vi "OP_Print_TPS_cluster_20180209_v2013last.vi"() -> ()   [LabVIEW 2017]
uses:
  <vilib>/addons/database/Connection.llb/DB Tools Open Connec (Path).vi
  <vilib>/addons/database/Connection.llb/Conn Execute.vi
  <vilib>/addons/database/Recordset.llb/Rec Fetch Recordset Data (R).vi
  <vilib>/addons/database/Recordset.llb/Rec Destroy - Connection.vi
  <userlib>/caLab/Private/Get_PV-1D.vi
  <userlib>/caLab/Private/Get_PV.vi
  <vilib>/Utility/file.llb/Write To Spreadsheet File (string).vi
  <vilib>/addons/database/NI_Database_API.lvlib
panel:
  out "error out 2":errorcluster
  in  "WindowsMediaPlayer":refnum<k7>(container)
  in  "Vol.":i32(slide)=12 min=0 max=100 step=1 scale=0.0..100.0
  out "index":i32
  in  "Play Button":bool
  in  "Skip Forward Button":bool
  in  "Skip Back Button":bool
  in  "Pause Button":bool
  out "appended path":path=path "C:/Users/TPSOP/Desktop/新增資料夾 (2)/musics/1.mp3"
  out "status":string="就緒"
  out "error out":errorcluster
  out "new picture":picture
  in  "T:Slow\nF:Fast":bool
  in  "Switch Tab":bool=TRUE
  out "Tab Control":enum32{"_____", "           "}(tab)
  out "Cluster":T1={"SR Fill Pattern"=[], "Beam Current(mA"=320.769453, "Beam Lifetime(min)"=354.3939151043138, "Beamsize X(um)"=63.15189373514937, "Beamsize Y(um)"=38.03691397287648, "Tune X(from BPM)"=0.1487279843444227, "Tune Y(from BPM)"=0.2309197651663405, "Mode"="Top-Up", "NuX(from BBF) "=0.15142063757609414, "NuY(from BBF)"=0.22496346361412184, "IU22-23gap(R)"=7.0, "IU22-05gap(R)"=7.372, "IU22-05M"=TRUE, "IU22A-09gap(R)"=8.05, "IU22A-09M"=TRUE, "IU22B-09gap(R)"=40.001, "IU22B-09M"=FALSE, "IUT22-21gap(R)"=7.0, "IUT22-21M"=TRUE, "IU22-23M"=TRUE, "IU22A-25gap(R)"=7.0, "IU22A-25M"=TRUE, "IU22B-25gap(R)"=40.0, "IU22B-25M"=FALSE, "EPU48A-41gap(R)"=65.00055, "EPU48A-41gM"=FALSE, "EPU48B-41gap(R)"=27.450000000000003, "EPU48B-41gM"=TRUE, "EPU46-45gap(R)"=44.99850000000001, "EPU46-45gM"=FALSE, "EPU48A-41phase(R)"=0.00055, "EPU48B-41phase(R)"=0.0, "EPU46-45phase(R)"=5e-05, "Grid volt.(V)[S]"=33.0, "Gun mode"="MBM", "Mod.3 HV(kV)[S]"=35.37999999999996, "SR"="SR_DMB_2017_1024_0300LOCO.data", "BR"="Booster_2017_1023_0900.data", "LI"="Linac_2017_0413_1015.data", "LTB"="LTB_JT_2017_0828_1050.data", "BTS"="BTS_2017_1023_0900.data", "RF2 remote"=TRUE, "RF2 OP mode"=TRUE, "RF2 phase.[S]"=-42.0, "RF Freq.(s)"=499655365.67399085, "RF2 gap volt[S]"=1600.0, "RF3 remote"=TRUE, "RF3 OP mode"=TRUE, "RF3 phase.[S]"=1.1999999999999995, "RF3 gap volt.[S]"=1600.0, "BBF V"=TRUE, "BBF H"=TRUE, "BR ext. kicker1(kV)"=17.666, "BR ext. kicker2(kV)"=17.666, "BR ext. sep.1(V)"=322.14, "BR ext. sep.2(V)"=441.1, "BR inj. sep.(V)"=104.95, "BR inj. kicker(kV)"=13.449999999999969, "SR kicker4(kV)"=7.945, "SR kicker3(kV)"=8.02, "SR kicker2(kV)"=8.142, "SR kicker1(kV)"=8.1, "SR inj. sep.2(V)"=397.2, "SR inj. sep.1(V)"=398.04, "Bucket Start"=100.0, "Bucket Last"=450.0, "Bucket Step"=10.0, "Orbit ILK(P)"=TRUE, "IU22-05 Hutch Enable"=TRUE, "IU22A-09M Hutch Enable"=TRUE, "IUT22-21M Hutch Enable"=TRUE, "IU22-23M Hutch Enable"=TRUE, "IU22A-25M Hutch Enable"=TRUE, "EPU48A-41M Hutch Enable"=TRUE, "EPU46-45M Hutch Enable"=FALSE, "EPU46-45 FE Enable"=TRUE, "EPU48A-41 FE Enable"=TRUE, "IU22A-25 FE Enable"=TRUE, "IU22-23 FE Enable"=TRUE, "IUT22-21 FE Enable"=TRUE, "IU22A-09 FE Enable"=TRUE, "IU22-05 FE Enable"=TRUE, "EPU48A-41pM"=FALSE, "EPU48B-41pM"=TRUE, "EPU46-45pM"=FALSE, "Gun volt.(V)[S]"=23.5, "Width count"=75.0, "2ns step"=2.0, "10ps delay"=150.0, "phase shifter"=130.0015, "Taper"=1.0899999999999999, "05XBPMX 1"=14.279, "09XBPMX 1"=-34.837, "21XBPMX 1"=-36.466, "23XBPMX 1"=-38.547000000000004, "25XBPMX 1"=-40.08, "41XBPMX 1"=-513.551, "45XBPMX 1"=-12.86, "05XBPMY 1"=51.999, "09XBPMY 1"=30.004, "21XBPMY 1"=-4.771, "23XBPMY 1"=19.080000000000002, "25XBPMY 1"=-4.366, "41XBPMY 1"=309.241, "45XBPMY 1"=1.842, "FOFB H"="On", "FOFB V"="On", "time string"="15:45:09", "date"="2017/10/28", "date (last kicker ON)"="", "time string (last kicker ON)"="", "Radio Buttons 2"=enum."absolute", "09XBPMX 2"="23.77", "09XBPMY 2"="-18.01", "05XBPMY 2"="-459.85", "05XBPMX 2"="-403.56", "21XBPMY 2"="-134.87", "21XBPMX 2"="-31.92", "23XBPMY 2"="233.82", "23XBPMX 2"="11.09", "25XBPMY 2"="5171.53", "25XBPMX 2"="2152.43", "41XBPMY 2"=" closed", "41XBPMX 2"=" PAB ", "45XBPMX 2"=" Hutch ", "45XBPMY 2"=" closed", "05 mode"="Follow", "09A mode"="Follow", "09B mode"="Follow", "21 mode"="Follow", "23 mode"="Follow", "25A mode"="Follow", "25B mode"="Follow", "41A mode"="Follow", "41B mode"="Follow", "46 mode"="Follow", "BeamCurrent History"={"BPM NO.  1_172"=array[4319 elements], array[4319 elements]}, "SR Beam Current in            hours"=12.0, "RF FB"="On", "gap value："=0, "BR Fill Pattern"=[], "time string (last INJ) "="", "BPMX Graph 2"={"Array of X axis  平均分配至各段"=[1.0, 1.1666666666666667, 1.3333333333333333, 1.5, 1.6666666666666665, 1.8333333333333333, 2.0, 2.142857142857143, 2.2857142857142856, 2.4285714285714284, 2.571428571428571, 2.7142857142857144, 2.857142857142857, 3.0, 3.142857142857143, 3.2857142857142856, 3.4285714285714284, 3.571428571428571, 3.7142857142857144, 3.857142857142857, 4.0, 4.125, 4.25, 4.375, 4.5, 4.625, 4.75, 4.875, 5.0, 5.125, 5.25, 5.375, 5.5, 5.625, 5.75, 5.875, 6.0, 6.142857142857143, 6.285714285714286, 6.428571428571429, 6.571428571428571, 6.714285714285714, 6.857142857142857, 7.0, 7.142857142857143, 7.285714285714286, 7.428571428571429, 7.571428571428571, 7.714285714285714, 7.857142857142857, 8.0, 8.142857142857142, 8.285714285714286, 8.428571428571429, 8.571428571428571, 8.714285714285714, 8.857142857142858, 9.0, 9.142857142857142, 9.285714285714286, 9.428571428571429, 9.571428571428571, 9.714285714285714, 9.857142857142858, 10.0, 10.142857142857142, 10.285714285714286, 10.428571428571429, 10.571428571428571, 10.714285714285714, 10.857142857142858, 11.0, 11.142857142857142, 11.285714285714286, 11.428571428571429, 11.571428571428571, 11.714285714285714, 11.857142857142858, 12.0, 12.125, 12.25, 12.375, 12.5, 12.625, 12.75, 12.875, 13.0, 13.125, 13.25, 13.375, 13.5, 13.625, 13.75, 13.875, 14.0, 14.142857142857142, 14.285714285714286, 14.428571428571429, 14.571428571428571, 14.714285714285714, 14.857142857142858, 15.0, 15.142857142857142, 15.285714285714286, 15.428571428571429, 15.571428571428571, 15.714285714285714, 15.857142857142858, 16.0, 16.142857142857142, 16.285714285714285, 16.428571428571427, 16.571428571428573, 16.714285714285715, 16.857142857142858, 17.0, 17.142857142857142, 17.285714285714285, 17.428571428571427, 17.571428571428573, 17.714285714285715, 17.857142857142858, 18.0, 18.142857142857142, 18.285714285714285, 18.428571428571427, 18.571428571428573, 18.714285714285715, 18.857142857142858, 19.0, 19.142857142857142, 19.285714285714285, 19.428571428571427, 19.571428571428573, 19.714285714285715, 19.857142857142858, 20.0, 20.125, 20.25, 20.375, 20.5, 20.625, 20.75, 20.875, 21.0, 21.125, 21.25, 21.375, 21.5, 21.625, 21.75, 21.875, 22.0, 22.142857142857142, 22.285714285714285, 22.428571428571427, 22.571428571428573, 22.714285714285715, 22.857142857142858, 23.0, 23.142857142857142, 23.285714285714285, 23.428571428571427, 23.571428571428573, 23.714285714285715, 23.857142857142858, 24.0, 24.166666666666668, 24.333333333333332, 24.5, 24.666666666666668, 24.833333333333332], [-104.35000000000001, -27.61, -81.269, 31.074, 6.062, -136.0, 99.494, -88.141, -46.889, -165.06900000000002, 6.021, -84.98, 1.75, -8.811, 8.532, -133.949, -96.848, 24.799, 5.059, -100.301, 144.643, -9.353, 21.271, -55.053000000000004, 53.308, 191.175, 158.868, 222.566, -123.501, -26.869, 534.8770000000001, 573.141, -225.076, -6.779, 120.711, -75.419, 85.256, 50.948, -59.4, -203.09900000000002, -20.847, 130.465, -112.508, 76.115, 15.039, -35.207, -105.659, -16.897000000000002, 68.91, -141.159, 107.378, 144.351, -55.053000000000004, -193.076, 129.21, 58.157000000000004, -162.566, 153.643, 28.149, 9.358, -84.211, 85.112, 22.422, -31.252, 89.379, -47.49, 54.793, -68.275, 110.611, -118.584, -371.90500000000003, -20.115000000000002, -329.103, -249.097, -146.817, 118.556, -25.749, -98.32600000000001, 55.269, -122.093, 50.967, -55.89, 88.019, -0.462, -608.1560000000001, -139.752, -304.999, -215.022, 93.23400000000001, 44.699, -65.235, 37.049, -3.491, -169.852, 216.458, 50.398, -92.285, -132.13400000000001, -12.869, 66.74, -188.53300000000002, 148.653, -5.112, -71.334, -177.681, 41.168, -12.532, -184.913, 194.919, 52.414, -75.628, -80.415, -36.814, 105.73100000000001, -104.36800000000001, 110.101, 49.669000000000004, -67.327, -157.372, 29.624000000000002, 22.156, -105.663, 47.799, 11.591000000000001, -75.285, -79.821, 34.331, -24.937, -158.703, 177.15, 200.872, -165.849, -60.67, 20.183, -15.311, -111.206, 107.58800000000001, 26.489, 69.547, -41.230000000000004, 81.986, 54.43, 253.076, 378.43600000000004, -117.003, -304.999, 131.013, 2.21, -158.435, 94.489, 63.017, -82.94500000000001, 99.147, 65.752, -37.261, -102.577, 41.791000000000004, 66.599, -163.73, 160.137, -7.15, -51.275, -140.353, 33.772, 54.203, -147.597, 128.696, 58.22, -47.144, -184.493, 56.980000000000004, 67.437, -54.227000000000004, -0.031]}, "BPMY Graph 2"={"Array of X axis  平均分配至各段"=[1.0, 1.1666666666666667, 1.3333333333333333, 1.5, 1.6666666666666665, 1.8333333333333333, 2.0, 2.142857142857143, 2.2857142857142856, 2.4285714285714284, 2.571428571428571, 2.7142857142857144, 2.857142857142857, 3.0, 3.142857142857143, 3.2857142857142856, 3.4285714285714284, 3.571428571428571, 3.7142857142857144, 3.857142857142857, 4.0, 4.125, 4.25, 4.375, 4.5, 4.625, 4.75, 4.875, 5.0, 5.125, 5.25, 5.375, 5.5, 5.625, 5.75, 5.875, 6.0, 6.142857142857143, 6.285714285714286, 6.428571428571429, 6.571428571428571, 6.714285714285714, 6.857142857142857, 7.0, 7.142857142857143, 7.285714285714286, 7.428571428571429, 7.571428571428571, 7.714285714285714, 7.857142857142857, 8.0, 8.142857142857142, 8.285714285714286, 8.428571428571429, 8.571428571428571, 8.714285714285714, 8.857142857142858, 9.0, 9.142857142857142, 9.285714285714286, 9.428571428571429, 9.571428571428571, 9.714285714285714, 9.857142857142858, 10.0, 10.142857142857142, 10.285714285714286, 10.428571428571429, 10.571428571428571, 10.714285714285714, 10.857142857142858, 11.0, 11.142857142857142, 11.285714285714286, 11.428571428571429, 11.571428571428571, 11.714285714285714, 11.857142857142858, 12.0, 12.125, 12.25, 12.375, 12.5, 12.625, 12.75, 12.875, 13.0, 13.125, 13.25, 13.375, 13.5, 13.625, 13.75, 13.875, 14.0, 14.142857142857142, 14.285714285714286, 14.428571428571429, 14.571428571428571, 14.714285714285714, 14.857142857142858, 15.0, 15.142857142857142, 15.285714285714286, 15.428571428571429, 15.571428571428571, 15.714285714285714, 15.857142857142858, 16.0, 16.142857142857142, 16.285714285714285, 16.428571428571427, 16.571428571428573, 16.714285714285715, 16.857142857142858, 17.0, 17.142857142857142, 17.285714285714285, 17.428571428571427, 17.571428571428573, 17.714285714285715, 17.857142857142858, 18.0, 18.142857142857142, 18.285714285714285, 18.428571428571427, 18.571428571428573, 18.714285714285715, 18.857142857142858, 19.0, 19.142857142857142, 19.285714285714285, 19.428571428571427, 19.571428571428573, 19.714285714285715, 19.857142857142858, 20.0, 20.125, 20.25, 20.375, 20.5, 20.625, 20.75, 20.875, 21.0, 21.125, 21.25, 21.375, 21.5, 21.625, 21.75, 21.875, 22.0, 22.142857142857142, 22.285714285714285, 22.428571428571427, 22.571428571428573, 22.714285714285715, 22.857142857142858, 23.0, 23.142857142857142, 23.285714285714285, 23.428571428571427, 23.571428571428573, 23.714285714285715, 23.857142857142858, 24.0, 24.166666666666668, 24.333333333333332, 24.5, 24.666666666666668, 24.833333333333332], [-143.858, -13.775, -13.785, 122.665, -66.475, 31.541, 2.118, -24.67, 28.275000000000002, 0.139, -36.578, -28.396, 48.925000000000004, 9.287, -3.412, 70.053, -21.479, 14.89, -7.234, 5.521, -3.164, 19.558, -37.538000000000004, 37.11, -77.159, -13.755, 77.63, 28.249000000000002, -209.114, -44.569, 92.851, 173.641, -70.156, -22.722, 17.795, -6.59, 25.654, -41.882, 53.713, 9.237, -26.164, 18.357, 63.695, -8.542, 5.183, -5.99, 9.508000000000001, -5.462, -29.446, 36.574, -52.552, 51.439, -48.502, 0.73, -23.836000000000002, -3.648, -9.628, -5.485, -68.679, 95.486, -62.041000000000004, 54.633, -58.791000000000004, 68.305, -49.682, 29.838, -8.459, 3.213, -5.561, -80.617, 58.144, 15.346, -158.743, -40.726, 5.259, 3.258, 41.128, -54.377, 5.01, 18.84, 11.403, -20.73, 21.792, -17.296, 27.29, 0.783, -6.804, -137.476, 116.70700000000001, -6.929, 17.846, -3.586, 11.754, 6.341, 0.292, -0.911, -8.236, -5.312, 14.939, -29.945, 30.573, -9.991, -49.344, 82.117, -27.45, 22.291, -6.636, -9.389, 10.034, -14.218, 14.215, -7.3, 12.409, -44.302, 50.197, -36.089, -9.120000000000001, 45.881, 14.836, -27.324, 10.765, -10.139, -33.252, 2.737, -9.99, -6.019, -53.329, -28.159, 2.676, -36.9, -2.372, 8.92, 13.599, -25.723, -16.436, 7.722, -0.088, -29.122, 32.814, -20.521, 30.155, -45.734, 36.611000000000004, 74.528, 68.482, -22.548000000000002, -31.398, 134.603, -45.587, -0.981, -40.156, 24.441, 20.477, -31.424, 19.5, -11.789, 16.394000000000002, -38.567, 9.523, 0.09, -0.058, -4.8500000000000005, 11.71, 25.637, -10.51, -18.101, -12.389000000000001, 95.417, -138.726, 30.355, 96.245, -48.666000000000004, 40.851, -0.71]}} {"SR Beam Current in            hours" min=1.0 max=24.0 step=1.0 format="%#_2f"; "45XBPMY 1" format="%#.2f"; "41XBPMY 1" format="%#.2f"; "25XBPMY 1" format="%#.2f"; "23XBPMY 1" format="%#.2f"; "21XBPMY 1" format="%#.2f"; "09XBPMY 1" format="%#.2f"; "05XBPMY 1" format="%#.2f"; "45XBPMX 1" format="%#.2f"; "41XBPMX 1" format="%#.2f"; "25XBPMX 1" format="%#.2f"; "23XBPMX 1" format="%#.2f"; "21XBPMX 1" format="%#.2f"; "09XBPMX 1" format="%#.2f"; "05XBPMX 1" format="%#.2f"; "Taper" format="%#.4f"; "phase shifter" format="%#.3f"; "10ps delay" format="%#.1f"; "2ns step" format="%#.1f"; "Width count" format="%#.1f"; "Gun volt.(V)[S]" format="%#.1f"; "Bucket Step" format="%#.2f"; "Bucket Last" format="%#.2f"; "Bucket Start" format="%#.2f"; "BR ext. kicker1(kV)" format="%#.2f"; "BR ext. kicker2(kV)" format="%#.2f"; "BR ext. sep.1(V)" format="%#.2f"; "BR ext. sep.2(V)" format="%#.2f"; "BR inj. sep.(V)" format="%#.3f"; "BR inj. kicker(kV)" format="%#.3f"; "SR kicker4(kV)" format="%#.2f"; "SR kicker3(kV)" format="%#.2f"; "SR kicker2(kV)" format="%#.2f"; "SR kicker1(kV)" format="%#.2f"; "SR inj. sep.2(V)" format="%#.2f"; "SR inj. sep.1(V)" format="%#.2f"; "RF3 gap volt.[S]" format="%#.0f"; "RF3 phase.[S]" format="%#.1f"; "RF2 gap volt[S]" format="%#.0f"; "RF Freq.(s)" format="%#.1f"; "RF2 phase.[S]" format="%#.1f"; "Mod.3 HV(kV)[S]" format="%#.3f"; "Grid volt.(V)[S]" format="%#.1f"; "EPU46-45phase(R)" format="%#.4f"; "EPU48B-41phase(R)" format="%#.4f"; "EPU48A-41phase(R)" format="%#.4f"; "EPU46-45gap(R)" format="%#.4f"; "EPU48B-41gap(R)" format="%#.4f"; "EPU48A-41gap(R)" format="%#.4f"; "IU22B-25gap(R)" format="%#.4f"; "IU22A-25gap(R)" format="%#.4f"; "IUT22-21gap(R)" format="%#.4f"; "IU22B-09gap(R)" format="%#.4f"; "IU22A-09gap(R)" format="%#.4f"; "IU22-05gap(R)" format="%#.4f"; "IU22-23gap(R)" format="%#.4f"; "NuY(from BBF)" format="%#.4f"; "NuX(from BBF)" format="%#.4f"; "Tune Y(from BPM)" format="%#.4f"; "Tune X(from BPM)" format="%#.4f"; "Beamsize Y(um)" format="%#.2f"; "Beamsize X(um)" format="%#.2f"; "Beam Lifetime(min)" format="%#.3f"; "Beam Current(mA" format="%#.3f"}
  out "Diff list":string[][](array[string])
  out "EVENTs":i32
  out "check loop":i32
  in  "Check period":i32=10 min=0 max=10
  out "Program Start Time":dbl=3592021508.642459
  out "dT":u32=325
  out "PV list":string[](array[string])=["LI-ES-CPS-01:SETMODE", "LI-ES-CPS-01:PULSEMODE", "LI-ES-BPS-01:SETU:GRID", "LI-ES-BPS-01:SETU:SBM", "LI-ES-BPS-01:SETU:MBM", "LI-RF-CAB-07:SET:MODE", "LI-RF-HVP-11:SET:U", "LI-RF-CAB-09:SET:MODE", "LI-RF-HVP-21:SET:U", "LI-RF-CAB-11:SET:MODE", "LI-RF-HVP-31:SET:U", "LI-RF-WGA-01:SET:POS", "LI-RF-WGA-02:SET:POS", "LI-RF-WGA-03:SET:POS", "LI-RF-SFT-01:SET:POS", "LI-RF-SFT-02:SET:POS", "LI-RF-SFT-03:SET:POS", "LI-RF-CTR-01:ES:SET:DEG", "LI-RF-CTR-01:SP:SET:DEG", "LI-RF-CTR-01:K123:SET:DEG", "LI-RF-CTR-01:K1:SET:DEG", "LI-RF-CTR-01:K3:SET:DEG", "LI-RF-AMP-01:SET:PWR", "LI-RF-AMP-02:SET:PWR", "LI-MA-SPS-01:SET:I", "LI-MA-SPS-02:SET:I", "LI-MA-SPS-03:SET:I", "LI-MA-SPS-04:SET:I", "LI-MA-SPS-05:SET:I", "LI-MA-SPS-06:SET:I", "LI-MA-SPS-07:SET:I", "LI-MA-SPS-08:SET:I", "LI-MA-SPS-09:SET:I", "LI-MA-SPS-10:SET:I", "LI-MA-SPS-11:SET:I", "LI-MA-SPS-12:SET:I", "LI-MA-SPS-13:SET:I", "LI-MA-SPS-14:SET:I", "LI-MA-SPS-15:SET:I", "LI-MA-SPS-16:SET:I", "LI-MA-STP-01:SET:I", "LI-MA-STP-02:SET:I", "LI-MA-STP-03:SET:I", "LI-MA-STP-04:SET:I", "LI-MA-STP-05:SET:I", "LI-MA-STP-06:SET:I", "LI-MA-STP-07:SET:I", "LI-MA-STP-08:SET:I", "LI-MA-STP-09:SET:I", "LI-MA-STP-10:SET:I", "LI-MA-STP-11:SET:I", "LI-MA-STP-12:SET:I", "LI-MA-STP-13:SET:I", "LI-MA-STP-14:SET:I", "LI-MA-STP-15:SET:I", "LI-MA-STP-16:SET:I", "LI-MA-QPS-01:SET:I", "LI-MA-QPS-02:SET:I", "LI-MA-QPS-03:SET:I", "LI-MA-QPS-04:SET:I", "LI-MA-QPS-05:SET:I", "LI-MA-QPS-06:SET:I", "CPCITM-TI-EVRTG:Pulse7DelaySet", "CPCITM-TI-EVRTG:Pulse7WidthSet", "CPCITM-TI-EVRTG:GTX7CtrlGTXPHSet", "CPCITM-TI-EVRTG:GTX7DlySet", "CPCITM-TI-EVRTG:Pulse6DelaySet", "CPCITM-TI-EVRTG:Pulse6WidthSet", "CPCITM-TI-EVRTG:GTX6CtrlGTXPHSet", "CPCITM-TI-EVRTG:GTX6DlySet", "CPCILI-TI-EVR:Pulse2DelaySet", "CPCILI-TI-EVR:Pulse2WidthSet", "CPCILI-TI-EVR:Pulse3DelaySet", "CPCILI-TI-EVR:Pulse3WidthSet", "CPCILI-TI-EVR:Pulse4DelaySet", "CPCILI-TI-EVR:Pulse4WidthSet", "CPCILI-TI-EVR:Pulse5DelaySet", "CPCILI-TI-EVR:Pulse5WidthSet", "CPCILI-TI-EVR:Pulse6DelaySet", "CPCILI-TI-EVR:Pulse6WidthSet", "CPCILI-TI-EVR:Pulse7DelaySet", "CPCILI-TI-EVR:Pulse7WidthSet", "CPCILI-TI-EVR:Pulse8DelaySet", "CPCILI-TI-EVR:Pulse8WidthSet", "CPCILI-TI-EVR:Pulse9DelaySet", "CPCILI-TI-EVR:Pulse9WidthSet", "CPCITM-TI-EVRTG:GTX6DlySet", "CPCITM-TI-EVRTG:GTX7DlySet", "LTB-PS-HC-1:setI", "LTB-PS-HC-2:setI", "LTB-PS-HC-3:setI", "LTB-PS-HC-4:setI", "LTB-PS-HC-5:setI", "LTB-PS-VC-1:setI", "LTB-PS-VC-2:setI", "LTB-PS-VC-3:setI", "LTB-PS-VC-4:setI", "LTB-PS-VC-5:setI", "LTB-PS-VC-6:setI", "LTB-PS-VC-7:setI", "LTB-PS-Q1A:setI", "LTB-PS-Q1B:setI", "LTB-PS-Q1C:setI", "LTB-PS-Q2A:setI", "LTB-PS-Q2B:setI", "LTB-PS-Q2C:setI", "LTB-PS-Q3A:setI", "LTB-PS-Q3B:setI", "LTB-PS-Q4A:setI", "LTB-PS-Q4B:setI", "LTB-PS-QQ:setI", "LTB-PS-BEND-1:setI", "LTB-PS-VC-2a:setI", "LTB-PS-HC-3a:setI", "LTB-PS-HC-3b:setI", "LTB-PS-HC-4a:setI", "LTB-PS-HC-5a:setI", "LI-DI-SLIT-motor:axis2Position1", "LI-DI-SLIT-motor:axis1Position1", "BR-PS-HC-101:setI", "BR-PS-HC-102:setI", "BR-PS-HC-103:setI", "BR-PS-HC-104:setI", "BR-PS-HC-105:setI", "BR-PS-HC-106:setI", "BR-PS-HC-107:setI", "BR-PS-HC-108:setI", "BR-PS-HC-109:setI", "BR-PS-HC-110:setI", "BR-PS-HC-201:setI", "BR-PS-HC-202:setI", "BR-PS-HC-203:setI", "BR-PS-HC-204:setI", "BR-PS-HC-205:setI", "BR-PS-HC-206:setI", "BR-PS-HC-207:setI", "BR-PS-HC-208:setI", "BR-PS-HC-209:setI", "BR-PS-HC-210:setI", "BR-PS-HC-301:setI", "BR-PS-HC-302:setI", "BR-PS-HC-303:setI", "BR-PS-HC-304:setI", "BR-PS-HC-305:setI", "BR-PS-HC-306:setI", "BR-PS-HC-307:setI", "BR-PS-HC-308:setI", "BR-PS-HC-309:setI", "BR-PS-HC-310:setI", "BR-PS-HC-401:setI", "BR-PS-HC-402:setI", "BR-PS-HC-403:setI", "BR-PS-HC-404:setI", "BR-PS-HC-405:setI", "BR-PS-HC-406:setI", "BR-PS-HC-407:setI", "BR-PS-HC-408:setI", "BR-PS-HC-409:setI", "BR-PS-HC-410:setI", "BR-PS-HC-501:setI", "BR-PS-HC-502:setI", "BR-PS-HC-503:setI", "BR-PS-HC-504:setI", "BR-PS-HC-505:setI", "BR-PS-HC-506:setI", "BR-PS-HC-507:setI", "BR-PS-HC-508:setI", "BR-PS-HC-509:setI", "BR-PS-HC-510:setI", "BR-PS-HC-601:setI", "BR-PS-HC-602:setI", "BR-PS-HC-603:setI", "BR-PS-HC-603a:setI", "BR-PS-HC-604:setI", "BR-PS-HC-605:setI", "BR-PS-HC-606:setI", "BR-PS-HC-606a:setI", "BR-PS-HC-607:setI", "BR-PS-HC-608:setI", "BR-PS-HC-609:setI", "BR-PS-HC-610:setI", "BR-PS-VC-101:setI", "BR-PS-VC-102:setI", "BR-PS-VC-103:setI", "BR-PS-VC-104:setI", "BR-PS-VC-105:setI", "BR-PS-VC-106:setI", "BR-PS-VC-201:setI", "BR-PS-VC-202:setI", "BR-PS-VC-203:setI", "BR-PS-VC-204:setI", "BR-PS-VC-205:setI", "BR-PS-VC-206:setI", "BR-PS-VC-301:setI", "BR-PS-VC-302:setI", "BR-PS-VC-303:setI", "BR-PS-VC-304:setI", "BR-PS-VC-305:setI", "BR-PS-VC-306:setI", "BR-PS-VC-401:setI", "BR-PS-VC-402:setI", "BR-PS-VC-403:setI", "BR-PS-VC-404:setI", "BR-PS-VC-405:setI", "BR-PS-VC-406:setI", "BR-PS-VC-501:setI", "BR-PS-VC-502:setI", "BR-PS-VC-503:setI", "BR-PS-VC-504:setI", "BR-PS-VC-505:setI", "BR-PS-VC-506:setI", "BR-PS-VC-601:setI", "BR-PS-VC-602:setI", "BR-PS-VC-602a:setI", "BR-PS-VC-603:setI", "BR-PS-VC-604:setI", "BR-PS-VC-604a:setI", "BR-PS-VC-605:setI", "BR-PS-VC-606:setI", "BR-PS-VC-100a:setI", "BR-PS-SD:setI", "BR-PS-SF:setI", "cpsc_027:AO:SLOW_SET:CH:1", "cpsc_037:AO:SLOW_SET:CH:3", "BR-RF-LLRF:setStationPhase", "TI-INJ-PROC:setTinj", "BR-PS-INJ-SE:setHV", "CPCIPM-TI-EVR:Pulse1DelaySet", "BR-PS-INJ-KI:setHV", "CPCIPM-TI-EVR:Pulse2DelaySet", "BR-PS-QF:setWfDC", "BR-PS-QM:setWfDC", "BR-PS-Q1:setWfDC", "BR-PS-Q2:setWfDC", "BR-PS-BEND:setWfDC", "BTS-PS-HC-1:setI", "BTS-PS-HC-2:setI", "BTS-PS-HC-3:setI", "BTS-PS-HC-4:setI", "BTS-PS-HC-5:setI", "BTS-PS-VC-2:setI", "BTS-PS-VC-3:setI", "BTS-PS-VC-4:setI", "BTS-PS-VC-5:setI", "BTS-PS-VC-6:setI", "BTS-PS-Q1A:setI", "BTS-PS-Q1B:setI", "BTS-PS-Q1C:setI", "BTS-PS-Q2A:setI", "BTS-PS-Q2B:setI", "BTS-PS-Q2C:setI", "BTS-PS-Q3A:setI", "BTS-PS-BEND-1:setI", "BTS-PS-BEND-2:setI", "BR-PS-EXT-K1:setHV", "BR-PS-EXT-K2:setHV", "SR-PS-INJ-SE1:setHV", "SR-PS-INJ-SE2:setHV", "SR-PS-INJ-K1:setHV", "SR-PS-INJ-K2:setHV", "SR-PS-INJ-K3:setHV", "SR-PS-INJ-K4:setHV", "CPCIPM-TI-EVR:Pulse4DelaySet", "CPCIPM-TI-EVR:Pulse5DelaySet", "CPCIPM-TI-EVR:Pulse3DelaySet", "CPCIPM-TI-EVR:Pulse6DelaySet", "CPCIPM-TI-EVR:Pulse7DelaySet", "T560:setADelay", "T560:setBDelay", "T560:setCDelay", "T560:setDDelay", "CPCIPM-TI-EVR:Pulse4DelaySet", "CPCIPM-TI-EVR:Pulse5DelaySet", "BR-PS-EXT-SE1:setHV", "BR-PS-EXT-SE2:setHV", "CPCIPM-TI-EVR:Pulse3DelaySet", "CPCIPM-TI-EVR:Pulse11DelaySet", "SR-PS-BEND:setI", "SR-PS-HC-011:setI", "SR-PS-HC-012:setI", "SR-PS-HC-013:setI", "SR-PS-HC-014:setI", "SR-PS-HC-015:setI", "SR-PS-HC-016:setI", "SR-PS-HC-017:setI", "SR-PS-HC-021:setI", "SR-PS-HC-022:setI", "SR-PS-HC-023:setI", "SR-PS-HC-024:setI", "SR-PS-HC-025:setI", "SR-PS-HC-026:setI", "SR-PS-HC-027:setI", "SR-PS-HC-031:setI", "SR-PS-HC-032:setI", "SR-PS-HC-033:setI", "SR-PS-HC-034:setI", "SR-PS-HC-035:setI", "SR-PS-HC-036:setI", "SR-PS-HC-037:setI", "SR-PS-HC-041:setI", "SR-PS-HC-042:setI", "SR-PS-HC-043:setI", "SR-PS-HC-044:setI", "SR-PS-HC-045:setI", "SR-PS-HC-046:setI", "SR-PS-HC-047:setI", "SR-PS-HC-051:setI", "SR-PS-HC-052:setI", "SR-PS-HC-053:setI", "SR-PS-HC-054:setI", "SR-PS-HC-055:setI", "SR-PS-HC-056:setI", "SR-PS-HC-057:setI", "SR-PS-HC-061:setI", "SR-PS-HC-062:setI", "SR-PS-HC-063:setI", "SR-PS-HC-064:setI", "SR-PS-HC-065:setI", "SR-PS-HC-066:setI", "SR-PS-HC-067:setI", "SR-PS-HC-071:setI", "SR-PS-HC-072:setI", "SR-PS-HC-073:setI", "SR-PS-HC-074:setI", "SR-PS-HC-075:setI", "SR-PS-HC-076:setI", "SR-PS-HC-077:setI", "SR-PS-HC-081:setI", "SR-PS-HC-082:setI", "SR-PS-HC-083:setI", "SR-PS-HC-084:setI", "SR-PS-HC-085:setI", "SR-PS-HC-086:setI", "SR-PS-HC-087:setI", "SR-PS-HC-091:setI", "SR-PS-HC-092:setI", "SR-PS-HC-093:setI", "SR-PS-HC-094:setI", "SR-PS-HC-095:setI", "SR-PS-HC-096:setI", "SR-PS-HC-097:setI", "SR-PS-HC-101:setI", "SR-PS-HC-102:setI", "SR-PS-HC-103:setI", "SR-PS-HC-104:setI", "SR-PS-HC-105:setI", "SR-PS-HC-106:setI", "SR-PS-HC-107:setI", "SR-PS-HC-111:setI", "SR-PS-HC-112:setI", "SR-PS-HC-113:setI", "SR-PS-HC-114:setI", "SR-PS-HC-115:setI", "SR-PS-HC-116:setI", "SR-PS-HC-117:setI", "SR-PS-HC-121:setI", "SR-PS-HC-122:setI", "SR-PS-HC-123:setI", "SR-PS-HC-124:setI", "SR-PS-HC-125:setI", "SR-PS-HC-126:setI", "SR-PS-HC-127:setI", "SR-PS-HC-131:setI", "SR-PS-HC-132:setI", "SR-PS-HC-133:setI", "SR-PS-HC-134:setI", "SR-PS-HC-135:setI", "SR-PS-HC-136:setI", "SR-PS-HC-137:setI", "SR-PS-HC-141:setI", "SR-PS-HC-142:setI", "SR-PS-HC-143:setI", "SR-PS-HC-144:setI", "SR-PS-HC-145:setI", "SR-PS-HC-146:setI", "SR-PS-HC-147:setI", "SR-PS-HC-151:setI", "SR-PS-HC-152:setI", "SR-PS-HC-153:setI", "SR-PS-HC-154:setI", "SR-PS-HC-155:setI", "SR-PS-HC-156:setI", "SR-PS-HC-157:setI", "SR-PS-HC-161:setI", "SR-PS-HC-162:setI", "SR-PS-HC-163:setI", "SR-PS-HC-164:setI", "SR-PS-HC-165:setI", "SR-PS-HC-166:setI", "SR-PS-HC-167:setI", "SR-PS-HC-171:setI", "SR-PS-HC-172:setI", "SR-PS-HC-173:setI", "SR-PS-HC-174:setI", "SR-PS-HC-175:setI", "SR-PS-HC-176:setI", "SR-PS-HC-177:setI", "SR-PS-HC-181:setI", "SR-PS-HC-182:setI", "SR-PS-HC-183:setI", "SR-PS-HC-184:setI", "SR-PS-HC-185:setI", "SR-PS-HC-186:setI", "SR-PS-HC-187:setI", "SR-PS-HC-191:setI", "SR-PS-HC-192:setI", "SR-PS-HC-193:setI", "SR-PS-HC-194:setI", "SR-PS-HC-195:setI", "SR-PS-HC-196:setI", "SR-PS-HC-197:setI", "SR-PS-HC-201:setI", "SR-PS-HC-202:setI", "SR-PS-HC-203:setI", "SR-PS-HC-204:setI", "SR-PS-HC-205:setI", "SR-PS-HC-206:setI", "SR-PS-HC-207:setI", "SR-PS-HC-211:setI", "SR-PS-HC-212:setI", "SR-PS-HC-213:setI", "SR-PS-HC-214:setI", "SR-PS-HC-215:setI", "SR-PS-HC-216:setI", "SR-PS-HC-217:setI", "SR-PS-HC-221:setI", "SR-PS-HC-222:setI", "SR-PS-HC-223:setI", "SR-PS-HC-224:setI", "SR-PS-HC-225:setI", "SR-PS-HC-226:setI", "SR-PS-HC-227:setI", "SR-PS-HC-231:setI", "SR-PS-HC-232:setI", "SR-PS-HC-233:setI", "SR-PS-HC-234:setI", "SR-PS-HC-235:setI", "SR-PS-HC-236:setI", "SR-PS-HC-237:setI", "SR-PS-HC-241:setI", "SR-PS-HC-242:setI", "SR-PS-HC-243:setI", "SR-PS-HC-244:setI", "SR-PS-HC-245:setI", "SR-PS-HC-246:setI", "SR-PS-HC-247:setI", "SR-PS-VC-011:setI", "SR-PS-VC-012:setI", "SR-PS-VC-013:setI", "SR-PS-VC-014:setI", "SR-PS-VC-015:setI", "SR-PS-VC-016:setI", "SR-PS-VC-017:setI", "SR-PS-VC-021:setI", "SR-PS-VC-022:setI", "SR-PS-VC-023:setI", "SR-PS-VC-024:setI", "SR-PS-VC-025:setI", "SR-PS-VC-026:setI", "SR-PS-VC-027:setI", "SR-PS-VC-031:setI", "SR-PS-VC-032:setI", "SR-PS-VC-033:setI", "SR-PS-VC-034:setI", "SR-PS-VC-035:setI", "SR-PS-VC-036:setI", "SR-PS-VC-037:setI", "SR-PS-VC-041:setI", "SR-PS-VC-042:setI", "SR-PS-VC-043:setI", "SR-PS-VC-044:setI", "SR-PS-VC-045:setI", "SR-PS-VC-046:setI", "SR-PS-VC-047:setI", "SR-PS-VC-051:setI", "SR-PS-VC-052:setI", "SR-PS-VC-053:setI", "SR-PS-VC-054:setI", "SR-PS-VC-055:setI", "SR-PS-VC-056:setI", "SR-PS-VC-057:setI", "SR-PS-VC-061:setI", "SR-PS-VC-062:setI", "SR-PS-VC-063:setI", "SR-PS-VC-064:setI", "SR-PS-VC-065:setI", "SR-PS-VC-066:setI", "SR-PS-VC-067:setI", "SR-PS-VC-071:setI", "SR-PS-VC-072:setI", "SR-PS-VC-073:setI", "SR-PS-VC-074:setI", "SR-PS-VC-075:setI", "SR-PS-VC-076:setI", "SR-PS-VC-077:setI", "SR-PS-VC-081:setI", "SR-PS-VC-082:setI", "SR-PS-VC-083:setI", "SR-PS-VC-084:setI", "SR-PS-VC-085:setI", "SR-PS-VC-086:setI", "SR-PS-VC-087:setI", "SR-PS-VC-091:setI", "SR-PS-VC-092:setI", "SR-PS-VC-093:setI", "SR-PS-VC-094:setI", "SR-PS-VC-095:setI", "SR-PS-VC-096:setI", "SR-PS-VC-097:setI", "SR-PS-VC-101:setI", "SR-PS-VC-102:setI", "SR-PS-VC-103:setI", "SR-PS-VC-104:setI", "SR-PS-VC-105:setI", "SR-PS-VC-106:setI", "SR-PS-VC-107:setI", "SR-PS-VC-111:setI", "SR-PS-VC-112:setI", "SR-PS-VC-113:setI", "SR-PS-VC-114:setI", "SR-PS-VC-115:setI", "SR-PS-VC-116:setI", "SR-PS-VC-117:setI", "SR-PS-VC-121:setI", "SR-PS-VC-122:setI", "SR-PS-VC-123:setI", "SR-PS-VC-124:setI", "SR-PS-VC-125:setI", "SR-PS-VC-126:setI", "SR-PS-VC-127:setI", "SR-PS-VC-131:setI", "SR-PS-VC-132:setI", "SR-PS-VC-133:setI", "SR-PS-VC-134:setI", "SR-PS-VC-135:setI", "SR-PS-VC-136:setI", "SR-PS-VC-137:setI", "SR-PS-VC-141:setI", "SR-PS-VC-142:setI", "SR-PS-VC-143:setI", "SR-PS-VC-144:setI", "SR-PS-VC-145:setI", "SR-PS-VC-146:setI", "SR-PS-VC-147:setI", "SR-PS-VC-151:setI", "SR-PS-VC-152:setI", "SR-PS-VC-153:setI", "SR-PS-VC-154:setI", "SR-PS-VC-155:setI", "SR-PS-VC-156:setI", "SR-PS-VC-157:setI", "SR-PS-VC-161:setI", "SR-PS-VC-162:setI", "SR-PS-VC-163:setI", "SR-PS-VC-164:setI", "SR-PS-VC-165:setI", "SR-PS-VC-166:setI", "SR-PS-VC-167:setI", "SR-PS-VC-171:setI", "SR-PS-VC-172:setI", "SR-PS-VC-173:setI", "SR-PS-VC-174:setI", "SR-PS-VC-175:setI", "SR-PS-VC-176:setI", "SR-PS-VC-177:setI", "SR-PS-VC-181:setI", "SR-PS-VC-182:setI", "SR-PS-VC-183:setI", "SR-PS-VC-184:setI", "SR-PS-VC-185:setI", "SR-PS-VC-186:setI", "SR-PS-VC-187:setI", "SR-PS-VC-191:setI", "SR-PS-VC-192:setI", "SR-PS-VC-193:setI", "SR-PS-VC-194:setI", "SR-PS-VC-195:setI", "SR-PS-VC-196:setI", "SR-PS-VC-197:setI", "SR-PS-VC-201:setI", "SR-PS-VC-202:setI", "SR-PS-VC-203:setI", "SR-PS-VC-204:setI", "SR-PS-VC-205:setI", "SR-PS-VC-206:setI", "SR-PS-VC-207:setI", "SR-PS-VC-211:setI", "SR-PS-VC-212:setI", "SR-PS-VC-213:setI", "SR-PS-VC-214:setI", "SR-PS-VC-215:setI", "SR-PS-VC-216:setI", "SR-PS-VC-217:setI", "SR-PS-VC-221:setI", "SR-PS-VC-222:setI", "SR-PS-VC-223:setI", "SR-PS-VC-224:setI", "SR-PS-VC-225:setI", "SR-PS-VC-226:setI", "SR-PS-VC-227:setI", "SR-PS-VC-231:setI", "SR-PS-VC-232:setI", "SR-PS-VC-233:setI", "SR-PS-VC-234:setI", "SR-PS-VC-235:setI", "SR-PS-VC-236:setI", "SR-PS-VC-237:setI", "SR-PS-VC-241:setI", "SR-PS-VC-242:setI", "SR-PS-VC-243:setI", "SR-PS-VC-244:setI", "SR-PS-VC-245:setI", "SR-PS-VC-246:setI", "SR-PS-VC-247:setI", "SR-PS-QL1-0101:setI", "SR-PS-QL2-0102:setI", "SR-PS-QL3-0103:setI", "SR-PS-QS4-0104:setI", "SR-PS-QS5-0105:setI", "SR-PS-QS5-0106:setI", "SR-PS-QS4-0107:setI", "SR-PS-QS3-0108:setI", "SR-PS-QS2-0109:setI", "SR-PS-QS1-0110:setI", "SR-PS-QS1-0201:setI", "SR-PS-QS2-0202:setI", "SR-PS-QS3-0203:setI", "SR-PS-QS4-0204:setI", "SR-PS-QS5-0205:setI", "SR-PS-QS5-0206:setI", "SR-PS-QS4-0207:setI", "SR-PS-QS3-0208:setI", "SR-PS-QS2-0209:setI", "SR-PS-QS1-0210:setI", "SR-PS-QS1-0301:setI", "SR-PS-QS2-0302:setI", "SR-PS-QS3-0303:setI", "SR-PS-QS4-0304:setI", "SR-PS-QS5-0305:setI", "SR-PS-QS5-0306:setI", "SR-PS-QS4-0307:setI", "SR-PS-QS3-0308:setI", "SR-PS-QS2-0309:setI", "SR-PS-QS1-0310:setI", "SR-PS-QS1-0401:setI", "SR-PS-QS2-0402:setI", "SR-PS-QS3-0403:setI", "SR-PS-QS4-0404:setI", "SR-PS-QS5-0405:setI", "SR-PS-QS5-0406:setI", "SR-PS-QS4-0407:setI", "SR-PS-QL3-0408:setI", "SR-PS-QL2-0409:setI", "SR-PS-QL1-0410:setI", "SR-PS-QL1-0501:setI", "SR-PS-QL2-0502:setI", "SR-PS-QL3-0503:setI", "SR-PS-QS4-0504:setI", "SR-PS-QS5-0505:setI", "SR-PS-QS5-0506:setI", "SR-PS-QS4-0507:setI", "SR-PS-QS3-0508:setI", "SR-PS-QS2-0509:setI", "SR-PS-QS1-0510:setI", "SR-PS-QS1-0601:setI", "SR-PS-QS2-0602:setI", "SR-PS-QS3-0603:setI", "SR-PS-QS4-0604:setI", "SR-PS-QS5-0605:setI", "SR-PS-QS5-0606:setI", "SR-PS-QS4-0607:setI", "SR-PS-QS3-0608:setI", "SR-PS-QS2-0609:setI", "SR-PS-QS1-0610:setI", "SR-PS-QS1-0701:setI", "SR-PS-QS2-0702:setI", "SR-PS-QS3-0703:setI", "SR-PS-QS4-0704:setI", "SR-PS-QS5-0705:setI", "SR-PS-QS5-0706:setI", "SR-PS-QS4-0707:setI", "SR-PS-QS3-0708:setI", "SR-PS-QS2-0709:setI", "SR-PS-QS1-0710:setI", "SR-PS-QS1-0801:setI", "SR-PS-QS2-0802:setI", "SR-PS-QS3-0803:setI", "SR-PS-QS4-0804:setI", "SR-PS-QS5-0805:setI", "SR-PS-QS5-0806:setI", "SR-PS-QS4-0807:setI", "SR-PS-QL3-0808:setI", "SR-PS-QL2-0809:setI", "SR-PS-QL1-0810:setI", "SR-PS-QL1-0901:setI", "SR-PS-QL2-0902:setI", "SR-PS-QL3-0903:setI", "SR-PS-QS4-0904:setI", "SR-PS-QS5-0905:setI", "SR-PS-QS5-0906:setI", "SR-PS-QS4-0907:setI", "SR-PS-QS3-0908:setI", "SR-PS-QS2-0909:setI", "SR-PS-QS1-0910:setI", "SR-PS-QS1-1001:setI", "SR-PS-QS2-1002:setI", "SR-PS-QS3-1003:setI", "SR-PS-QS4-1004:setI", "SR-PS-QS5-1005:setI", "SR-PS-QS5-1006:setI", "SR-PS-QS4-1007:setI", "SR-PS-QS3-1008:setI", "SR-PS-QS2-1009:setI", "SR-PS-QS1-1010:setI", "SR-PS-QS1-1101:setI", "SR-PS-QS2-1102:setI", "SR-PS-QS3-1103:setI", "SR-PS-QS4-1104:setI", "SR-PS-QS5-1105:setI", "SR-PS-QS5-1106:setI", "SR-PS-QS4-1107:setI", "SR-PS-QS3-1108:setI", "SR-PS-QS2-1109:setI", "SR-PS-QS1-1110:setI", "SR-PS-QS1-1201:setI", "SR-PS-QS2-1202:setI", "SR-PS-QS3-1203:setI", "SR-PS-QS4-1204:setI", "SR-PS-QS5-1205:setI", "SR-PS-QS5-1206:setI", "SR-PS-QS4-1207:setI", "SR-PS-QL3-1208:setI", "SR-PS-QL2-1209:setI", "SR-PS-QL1-1210:setI", "SR-PS-QL1-1301:setI", "SR-PS-QL2-1302:setI", "SR-PS-QL3-1303:setI", "SR-PS-QS4-1304:setI", "SR-PS-QS5-1305:setI", "SR-PS-QS5-1306:setI", "SR-PS-QS4-1307:setI", "SR-PS-QS3-1308:setI", "SR-PS-QS2-1309:setI", "SR-PS-QS1-1310:setI", "SR-PS-QS1-1401:setI", "SR-PS-QS2-1402:setI", "SR-PS-QS3-1403:setI", "SR-PS-QS4-1404:setI", "SR-PS-QS5-1405:setI", "SR-PS-QS5-1406:setI", "SR-PS-QS4-1407:setI", "SR-PS-QS3-1408:setI", "SR-PS-QS2-1409:setI", "SR-PS-QS1-1410:setI", "SR-PS-QS1-1501:setI", "SR-PS-QS2-1502:setI", "SR-PS-QS3-1503:setI", "SR-PS-QS4-1504:setI", "SR-PS-QS5-1505:setI", "SR-PS-QS5-1506:setI", "SR-PS-QS4-1507:setI", "SR-PS-QS3-1508:setI", "SR-PS-QS2-1509:setI", "SR-PS-QS1-1510:setI", "SR-PS-QS1-1601:setI", "SR-PS-QS2-1602:setI", "SR-PS-QS3-1603:setI", "SR-PS-QS4-1604:setI", "SR-PS-QS5-1605:setI", "SR-PS-QS5-1606:setI", "SR-PS-QS4-1607:setI", "SR-PS-QL3-1608:setI", "SR-PS-QL2-1609:setI", "SR-PS-QL1-1610:setI", "SR-PS-QL1-1701:setI", "SR-PS-QL2-1702:setI", "SR-PS-QL3-1703:setI", "SR-PS-QS4-1704:setI", "SR-PS-QS5-1705:setI", "SR-PS-QS5-1706:setI", "SR-PS-QS4-1707:setI", "SR-PS-QS3-1708:setI", "SR-PS-QS2-1709:setI", "SR-PS-QS1-1710:setI", "SR-PS-QS1-1801:setI", "SR-PS-QS2-1802:setI", "SR-PS-QS3-1803:setI", "SR-PS-QS4-1804:setI", "SR-PS-QS5-1805:setI", "SR-PS-QS5-1806:setI", "SR-PS-QS4-1807:setI", "SR-PS-QS3-1808:setI", "SR-PS-QS2-1809:setI", "SR-PS-QS1-1810:setI", "SR-PS-QS1-1901:setI", "SR-PS-QS2-1902:setI", "SR-PS-QS3-1903:setI", "SR-PS-QS4-1904:setI", "SR-PS-QS5-1905:setI", "SR-PS-QS5-1906:setI", "SR-PS-QS4-1907:setI", "SR-PS-QS3-1908:setI", "SR-PS-QS2-1909:setI", "SR-PS-QS1-1910:setI", "SR-PS-QS1-2001:setI", "SR-PS-QS2-2002:setI", "SR-PS-QS3-2003:setI", "SR-PS-QS4-2004:setI", "SR-PS-QS5-2005:setI", "SR-PS-QS5-2006:setI", "SR-PS-QS4-2007:setI", "SR-PS-QL3-2008:setI", "SR-PS-QL2-2009:setI", "SR-PS-QL1-2010:setI", "SR-PS-QL1-2101:setI", "SR-PS-QL2-2102:setI", "SR-PS-QL3-2103:setI", "SR-PS-QS4-2104:setI", "SR-PS-QS5-2105:setI", "SR-PS-QS5-2106:setI", "SR-PS-QS4-2107:setI", "SR-PS-QS3-2108:setI", "SR-PS-QS2-2109:setI", "SR-PS-QS1-2110:setI", "SR-PS-QS1-2201:setI", "SR-PS-QS2-2202:setI", "SR-PS-QS3-2203:setI", "SR-PS-QS4-2204:setI", "SR-PS-QS5-2205:setI", "SR-PS-QS5-2206:setI", "SR-PS-QS4-2207:setI", "SR-PS-QS3-2208:setI", "SR-PS-QS2-2209:setI", "SR-PS-QS1-2210:setI", "SR-PS-QS1-2301:setI", "SR-PS-QS2-2302:setI", "SR-PS-QS3-2303:setI", "SR-PS-QS4-2304:setI", "SR-PS-QS5-2305:setI", "SR-PS-QS5-2306:setI", "SR-PS-QS4-2307:setI", "SR-PS-QS3-2308:setI", "SR-PS-QS2-2309:setI", "SR-PS-QS1-2310:setI", "SR-PS-QS1-2401:setI", "SR-PS-QS2-2402:setI", "SR-PS-QS3-2403:setI", "SR-PS-QS4-2404:setI", "SR-PS-QS5-2405:setI", "SR-PS-QS5-2406:setI", "SR-PS-QS4-2407:setI", "SR-PS-QL3-2408:setI", "SR-PS-QL2-2409:setI", "SR-PS-QL1-2410:setI", "SR-PS-S1-011:setI", "SR-PS-S2-012:setI", "SR-PS-SD-013:setI", "SR-PS-SF-014:setI", "SR-PS-SD-015:setI", "SR-PS-S4-016:setI", "SR-PS-S3-017:setI", "SR-PS-S5-021:setI", "SR-PS-S6-022:setI", "SR-PS-SD-023:setI", "SR-PS-SF-024:setI", "SR-PS-SD-025:setI", "SR-PS-S6-026:setI", "SR-PS-S5-027:setI", "SR-PS-S5-031:setI", "SR-PS-S6-032:setI", "SR-PS-SD-033:setI", "SR-PS-SF-034:setI", "SR-PS-SD-035:setI", "SR-PS-S6-036:setI", "SR-PS-S5-037:setI", "SR-PS-S3-041:setI", "SR-PS-S4-042:setI", "SR-PS-SD-043:setI", "SR-PS-SF-044:setI", "SR-PS-SD-045:setI", "SR-PS-S2-046:setI", "SR-PS-S1-047:setI", "SR-PS-S1-051:setI", "SR-PS-S2-052:setI", "SR-PS-SD-053:setI", "SR-PS-SF-054:setI", "SR-PS-SD-055:setI", "SR-PS-S4-056:setI", "SR-PS-S3-057:setI", "SR-PS-S5-061:setI", "SR-PS-S6-062:setI", "SR-PS-SD-063:setI", "SR-PS-SF-064:setI", "SR-PS-SD-065:setI", "SR-PS-S6-066:setI", "SR-PS-S5-067:setI", "SR-PS-S5-071:setI", "SR-PS-S6-072:setI", "SR-PS-SD-073:setI", "SR-PS-SF-074:setI", "SR-PS-SD-075:setI", "SR-PS-S6-076:setI", "SR-PS-S5-077:setI", "SR-PS-S3-081:setI", "SR-PS-S4-082:setI", "SR-PS-SD-083:setI", "SR-PS-SF-084:setI", "SR-PS-SD-085:setI", "SR-PS-S2-086:setI", "SR-PS-S1-087:setI", "SR-PS-S1-091:setI", "SR-PS-S2-092:setI", "SR-PS-SD-093:setI", "SR-PS-SF-094:setI", "SR-PS-SD-095:setI", "SR-PS-S4-096:setI", "SR-PS-S3-097:setI", "SR-PS-S5-101:setI", "SR-PS-S6-102:setI", "SR-PS-SD-103:setI", "SR-PS-SF-104:setI", "SR-PS-SD-105:setI", "SR-PS-S6-106:setI", "SR-PS-S5-107:setI", "SR-PS-S5-111:setI", "SR-PS-S6-112:setI", "SR-PS-SD-113:setI", "SR-PS-SF-114:setI", "SR-PS-SD-115:setI", "SR-PS-S6-116:setI", "SR-PS-S5-117:setI", "SR-PS-S3-121:setI", "SR-PS-S4-122:setI", "SR-PS-SD-123:setI", "SR-PS-SF-124:setI", "SR-PS-SD-125:setI", "SR-PS-S2-126:setI", "SR-PS-S1-127:setI", "SR-PS-S1-131:setI", "SR-PS-S2-132:setI", "SR-PS-SD-133:setI", "SR-PS-SF-134:setI", "SR-PS-SD-135:setI", "SR-PS-S4-136:setI", "SR-PS-S3-137:setI", "SR-PS-S5-141:setI", "SR-PS-S6-142:setI", "SR-PS-SD-143:setI", "SR-PS-SF-144:setI", "SR-PS-SD-145:setI", "SR-PS-S6-146:setI", "SR-PS-S5-147:setI", "SR-PS-S5-151:setI", "SR-PS-S6-152:setI", "SR-PS-SD-153:setI", "SR-PS-SF-154:setI", "SR-PS-SD-155:setI", "SR-PS-S6-156:setI", "SR-PS-S5-157:setI", "SR-PS-S3-161:setI", "SR-PS-S4-162:setI", "SR-PS-SD-163:setI", "SR-PS-SF-164:setI", "SR-PS-SD-165:setI", "SR-PS-S2-166:setI", "SR-PS-S1-167:setI", "SR-PS-S1-171:setI", "SR-PS-S2-172:setI", "SR-PS-SD-173:setI", "SR-PS-SF-174:setI", "SR-PS-SD-175:setI", "SR-PS-S4-176:setI", "SR-PS-S3-177:setI", "SR-PS-S5-181:setI", "SR-PS-S6-182:setI", "SR-PS-SD-183:setI", "SR-PS-SF-184:setI", "SR-PS-SD-185:setI", "SR-PS-S6-186:setI", "SR-PS-S5-187:setI", "SR-PS-S5-191:setI", "SR-PS-S6-192:setI", "SR-PS-SD-193:setI", "SR-PS-SF-194:setI", "SR-PS-SD-195:setI", "SR-PS-S6-196:setI", "SR-PS-S5-197:setI", "SR-PS-S3-201:setI", "SR-PS-S4-202:setI", "SR-PS-SD-203:setI", "SR-PS-SF-204:setI", "SR-PS-SD-205:setI", "SR-PS-S2-206:setI", "SR-PS-S1-207:setI", "SR-PS-S1-211:setI", "SR-PS-S2-212:setI", "SR-PS-SD-213:setI", "SR-PS-SF-214:setI", "SR-PS-SD-215:setI", "SR-PS-S4-216:setI", "SR-PS-S3-217:setI", "SR-PS-S5-221:setI", "SR-PS-S6-222:setI", "SR-PS-SD-223:setI", "SR-PS-SF-224:setI", "SR-PS-SD-225:setI", "SR-PS-S6-226:setI", "SR-PS-S5-227:setI", "SR-PS-S5-231:setI", "SR-PS-S6-232:setI", "SR-PS-SD-233:setI", "SR-PS-SF-234:setI", "SR-PS-SD-235:setI", "SR-PS-S6-236:setI", "SR-PS-S5-237:setI", "SR-PS-S3-241:setI", "SR-PS-S4-242:setI", "SR-PS-SD-243:setI", "SR-PS-SF-244:setI", "SR-PS-SD-245:setI", "SR-PS-S2-246:setI", "SR-PS-S1-247:setI", "SR-PS-SKEW-011:setI", "SR-PS-SKEW-012:setI", "SR-PS-SKEW-013:setI", "SR-PS-SKEW-014:setI", "SR-PS-SKEW-015:setI", "SR-PS-SKEW-016:setI", "SR-PS-SKEW-017:setI", "SR-PS-SKEW-021:setI", "SR-PS-SKEW-022:setI", "SR-PS-SKEW-023:setI", "SR-PS-SKEW-024:setI", "SR-PS-SKEW-025:setI", "SR-PS-SKEW-026:setI", "SR-PS-SKEW-027:setI", "SR-PS-SKEW-031:setI", "SR-PS-SKEW-032:setI", "SR-PS-SKEW-033:setI", "SR-PS-SKEW-034:setI", "SR-PS-SKEW-035:setI", "SR-PS-SKEW-036:setI", "SR-PS-SKEW-037:setI", "SR-PS-SKEW-041:setI", "SR-PS-SKEW-042:setI", "SR-PS-SKEW-043:setI", "SR-PS-SKEW-044:setI", "SR-PS-SKEW-045:setI", "SR-PS-SKEW-046:setI", "SR-PS-SKEW-047:setI", "SR-PS-SKEW-051:setI", "SR-PS-SKEW-052:setI", "SR-PS-SKEW-053:setI", "SR-PS-SKEW-054:setI", "SR-PS-SKEW-055:setI", "SR-PS-SKEW-056:setI", "SR-PS-SKEW-057:setI", "SR-PS-SKEW-061:setI", "SR-PS-SKEW-062:setI", "SR-PS-SKEW-063:setI", "SR-PS-SKEW-064:setI", "SR-PS-SKEW-065:setI", "SR-PS-SKEW-066:setI", "SR-PS-SKEW-067:setI", "SR-PS-SKEW-071:setI", "SR-PS-SKEW-072:setI", "SR-PS-SKEW-073:setI", "SR-PS-SKEW-074:setI", "SR-PS-SKEW-075:setI", "SR-PS-SKEW-076:setI", "SR-PS-SKEW-077:setI", "SR-PS-SKEW-081:setI", "SR-PS-SKEW-082:setI", "SR-PS-SKEW-083:setI", "SR-PS-SKEW-084:setI", "SR-PS-SKEW-085:setI", "SR-PS-SKEW-086:setI", "SR-PS-SKEW-087:setI", "SR-PS-SKEW-091:setI", "SR-PS-SKEW-092:setI", "SR-PS-SKEW-093:setI", "SR-PS-SKEW-094:setI", "SR-PS-SKEW-095:setI", "SR-PS-SKEW-096:setI", "SR-PS-SKEW-097:setI", "SR-PS-SKEW-101:setI", "SR-PS-SKEW-102:setI", "SR-PS-SKEW-103:setI", "SR-PS-SKEW-104:setI", "SR-PS-SKEW-105:setI", "SR-PS-SKEW-106:setI", "SR-PS-SKEW-107:setI", "SR-PS-SKEW-111:setI", "SR-PS-SKEW-112:setI", "SR-PS-SKEW-113:setI", "SR-PS-SKEW-114:setI", "SR-PS-SKEW-115:setI", "SR-PS-SKEW-116:setI", "SR-PS-SKEW-117:setI", "SR-PS-SKEW-121:setI", "SR-PS-SKEW-122:setI", "SR-PS-SKEW-123:setI", "SR-PS-SKEW-124:setI", "SR-PS-SKEW-125:setI", "SR-PS-SKEW-126:setI", "SR-PS-SKEW-127:setI", "SR-PS-SKEW-131:setI", "SR-PS-SKEW-132:setI", "SR-PS-SKEW-133:setI", "SR-PS-SKEW-134:setI", "SR-PS-SKEW-135:setI", "SR-PS-SKEW-136:setI", "SR-PS-SKEW-137:setI", "SR-PS-SKEW-141:setI", "SR-PS-SKEW-142:setI", "SR-PS-SKEW-143:setI", "SR-PS-SKEW-144:setI", "SR-PS-SKEW-145:setI", "SR-PS-SKEW-146:setI", "SR-PS-SKEW-147:setI", "SR-PS-SKEW-151:setI", "SR-PS-SKEW-152:setI", "SR-PS-SKEW-153:setI", "SR-PS-SKEW-154:setI", "SR-PS-SKEW-155:setI", "SR-PS-SKEW-156:setI", "SR-PS-SKEW-157:setI", "SR-PS-SKEW-161:setI", "SR-PS-SKEW-162:setI", "SR-PS-SKEW-163:setI", "SR-PS-SKEW-164:setI", "SR-PS-SKEW-165:setI", "SR-PS-SKEW-166:setI", "SR-PS-SKEW-167:setI", "SR-PS-SKEW-171:setI", "SR-PS-SKEW-172:setI", "SR-PS-SKEW-173:setI", "SR-PS-SKEW-174:setI", "SR-PS-SKEW-175:setI", "SR-PS-SKEW-176:setI", "SR-PS-SKEW-177:setI", "SR-PS-SKEW-181:setI", "SR-PS-SKEW-182:setI", "SR-PS-SKEW-183:setI", "SR-PS-SKEW-184:setI", "SR-PS-SKEW-185:setI", "SR-PS-SKEW-186:setI", "SR-PS-SKEW-187:setI", "SR-PS-SKEW-191:setI", "SR-PS-SKEW-192:setI", "SR-PS-SKEW-193:setI", "SR-PS-SKEW-194:setI", "SR-PS-SKEW-195:setI", "SR-PS-SKEW-196:setI", "SR-PS-SKEW-197:setI", "SR-PS-SKEW-201:setI", "SR-PS-SKEW-202:setI", "SR-PS-SKEW-203:setI", "SR-PS-SKEW-204:setI", "SR-PS-SKEW-205:setI", "SR-PS-SKEW-206:setI", "SR-PS-SKEW-207:setI", "SR-PS-SKEW-211:setI", "SR-PS-SKEW-212:setI", "SR-PS-SKEW-213:setI", "SR-PS-SKEW-214:setI", "SR-PS-SKEW-215:setI", "SR-PS-SKEW-216:setI", "SR-PS-SKEW-217:setI", "SR-PS-SKEW-221:setI", "SR-PS-SKEW-222:setI", "SR-PS-SKEW-223:setI", "SR-PS-SKEW-224:setI", "SR-PS-SKEW-225:setI", "SR-PS-SKEW-226:setI", "SR-PS-SKEW-227:setI", "SR-PS-SKEW-231:setI", "SR-PS-SKEW-232:setI", "SR-PS-SKEW-233:setI", "SR-PS-SKEW-234:setI", "SR-PS-SKEW-235:setI", "SR-PS-SKEW-236:setI", "SR-PS-SKEW-237:setI", "SR-PS-SKEW-241:setI", "SR-PS-SKEW-242:setI", "SR-PS-SKEW-243:setI", "SR-PS-SKEW-244:setI", "SR-PS-SKEW-245:setI", "SR-PS-SKEW-246:setI", "SR-PS-SKEW-247:setI", "SR-RF2-LLRF:setGapVoltage", "SR-RF2-LLRF:setStationPhase", "SR-RF3-LLRF:setGapVoltage", "SR-RF3-LLRF:setStationPhase", "SR-PS-DMB09-Q1:setI", "SR-PS-DMB09-Q2:setI", "SR-PS-DMB09-Q3:setI", "SR-PS-DMB25-Q1:setI", "SR-PS-DMB25-Q2:setI", "SR-PS-DMB25-Q3:setI", "SR-PS-DMB41-Q1:setI", "SR-PS-DMB41-Q2:setI", "SR-PS-DMB41-Q3:setI", "SR-PS-DMB09-HC1:setI", "SR-PS-DMB09-HC2:setI", "SR-PS-DMB09-VC1:setI", "SR-PS-DMB09-VC2:setI", "SR-PS-DMB25-HC1:setI", "SR-PS-DMB25-HC2:setI", "SR-PS-DMB25-VC1:setI", "SR-PS-DMB25-VC2:setI", "SR-PS-DMB41-HC1:setI", "SR-PS-DMB41-HC2:setI", "SR-PS-DMB41-VC1:setI", "SR-PS-DMB41-VC2:setI", "SR-ID-IU22-05:setGap", "SR-ID-IU22A-09:setGap", "SR-ID-IU22B-09:setGap", "SR-ID-IUT22-21:setGap", "SR-ID-IU22-23:setGap", "SR-ID-IU22A-25:setGap", "SR-ID-IU22B-25:setGap", "SR-ID-EPU48A-41:setGap", "SR-ID-EPU48A-41:setPhase", "SR-ID-EPU48B-41:setGap", "SR-ID-EPU48B-41:setPhase", "SR-ID-EPU46-45:setGap", "SR-ID-EPU46-45:setPhase", "SR-ID-IUT22-21:setGapTaper", "SR-ID-EPU48PS-41:setGap", "SR-ID-IU22-05:gapMotorOff", "SR-ID-IU22A-09:gapMotorOff", "SR-ID-IU22B-09:gapMotorOff", "SR-ID-IUT22-21:gapMotorOff", "SR-ID-IU22-23:gapMotorOff", "SR-ID-IU22A-25:gapMotorOff", "SR-ID-IU22B-25:gapMotorOff", "SR-ID-EPU48A-41:gapMotorOff", "SR-ID-EPU48B-41:gapMotorOff", "SR-ID-EPU46-45:gapMotorOff", "SR-ID-EPU48A-41:phaseMotorOff", "SR-ID-EPU48B-41:phaseMotorOff", "SR-ID-EPU46-45:phaseMotorOff", "SR-DI-FOFB-H:setStatus", "SR-DI-FOFB-V:setStatus", "IGPF:TPSX:FBCTRL", "IGPF:TPSY:FBCTRL", "TPS-SR-022:bpm3:ilk:enabled", "SR-DI-ANGLE-ILK:StatusX", "SR-DI-ANGLE-ILK:StatusY", "SR-DI-RF-FB:setStatus", "SR-ID-EPU48-TFF:status", "SR-ID-EPU48-CFF:status", "SR-ID-EPU46-TFF:status", "SR-ID-EPU46-CFF:status", "TI-INJ-PROC:TopupHiLowStart"]
  out "result":string="Beam Trip Events \nTatal Counts: 0"
  in  "last ? Hrs":dbl=12.0 min=1.0 max=24.0 step=1.0
  in  "Trip Evt B":bool
  in  "Show Check list Button":bool=TRUE
  in  "View Diff Button":bool
  in  "Save Lattice Button":bool
  in  "Refresh B":bool
  out "x = y?":bool
  out "NOW time":string="15:45:10"
  out "NOW date":string="2017/10/28"
  in  "Save Button":bool
  out "error out 3":errorcluster
  in  "stop":bool
  out "time kickeron":string="15:43:52"
  out "date kickeron":string="2017/10/28"
  out "Orbit ILK(A)":bool
  out "Orbit INT. Ang Active":bool
  out "Orbit INT.Ang. On":bool
  out "Orbit INT. Pos Active":bool
  out "Orbit INT.Pos. On":bool
  in  "Copy Button":bool
  in  "Print Button":bool
  in  "Help Button":bool
  in  "Open Button":bool
  # "TPS OP Handover Information"
  # "Others"
  # "Additional Functions"
  # "Time："
  # "follow"
  # "歷史電流圖\ntrip次數?\n輻射劑量?\n平均氣壓\n目前最高累計劑量\n最近一次觸發時BR電流及WCM數值"
  # "Valve  Status"
  # "TFF"
  # "CFF"
  # "SM Status"
  # "TPS Operational Handover Information v1.5.3"
  # "SR Status"
  # "Feedback"
  # "Pulse Mag"
  # "LINAC"
  # "x8(ns)"
  # "x2(ns)"
  # "x0.01(ns)"
  # "RF Status"
  # "Hz"
  # "(kV)"
  # "(kV)"
  # "Changeliang@LOP.NSRRC"
  # "BR Fill Pattern"
  # "SR Fill Pattern"
  # "Lattice Files in Using"
  # "ID &Beamline [R]"
  # "Gap\nmm"
  # "Motor"
  # "Phase"
  # "FE/Hutch"
  # "Mode"
  # "Phase\nShifter"
  # "XBPM1X\num"
  # "XBPM1Y\num"
  # "XBPM2X\num"
  # "XBPM2Y\num"
  # "Note"
  # "05"
  # "09"
  # "Taper(enc)"
  # "21"
  # "23"
  # "25"
  # "41"
  # "45"
  # "SR Orbit"
  # "BPMX"
  # "BPMY"
  # "SR Beam Current History"
  # "ns"
  # "threshold:0.05mA"
  # "Adjusted History\n#Note: This file recorded PVs(set values) that were changed during this time.\n#(RF frequency was not recorded in this file)"
  # "Event Time"
  # "PV_name"
  # "Ori_Value"
  # "New_Value"
  # "hrs"
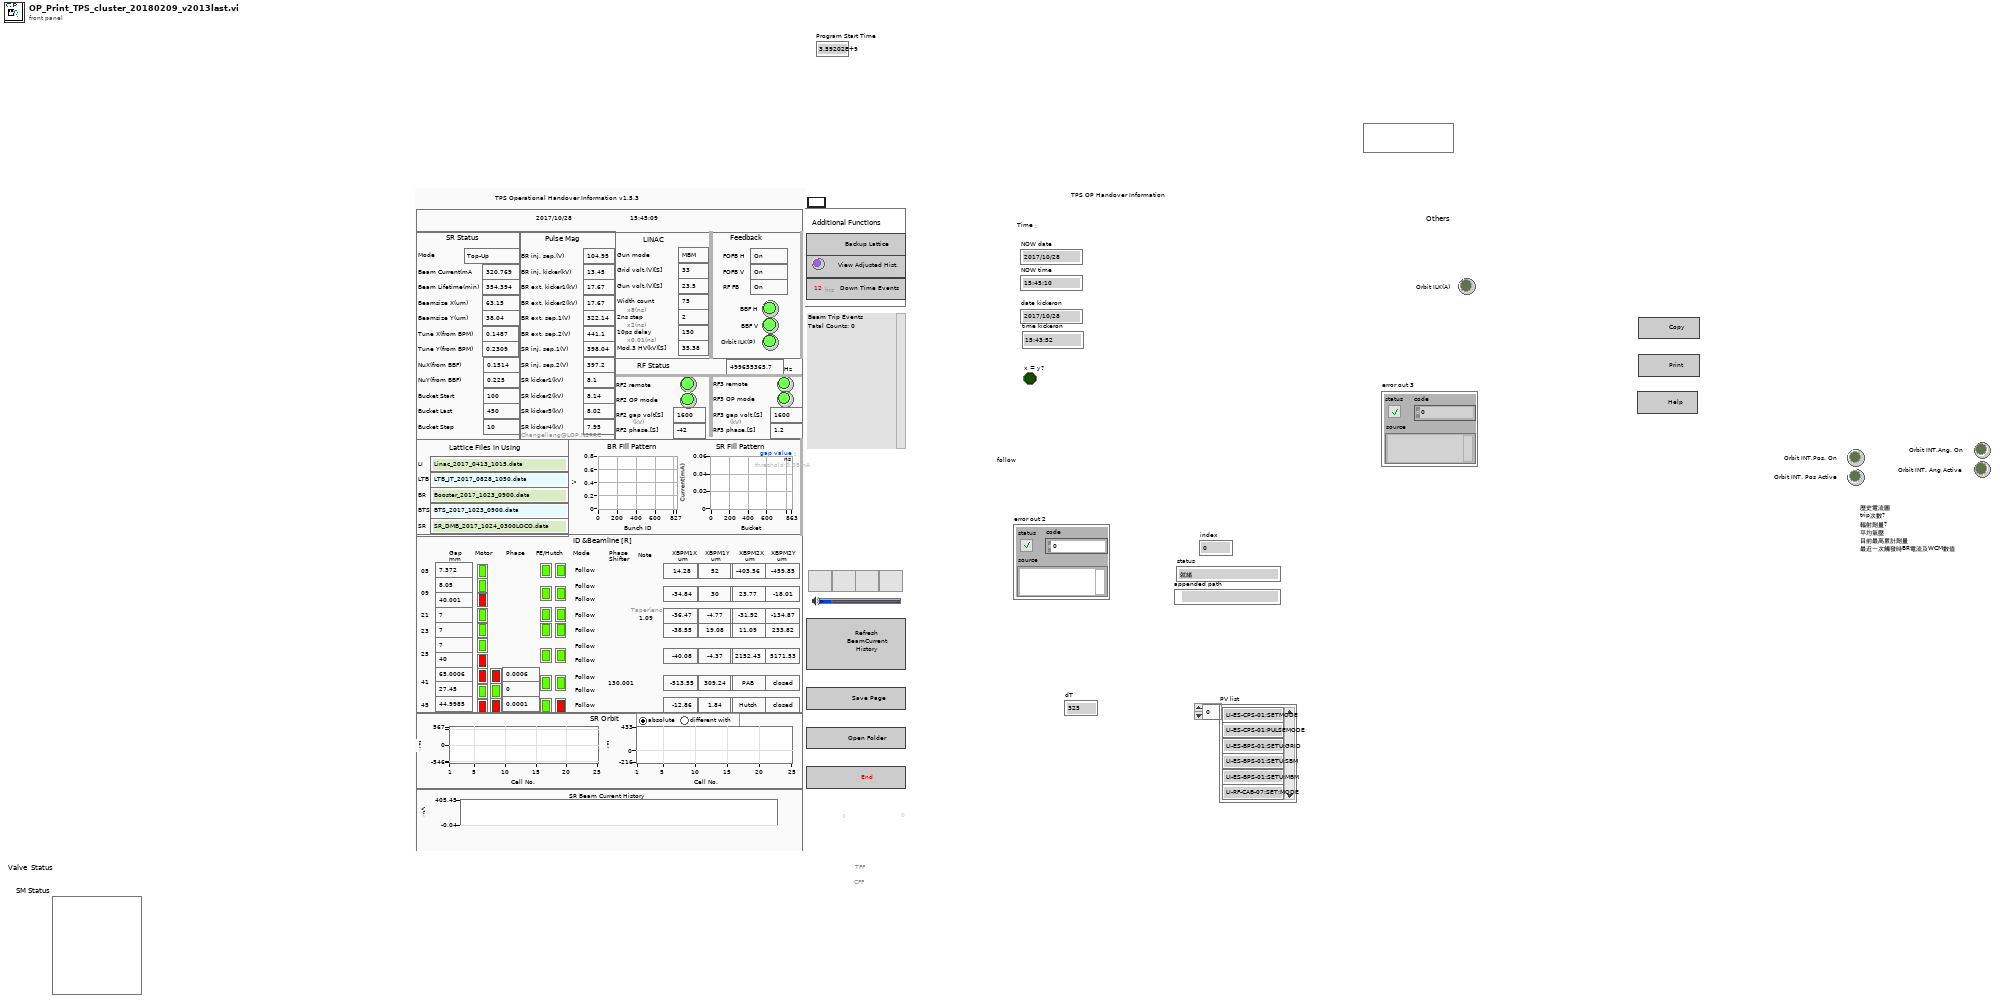
[diagram p1: front panel]
types:
  T1 = cluster{"SR Fill Pattern":dbl[], "Beam Current(mA":dbl, "Beam Lifetime(min)":dbl, "Beamsize X(um)":dbl, "Beamsize Y(um)":dbl, "Tune X(from BPM)":dbl, "Tune Y(from BPM)":dbl, "Mode":string, "NuX(from BBF) ":dbl, "NuY(from BBF)":dbl, "IU22-23gap(R)":dbl, "IU22-05gap(R)":dbl, "IU22-05M":bool, "IU22A-09gap(R)":dbl, "IU22A-09M":bool, "IU22B-09gap(R)":dbl, "IU22B-09M":bool, "IUT22-21gap(R)":dbl, "IUT22-21M":bool, "IU22-23M":bool, "IU22A-25gap(R)":dbl, "IU22A-25M":bool, "IU22B-25gap(R)":dbl, "IU22B-25M":bool, "EPU48A-41gap(R)":dbl, "EPU48A-41gM":bool, "EPU48B-41gap(R)":dbl, "EPU48B-41gM":bool, "EPU46-45gap(R)":dbl, "EPU46-45gM":bool, "EPU48A-41phase(R)":dbl, "EPU48B-41phase(R)":dbl, "EPU46-45phase(R)":dbl, "Grid volt.(V)[S]":dbl, "Gun mode":string, "Mod.3 HV(kV)[S]":dbl, "SR":string, "BR":string, "LI":string, "LTB":string, "BTS":string, "RF2 remote":bool, "RF2 OP mode":bool, "RF2 phase.[S]":dbl, "RF Freq.(s)":dbl, "RF2 gap volt[S]":dbl, "RF3 remote":bool, "RF3 OP mode":bool, "RF3 phase.[S]":dbl, "RF3 gap volt.[S]":dbl, "BBF V":bool, "BBF H":bool, "BR ext. kicker1(kV)":dbl, "BR ext. kicker2(kV)":dbl, "BR ext. sep.1(V)":dbl, "BR ext. sep.2(V)":dbl, "BR inj. sep.(V)":dbl, "BR inj. kicker(kV)":dbl, "SR kicker4(kV)":dbl, "SR kicker3(kV)":dbl, "SR kicker2(kV)":dbl, "SR kicker1(kV)":dbl, "SR inj. sep.2(V)":dbl, "SR inj. sep.1(V)":dbl, "Bucket Start":dbl, "Bucket Last":dbl, "Bucket Step":dbl, "Orbit ILK(P)":bool, "IU22-05 Hutch Enable":bool, "IU22A-09M Hutch Enable":bool, "IUT22-21M Hutch Enable":bool, "IU22-23M Hutch Enable":bool, "IU22A-25M Hutch Enable":bool, "EPU48A-41M Hutch Enable":bool, "EPU46-45M Hutch Enable":bool, "EPU46-45 FE Enable":bool, "EPU48A-41 FE Enable":bool, "IU22A-25 FE Enable":bool, "IU22-23 FE Enable":bool, "IUT22-21 FE Enable":bool, "IU22A-09 FE Enable":bool, "IU22-05 FE Enable":bool, "EPU48A-41pM":bool, "EPU48B-41pM":bool, "EPU46-45pM":bool, "Gun volt.(V)[S]":dbl, "Width count":dbl, "2ns step":dbl, "10ps delay":dbl, "phase shifter":dbl, "Taper":dbl, "05XBPMX 1":dbl, "09XBPMX 1":dbl, "21XBPMX 1":dbl, "23XBPMX 1":dbl, "25XBPMX 1":dbl, "41XBPMX 1":dbl, "45XBPMX 1":dbl, "05XBPMY 1":dbl, "09XBPMY 1":dbl, "21XBPMY 1":dbl, "23XBPMY 1":dbl, "25XBPMY 1":dbl, "41XBPMY 1":dbl, "45XBPMY 1":dbl, "FOFB H":string, "FOFB V":string, "time string":string, "date":string, "date (last kicker ON)":string, "time string (last kicker ON)":string, "Radio Buttons 2":enum32{"absolute", "different with"}, "09XBPMX 2":string, "09XBPMY 2":string, "05XBPMY 2":string, "05XBPMX 2":string, "21XBPMY 2":string, "21XBPMX 2":string, "23XBPMY 2":string, "23XBPMX 2":string, "25XBPMY 2":string, "25XBPMX 2":string, "41XBPMY 2":string, "41XBPMX 2":string, "45XBPMX 2":string, "45XBPMY 2":string, "05 mode":string, "09A mode":string, "09B mode":string, "21 mode":string, "23 mode":string, "25A mode":string, "25B mode":string, "41A mode":string, "41B mode":string, "46 mode":string, "BeamCurrent History":cluster{"BPM NO.  1_172":dbl[], dbl[]}, "SR Beam Current in            hours":dbl, "RF FB":string, "gap value：":i32, "BR Fill Pattern":dbl[], "time string (last INJ) ":string, "BPMX Graph 2":cluster{"Array of X axis  平均分配至各段":dbl[], dbl[]}, "BPMY Graph 2":cluster{"Array of X axis  平均分配至各段":dbl[], dbl[]}}
  T2 = typedef "NI_Database_API.lvlib/Conn ObjectReference.ctl" = refnum<k1>
  T3 = typedef "NI_Database_API.lvlib/Rec ObjectReference.ctl" = refnum<k1>
  T4 = typedef "imagedata.ctl" = cluster{"image type":i32, "image depth":i32, "image":u8[], "mask":u8[], "colors":u32[], "Rectangle":cluster{"left":i16, "top":i16, "right":i16, "bottom":i16}}
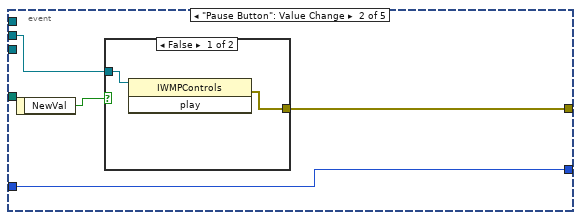
[diagram p6: hidden frame]
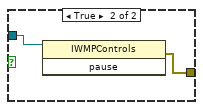
[diagram p7: hidden frame]
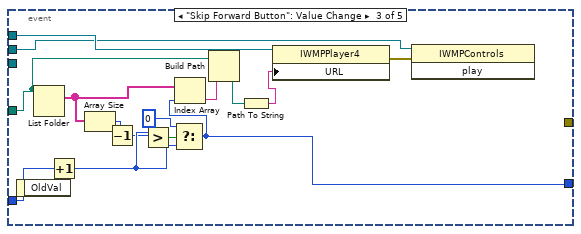
[diagram p8: hidden frame]
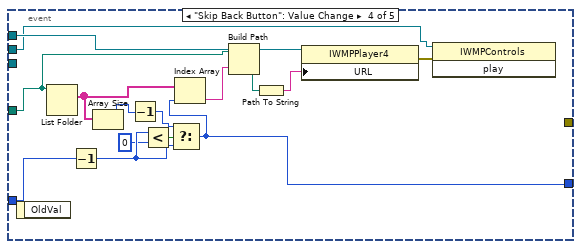
[diagram p9: hidden frame]
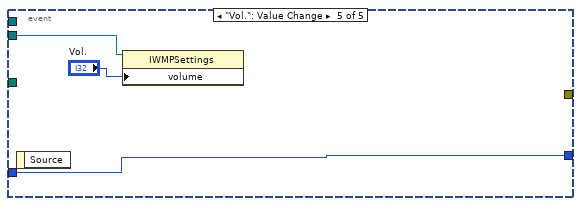
[diagram p10: hidden frame]
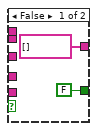
[diagram p13: hidden frame]
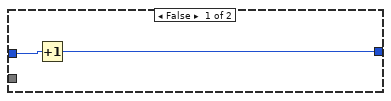
[diagram p14: hidden frame]
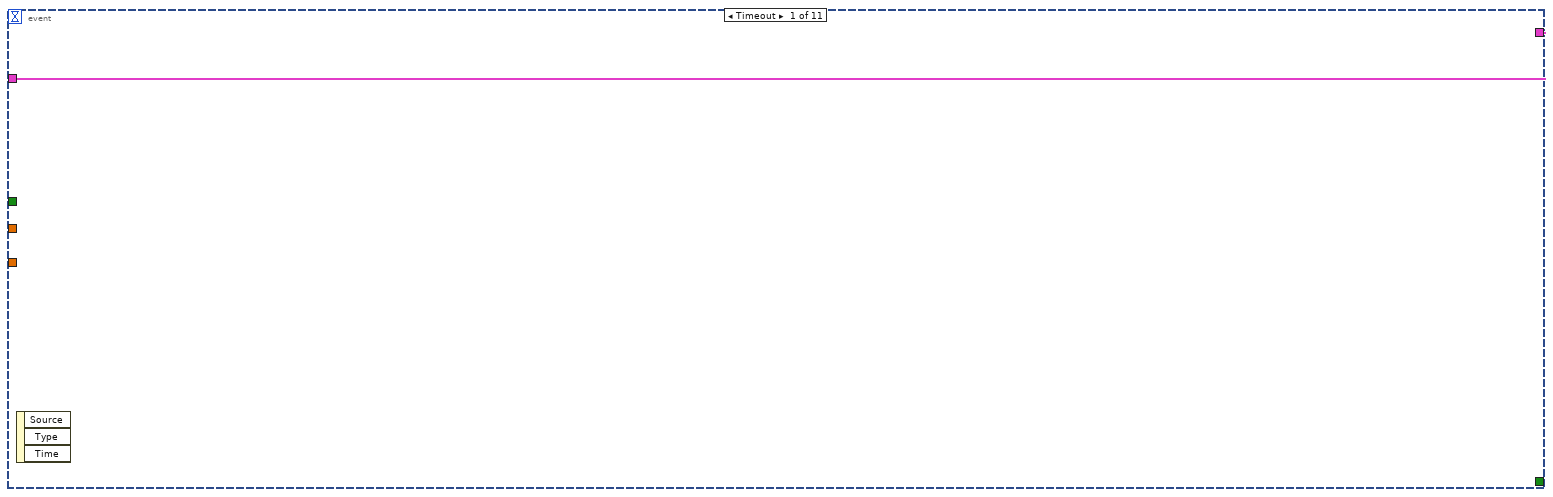
[diagram p19: hidden frame]
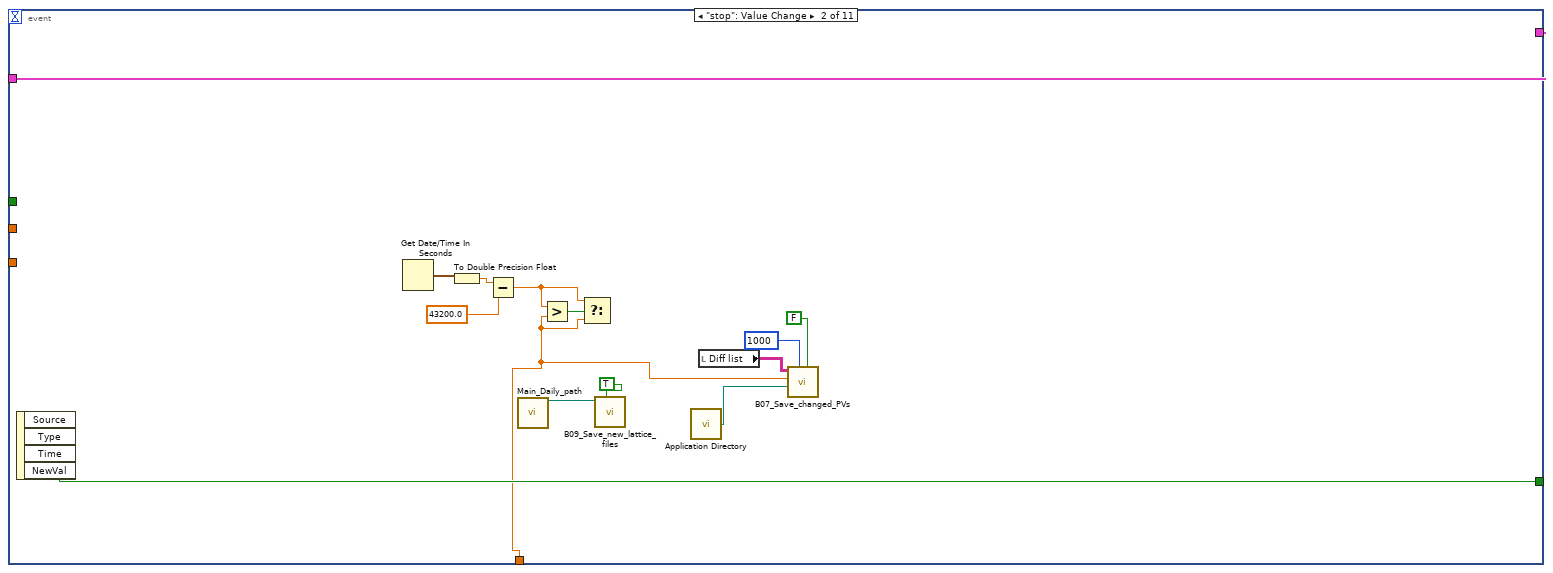
[diagram p20: hidden frame]
diagram:
  w17 = 0 ("index")
  w24 = string[] ["BR-PS-HC-101:setI", "BR-PS-HC-102:setI", "BR-PS-HC-103:setI", "BR-PS-HC-104:setI", "BR-PS-HC-105:setI", "BR-PS-HC-106:setI", "BR-PS-HC-107:setI", "BR-PS-HC-108:setI", "BR-PS-HC-109:setI", "BR-PS-HC-110:setI", "BR-PS-HC-201:setI", "BR-PS-HC-202:setI", "BR-PS-HC-203:setI", "BR-PS-HC-204:setI", "BR-PS-HC-205:setI", "BR-PS-HC-206:setI", "BR-PS-HC-207:setI", "BR-PS-HC-208:setI", "BR-PS-HC-209:setI", "BR-PS-HC-210:setI", "BR-PS-HC-301:setI", "BR-PS-HC-302:setI", "BR-PS-HC-303:setI", "BR-PS-HC-304:setI", "BR-PS-HC-305:setI", "BR-PS-HC-306:setI", "BR-PS-HC-307:setI", "BR-PS-HC-308:setI", "BR-PS-HC-309:setI", "BR-PS-HC-310:setI", "BR-PS-HC-401:setI", "BR-PS-HC-402:setI", "BR-PS-HC-403:setI", "BR-PS-HC-404:setI", "BR-PS-HC-405:setI", "BR-PS-HC-406:setI", "BR-PS-HC-407:setI", "BR-PS-HC-408:setI", "BR-PS-HC-409:setI", "BR-PS-HC-410:setI", "BR-PS-HC-501:setI", "BR-PS-HC-502:setI", "BR-PS-HC-503:setI", "BR-PS-HC-504:setI", "BR-PS-HC-505:setI", "BR-PS-HC-506:setI", "BR-PS-HC-507:setI", "BR-PS-HC-508:setI", "BR-PS-HC-509:setI", "BR-PS-HC-510:setI", "BR-PS-HC-601:setI", "BR-PS-HC-602:setI", "BR-PS-HC-603:setI", "BR-PS-HC-603a:setI", "BR-PS-HC-604:setI", "BR-PS-HC-605:setI", "BR-PS-HC-606:setI", "BR-PS-HC-606a:setI", "BR-PS-HC-607:setI", "BR-PS-HC-608:setI", "BR-PS-HC-609:setI", "BR-PS-HC-610:setI", "BR-PS-VC-101:setI", "BR-PS-VC-102:setI", "BR-PS-VC-103:setI", "BR-PS-VC-104:setI", "BR-PS-VC-105:setI", "BR-PS-VC-106:setI", "BR-PS-VC-201:setI", "BR-PS-VC-202:setI", "BR-PS-VC-203:setI", "BR-PS-VC-204:setI", "BR-PS-VC-205:setI", "BR-PS-VC-206:setI", "BR-PS-VC-301:setI", "BR-PS-VC-302:setI", "BR-PS-VC-303:setI", "BR-PS-VC-304:setI", "BR-PS-VC-305:setI", "BR-PS-VC-306:setI", "BR-PS-VC-401:setI", "BR-PS-VC-402:setI", "BR-PS-VC-403:setI", "BR-PS-VC-404:setI", "BR-PS-VC-405:setI", "BR-PS-VC-406:setI", "BR-PS-VC-501:setI", "BR-PS-VC-502:setI", "BR-PS-VC-503:setI", "BR-PS-VC-504:setI", "BR-PS-VC-505:setI", "BR-PS-VC-506:setI", "BR-PS-VC-601:setI", "BR-PS-VC-602:setI", "BR-PS-VC-602a:setI", "BR-PS-VC-603:setI", "BR-PS-VC-604:setI", "BR-PS-VC-604a:setI", "BR-PS-VC-605:setI", "BR-PS-VC-606:setI", "BR-PS-VC-100a:setI", "BR-PS-SD:setI", "BR-PS-SF:setI", "cpsc_027:AO:SLOW_SET:CH:1", "BR-RF-LLRF:setStationPhase", "TI-INJ-PROC:setTinj", "BR-PS-INJ-SE:setHV", "CPCIPM-TI-EVR:Pulse1DelaySet", "BR-PS-INJ-KI:setHV", "CPCIPM-TI-EVR:Pulse2DelaySet", "BR-PS-QF:setWfDC", "BR-PS-QM:setWfDC", "BR-PS-Q1:setWfDC", "BR-PS-Q2:setWfDC", "BR-PS-BEND:setWfDC"]  # PV nanes (BR_without_Wf, cpsc_037:AO:SLOW_SET:CH:3)
  w25 = string[] ["LI-ES-CPS-01:SETMODE", "LI-ES-CPS-01:PULSEMODE", "LI-ES-BPS-01:SETU:GRID", "LI-ES-BPS-01:SETU:SBM", "LI-ES-BPS-01:SETU:MBM", "LI-RF-CAB-07:SET:MODE", "LI-RF-HVP-11:SET:U", "LI-RF-CAB-09:SET:MODE", "LI-RF-HVP-21:SET:U", "LI-RF-HVP-31:SET:U", "LI-RF-WGA-01:SET:POS", "LI-RF-WGA-02:SET:POS", "LI-RF-WGA-03:SET:POS", "LI-RF-SFT-01:SET:POS", "LI-RF-SFT-02:SET:POS", "LI-RF-SFT-03:SET:POS", "LI-RF-CTR-01:ES:SET:DEG", "LI-RF-CTR-01:SP:SET:DEG", "LI-RF-CTR-01:K123:SET:DEG", "LI-RF-CTR-01:K1:SET:DEG", "LI-RF-CTR-01:K3:SET:DEG", "LI-RF-AMP-01:SET:PWR", "LI-RF-AMP-02:SET:PWR", "LI-MA-SPS-01:SET:I", "LI-MA-SPS-02:SET:I", "LI-MA-SPS-03:SET:I", "LI-MA-SPS-04:SET:I", "LI-MA-SPS-05:SET:I", "LI-MA-SPS-06:SET:I", "LI-MA-SPS-07:SET:I", "LI-MA-SPS-08:SET:I", "LI-MA-SPS-09:SET:I", "LI-MA-SPS-10:SET:I", "LI-MA-SPS-11:SET:I", "LI-MA-SPS-12:SET:I", "LI-MA-SPS-13:SET:I", "LI-MA-SPS-14:SET:I", "LI-MA-SPS-15:SET:I", "LI-MA-SPS-16:SET:I", "LI-MA-STP-01:SET:I", "LI-MA-STP-02:SET:I", "LI-MA-STP-03:SET:I", "LI-MA-STP-04:SET:I", "LI-MA-STP-05:SET:I", "LI-MA-STP-06:SET:I", "LI-MA-STP-07:SET:I", "LI-MA-STP-08:SET:I", "LI-MA-STP-09:SET:I", "LI-MA-STP-10:SET:I", "LI-MA-STP-11:SET:I", "LI-MA-STP-12:SET:I", "LI-MA-STP-13:SET:I", "LI-MA-STP-14:SET:I", "LI-MA-STP-15:SET:I", "LI-MA-STP-16:SET:I", "LI-MA-QPS-01:SET:I", "LI-MA-QPS-02:SET:I", "LI-MA-QPS-03:SET:I", "LI-MA-QPS-04:SET:I", "LI-MA-QPS-05:SET:I", "LI-MA-QPS-06:SET:I", "CPCITM-TI-EVRTG:Pulse7DelaySet", "CPCITM-TI-EVRTG:Pulse7WidthSet", "CPCITM-TI-EVRTG:GTX7DlySet", "CPCITM-TI-EVRTG:Pulse6DelaySet", "CPCITM-TI-EVRTG:Pulse6WidthSet", "CPCITM-TI-EVRTG:GTX6DlySet", "CPCILI-TI-EVR:Pulse2DelaySet", "CPCILI-TI-EVR:Pulse2WidthSet", "CPCILI-TI-EVR:Pulse3DelaySet", "CPCILI-TI-EVR:Pulse3WidthSet", "CPCILI-TI-EVR:Pulse4DelaySet", "CPCILI-TI-EVR:Pulse4WidthSet", "CPCILI-TI-EVR:Pulse5DelaySet", "CPCILI-TI-EVR:Pulse5WidthSet", "CPCILI-TI-EVR:Pulse6DelaySet", "CPCILI-TI-EVR:Pulse6WidthSet", "CPCILI-TI-EVR:Pulse7DelaySet", "CPCILI-TI-EVR:Pulse7WidthSet", "CPCILI-TI-EVR:Pulse8DelaySet", "CPCILI-TI-EVR:Pulse8WidthSet", "CPCILI-TI-EVR:Pulse9DelaySet", "CPCILI-TI-EVR:Pulse9WidthSet", "CPCITM-TI-EVRTG:GTX6DlySet", "CPCITM-TI-EVRTG:GTX7DlySet"]  # PV nanes(LINAC) without 3 set
  w26 = string[] ["TI-INJ-PROC:TopupHiLowStart", "TI-INJ-PROC:setBucketAddressStart", "TI-INJ-PROC:setBucketAddressLast", "TI-INJ-PROC:setBucketAddressStep", "TI-INJ-PROC:setPreCycle", "TI-INJ-PROC:setPostCycle", "TI-INJ-PROC:setBeamCurrentTopupHi", "TI-INJ-PROC:setBeamCurrentTopupLo", "TI-INJ-PROC:setSingleBunchAddr", "TI-INJ-PROC:setSingleInjCycle", "TI-INJ-PROC:setSingleBeamCurrent"]  # PV nanes(Others)
  w27 = string[] ["SR-ID-IU22-05:setECMode", "SR-ID-IU22A-09:setECMode", "SR-ID-IU22B-09:setECMode", "SR-ID-IUT22-21:setECMode", "SR-ID-IU22-23:setECMode", "SR-ID-IU22A-25:setECMode", "SR-ID-IU22B-25:setECMode", "SR-ID-EPU48A-41:setECMode", "SR-ID-EPU48B-41:setECMode", "SR-ID-EPU46-45:setECMode"]  # ID_mode
  (unwired) "cpsc_037:AO:SLOW_SET:CH:3" ("regular expression")
  w28 = string[] ["SR-DI-XPC-40:cam:AcquireTime", "SR-DI-XPC-40:cam:Gain"]  # Port40
  w29 = string[] ["LI:controlState0", "TI-INJ-PROC:trig-BRAC-ONOFF", "SR:controlState0"]  # Power Saving
  (unwired) "CPCITM-TI-EVRTG:GTX6CtrlGTXPHSet" ("regular expression")
  (unwired) "CPCITM-TI-EVRTG:GTX7CtrlGTXPHSet" ("regular expression")
  w32 = string[] ["SR-ID-IU22-05:gapMotorOff", "SR-ID-IU22A-09:gapMotorOff", "SR-ID-IU22B-09:gapMotorOff", "SR-ID-IUT22-21:gapMotorOff", "SR-ID-IU22-23:gapMotorOff", "SR-ID-IU22A-25:gapMotorOff", "SR-ID-IU22B-25:gapMotorOff", "SR-ID-EPU48A-41:gapMotorOff", "SR-ID-EPU48B-41:gapMotorOff", "SR-ID-EPU46-45:gapMotorOff", "SR-ID-EPU48A-41:phaseMotorOff", "SR-ID-EPU48B-41:phaseMotorOff", "SR-ID-EPU46-45:phaseMotorOff"]  # ID MO
  w31 = string[] ["SR-ID-IU22-05:setGap", "SR-ID-IU22A-09:setGap", "SR-ID-IU22B-09:setGap", "SR-ID-IUT22-21:setGap", "SR-ID-IU22-23:setGap", "SR-ID-IU22A-25:setGap", "SR-ID-IU22B-25:setGap", "SR-ID-EPU48A-41:setGap", "SR-ID-EPU48A-41:setPhase", "SR-ID-EPU48B-41:setGap", "SR-ID-EPU48B-41:setPhase", "SR-ID-EPU46-45:setGap", "SR-ID-EPU46-45:setPhase", "SR-ID-IUT22-21:getGapTaper", "SR-ID-EPU48PS-41:setGap", "SR-ID-IUT22-21:setGapMode"]  # PV nanes(ID gap_phase_Taper_)
  w40 = string[] ["SR-PS-BEND:setI", "SR-PS-HC-011:setI", "SR-PS-HC-012:setI", "SR-PS-HC-013:setI", "SR-PS-HC-014:setI", "SR-PS-HC-015:setI", "SR-PS-HC-016:setI", "SR-PS-HC-017:setI", "SR-PS-HC-021:setI", "SR-PS-HC-022:setI", "SR-PS-HC-023:setI", "SR-PS-HC-024:setI", "SR-PS-HC-025:setI", "SR-PS-HC-026:setI", "SR-PS-HC-027:setI", "SR-PS-HC-031:setI", "SR-PS-HC-032:setI", "SR-PS-HC-033:setI", "SR-PS-HC-034:setI", "SR-PS-HC-035:setI", "SR-PS-HC-036:setI", "SR-PS-HC-037:setI", "SR-PS-HC-041:setI", "SR-PS-HC-042:setI", "SR-PS-HC-043:setI", "SR-PS-HC-044:setI", "SR-PS-HC-045:setI", "SR-PS-HC-046:setI", "SR-PS-HC-047:setI", "SR-PS-HC-051:setI", "SR-PS-HC-052:setI", "SR-PS-HC-053:setI", "SR-PS-HC-054:setI", "SR-PS-HC-055:setI", "SR-PS-HC-056:setI", "SR-PS-HC-057:setI", "SR-PS-HC-061:setI", "SR-PS-HC-062:setI", "SR-PS-HC-063:setI", "SR-PS-HC-064:setI", "SR-PS-HC-065:setI", "SR-PS-HC-066:setI", "SR-PS-HC-067:setI", "SR-PS-HC-071:setI", "SR-PS-HC-072:setI", "SR-PS-HC-073:setI", "SR-PS-HC-074:setI", "SR-PS-HC-075:setI", "SR-PS-HC-076:setI", "SR-PS-HC-077:setI", "SR-PS-HC-081:setI", "SR-PS-HC-082:setI", "SR-PS-HC-083:setI", "SR-PS-HC-084:setI", "SR-PS-HC-085:setI", "SR-PS-HC-086:setI", "SR-PS-HC-087:setI", "SR-PS-HC-091:setI", "SR-PS-HC-092:setI", "SR-PS-HC-093:setI", "SR-PS-HC-094:setI", "SR-PS-HC-095:setI", "SR-PS-HC-096:setI", "SR-PS-HC-097:setI", "SR-PS-HC-101:setI", "SR-PS-HC-102:setI", "SR-PS-HC-103:setI", "SR-PS-HC-104:setI", "SR-PS-HC-105:setI", "SR-PS-HC-106:setI", "SR-PS-HC-107:setI", "SR-PS-HC-111:setI", "SR-PS-HC-112:setI", "SR-PS-HC-113:setI", "SR-PS-HC-114:setI", "SR-PS-HC-115:setI", "SR-PS-HC-116:setI", "SR-PS-HC-117:setI", "SR-PS-HC-121:setI", "SR-PS-HC-122:setI", "SR-PS-HC-123:setI", "SR-PS-HC-124:setI", "SR-PS-HC-125:setI", "SR-PS-HC-126:setI", "SR-PS-HC-127:setI", "SR-PS-HC-131:setI", "SR-PS-HC-132:setI", "SR-PS-HC-133:setI", "SR-PS-HC-134:setI", "SR-PS-HC-135:setI", "SR-PS-HC-136:setI", "SR-PS-HC-137:setI", "SR-PS-HC-141:setI", "SR-PS-HC-142:setI", "SR-PS-HC-143:setI", "SR-PS-HC-144:setI", "SR-PS-HC-145:setI", "SR-PS-HC-146:setI", "SR-PS-HC-147:setI", "SR-PS-HC-151:setI", "SR-PS-HC-152:setI", "SR-PS-HC-153:setI", "SR-PS-HC-154:setI", "SR-PS-HC-155:setI", "SR-PS-HC-156:setI", "SR-PS-HC-157:setI", "SR-PS-HC-161:setI", "SR-PS-HC-162:setI", "SR-PS-HC-163:setI", "SR-PS-HC-164:setI", "SR-PS-HC-165:setI", "SR-PS-HC-166:setI", "SR-PS-HC-167:setI", "SR-PS-HC-171:setI", "SR-PS-HC-172:setI", "SR-PS-HC-173:setI", "SR-PS-HC-174:setI", "SR-PS-HC-175:setI", "SR-PS-HC-176:setI", "SR-PS-HC-177:setI", "SR-PS-HC-181:setI", "SR-PS-HC-182:setI", "SR-PS-HC-183:setI", "SR-PS-HC-184:setI", "SR-PS-HC-185:setI", "SR-PS-HC-186:setI", "SR-PS-HC-187:setI", "SR-PS-HC-191:setI", "SR-PS-HC-192:setI", "SR-PS-HC-193:setI", "SR-PS-HC-194:setI", "SR-PS-HC-195:setI", "SR-PS-HC-196:setI", "SR-PS-HC-197:setI", "SR-PS-HC-201:setI", "SR-PS-HC-202:setI", "SR-PS-HC-203:setI", "SR-PS-HC-204:setI", "SR-PS-HC-205:setI", "SR-PS-HC-206:setI", "SR-PS-HC-207:setI", "SR-PS-HC-211:setI", "SR-PS-HC-212:setI", "SR-PS-HC-213:setI", "SR-PS-HC-214:setI", "SR-PS-HC-215:setI", "SR-PS-HC-216:setI", "SR-PS-HC-217:setI", "SR-PS-HC-221:setI", "SR-PS-HC-222:setI", "SR-PS-HC-223:setI", "SR-PS-HC-224:setI", "SR-PS-HC-225:setI", "SR-PS-HC-226:setI", "SR-PS-HC-227:setI", "SR-PS-HC-231:setI", "SR-PS-HC-232:setI", "SR-PS-HC-233:setI", "SR-PS-HC-234:setI", "SR-PS-HC-235:setI", "SR-PS-HC-236:setI", "SR-PS-HC-237:setI", "SR-PS-HC-241:setI", "SR-PS-HC-242:setI", "SR-PS-HC-243:setI", "SR-PS-HC-244:setI", "SR-PS-HC-245:setI", "SR-PS-HC-246:setI", "SR-PS-HC-247:setI", "SR-PS-VC-011:setI", "SR-PS-VC-012:setI", "SR-PS-VC-013:setI", "SR-PS-VC-014:setI", "SR-PS-VC-015:setI", "SR-PS-VC-016:setI", "SR-PS-VC-017:setI", "SR-PS-VC-021:setI", "SR-PS-VC-022:setI", "SR-PS-VC-023:setI", "SR-PS-VC-024:setI", "SR-PS-VC-025:setI", "SR-PS-VC-026:setI", "SR-PS-VC-027:setI", "SR-PS-VC-031:setI", "SR-PS-VC-032:setI", "SR-PS-VC-033:setI", "SR-PS-VC-034:setI", "SR-PS-VC-035:setI", "SR-PS-VC-036:setI", "SR-PS-VC-037:setI", "SR-PS-VC-041:setI", "SR-PS-VC-042:setI", "SR-PS-VC-043:setI", "SR-PS-VC-044:setI", "SR-PS-VC-045:setI", "SR-PS-VC-046:setI", "SR-PS-VC-047:setI", "SR-PS-VC-051:setI", "SR-PS-VC-052:setI", "SR-PS-VC-053:setI", "SR-PS-VC-054:setI", "SR-PS-VC-055:setI", "SR-PS-VC-056:setI", "SR-PS-VC-057:setI", "SR-PS-VC-061:setI", "SR-PS-VC-062:setI", "SR-PS-VC-063:setI", "SR-PS-VC-064:setI", "SR-PS-VC-065:setI", "SR-PS-VC-066:setI", "SR-PS-VC-067:setI", "SR-PS-VC-071:setI", "SR-PS-VC-072:setI", "SR-PS-VC-073:setI", "SR-PS-VC-074:setI", "SR-PS-VC-075:setI", "SR-PS-VC-076:setI", "SR-PS-VC-077:setI", "SR-PS-VC-081:setI", "SR-PS-VC-082:setI", "SR-PS-VC-083:setI", "SR-PS-VC-084:setI", "SR-PS-VC-085:setI", "SR-PS-VC-086:setI", "SR-PS-VC-087:setI", "SR-PS-VC-091:setI", "SR-PS-VC-092:setI", "SR-PS-VC-093:setI", "SR-PS-VC-094:setI", "SR-PS-VC-095:setI", "SR-PS-VC-096:setI", "SR-PS-VC-097:setI", "SR-PS-VC-101:setI", "SR-PS-VC-102:setI", "SR-PS-VC-103:setI", "SR-PS-VC-104:setI", "SR-PS-VC-105:setI", "SR-PS-VC-106:setI", "SR-PS-VC-107:setI", "SR-PS-VC-111:setI", "SR-PS-VC-112:setI", "SR-PS-VC-113:setI", "SR-PS-VC-114:setI", "SR-PS-VC-115:setI", "SR-PS-VC-116:setI", "SR-PS-VC-117:setI", "SR-PS-VC-121:setI", "SR-PS-VC-122:setI", "SR-PS-VC-123:setI", "SR-PS-VC-124:setI", "SR-PS-VC-125:setI", "SR-PS-VC-126:setI", "SR-PS-VC-127:setI", "SR-PS-VC-131:setI", "SR-PS-VC-132:setI", "SR-PS-VC-133:setI", "SR-PS-VC-134:setI", "SR-PS-VC-135:setI", "SR-PS-VC-136:setI", "SR-PS-VC-137:setI", "SR-PS-VC-141:setI", "SR-PS-VC-142:setI", "SR-PS-VC-143:setI", "SR-PS-VC-144:setI", "SR-PS-VC-145:setI", "SR-PS-VC-146:setI", "SR-PS-VC-147:setI", "SR-PS-VC-151:setI", "SR-PS-VC-152:setI", "SR-PS-VC-153:setI", "SR-PS-VC-154:setI", "SR-PS-VC-155:setI", "SR-PS-VC-156:setI", "SR-PS-VC-157:setI", "SR-PS-VC-161:setI", "SR-PS-VC-162:setI", "SR-PS-VC-163:setI", "SR-PS-VC-164:setI", "SR-PS-VC-165:setI", "SR-PS-VC-166:setI", "SR-PS-VC-167:setI", "SR-PS-VC-171:setI", "SR-PS-VC-172:setI", "SR-PS-VC-173:setI", "SR-PS-VC-174:setI", "SR-PS-VC-175:setI", "SR-PS-VC-176:setI", "SR-PS-VC-177:setI", "SR-PS-VC-181:setI", "SR-PS-VC-182:setI", "SR-PS-VC-183:setI", "SR-PS-VC-184:setI", "SR-PS-VC-185:setI", "SR-PS-VC-186:setI", "SR-PS-VC-187:setI", "SR-PS-VC-191:setI", "SR-PS-VC-192:setI", "SR-PS-VC-193:setI", "SR-PS-VC-194:setI", "SR-PS-VC-195:setI", "SR-PS-VC-196:setI", "SR-PS-VC-197:setI", "SR-PS-VC-201:setI", "SR-PS-VC-202:setI", "SR-PS-VC-203:setI", "SR-PS-VC-204:setI", "SR-PS-VC-205:setI", "SR-PS-VC-206:setI", "SR-PS-VC-207:setI", "SR-PS-VC-211:setI", "SR-PS-VC-212:setI", "SR-PS-VC-213:setI", "SR-PS-VC-214:setI", "SR-PS-VC-215:setI", "SR-PS-VC-216:setI", "SR-PS-VC-217:setI", "SR-PS-VC-221:setI", "SR-PS-VC-222:setI", "SR-PS-VC-223:setI", "SR-PS-VC-224:setI", "SR-PS-VC-225:setI", "SR-PS-VC-226:setI", "SR-PS-VC-227:setI", "SR-PS-VC-231:setI", "SR-PS-VC-232:setI", "SR-PS-VC-233:setI", "SR-PS-VC-234:setI", "SR-PS-VC-235:setI", "SR-PS-VC-236:setI", "SR-PS-VC-237:setI", "SR-PS-VC-241:setI", "SR-PS-VC-242:setI", "SR-PS-VC-243:setI", "SR-PS-VC-244:setI", "SR-PS-VC-245:setI", "SR-PS-VC-246:setI", "SR-PS-VC-247:setI", "SR-PS-QL1-0101:setI", "SR-PS-QL2-0102:setI", "SR-PS-QL3-0103:setI", "SR-PS-QS4-0104:setI", "SR-PS-QS5-0105:setI", "SR-PS-QS5-0106:setI", "SR-PS-QS4-0107:setI", "SR-PS-QS3-0108:setI", "SR-PS-QS2-0109:setI", "SR-PS-QS1-0110:setI", "SR-PS-QS1-0201:setI", "SR-PS-QS2-0202:setI", "SR-PS-QS3-0203:setI", "SR-PS-QS4-0204:setI", "SR-PS-QS5-0205:setI", "SR-PS-QS5-0206:setI", "SR-PS-QS4-0207:setI", "SR-PS-QS3-0208:setI", "SR-PS-QS2-0209:setI", "SR-PS-QS1-0210:setI", "SR-PS-QS1-0301:setI", "SR-PS-QS2-0302:setI", "SR-PS-QS3-0303:setI", "SR-PS-QS4-0304:setI", "SR-PS-QS5-0305:setI", "SR-PS-QS5-0306:setI", "SR-PS-QS4-0307:setI", "SR-PS-QS3-0308:setI", "SR-PS-QS2-0309:setI", "SR-PS-QS1-0310:setI", "SR-PS-QS1-0401:setI", "SR-PS-QS2-0402:setI", "SR-PS-QS3-0403:setI", "SR-PS-QS4-0404:setI", "SR-PS-QS5-0405:setI", "SR-PS-QS5-0406:setI", "SR-PS-QS4-0407:setI", "SR-PS-QL3-0408:setI", "SR-PS-QL2-0409:setI", "SR-PS-QL1-0410:setI", "SR-PS-QL1-0501:setI", "SR-PS-QL2-0502:setI", "SR-PS-QL3-0503:setI", "SR-PS-QS4-0504:setI", "SR-PS-QS5-0505:setI", "SR-PS-QS5-0506:setI", "SR-PS-QS4-0507:setI", "SR-PS-QS3-0508:setI", "SR-PS-QS2-0509:setI", "SR-PS-QS1-0510:setI", "SR-PS-QS1-0601:setI", "SR-PS-QS2-0602:setI", "SR-PS-QS3-0603:setI", "SR-PS-QS4-0604:setI", "SR-PS-QS5-0605:setI", "SR-PS-QS5-0606:setI", "SR-PS-QS4-0607:setI", "SR-PS-QS3-0608:setI", "SR-PS-QS2-0609:setI", "SR-PS-QS1-0610:setI", "SR-PS-QS1-0701:setI", "SR-PS-QS2-0702:setI", "SR-PS-QS3-0703:setI", "SR-PS-QS4-0704:setI", "SR-PS-QS5-0705:setI", "SR-PS-QS5-0706:setI", "SR-PS-QS4-0707:setI", "SR-PS-QS3-0708:setI", "SR-PS-QS2-0709:setI", "SR-PS-QS1-0710:setI", "SR-PS-QS1-0801:setI", "SR-PS-QS2-0802:setI", "SR-PS-QS3-0803:setI", "SR-PS-QS4-0804:setI", "SR-PS-QS5-0805:setI", "SR-PS-QS5-0806:setI", "SR-PS-QS4-0807:setI", "SR-PS-QL3-0808:setI", "SR-PS-QL2-0809:setI", "SR-PS-QL1-0810:setI", "SR-PS-QL1-0901:setI", "SR-PS-QL2-0902:setI", "SR-PS-QL3-0903:setI", "SR-PS-QS4-0904:setI", "SR-PS-QS5-0905:setI", "SR-PS-QS5-0906:setI", "SR-PS-QS4-0907:setI", "SR-PS-QS3-0908:setI", "SR-PS-QS2-0909:setI", "SR-PS-QS1-0910:setI", "SR-PS-QS1-1001:setI", "SR-PS-QS2-1002:setI", "SR-PS-QS3-1003:setI", "SR-PS-QS4-1004:setI", "SR-PS-QS5-1005:setI", "SR-PS-QS5-1006:setI", "SR-PS-QS4-1007:setI", "SR-PS-QS3-1008:setI", "SR-PS-QS2-1009:setI", "SR-PS-QS1-1010:setI", "SR-PS-QS1-1101:setI", "SR-PS-QS2-1102:setI", "SR-PS-QS3-1103:setI", "SR-PS-QS4-1104:setI", "SR-PS-QS5-1105:setI", "SR-PS-QS5-1106:setI", "SR-PS-QS4-1107:setI", "SR-PS-QS3-1108:setI", "SR-PS-QS2-1109:setI", "SR-PS-QS1-1110:setI", "SR-PS-QS1-1201:setI", "SR-PS-QS2-1202:setI", "SR-PS-QS3-1203:setI", "SR-PS-QS4-1204:setI", "SR-PS-QS5-1205:setI", "SR-PS-QS5-1206:setI", "SR-PS-QS4-1207:setI", "SR-PS-QL3-1208:setI", "SR-PS-QL2-1209:setI", "SR-PS-QL1-1210:setI", "SR-PS-QL1-1301:setI", "SR-PS-QL2-1302:setI", "SR-PS-QL3-1303:setI", "SR-PS-QS4-1304:setI", "SR-PS-QS5-1305:setI", "SR-PS-QS5-1306:setI", "SR-PS-QS4-1307:setI", "SR-PS-QS3-1308:setI", "SR-PS-QS2-1309:setI", "SR-PS-QS1-1310:setI", "SR-PS-QS1-1401:setI", "SR-PS-QS2-1402:setI", "SR-PS-QS3-1403:setI", "SR-PS-QS4-1404:setI", "SR-PS-QS5-1405:setI", "SR-PS-QS5-1406:setI", "SR-PS-QS4-1407:setI", "SR-PS-QS3-1408:setI", "SR-PS-QS2-1409:setI", "SR-PS-QS1-1410:setI", "SR-PS-QS1-1501:setI", "SR-PS-QS2-1502:setI", "SR-PS-QS3-1503:setI", "SR-PS-QS4-1504:setI", "SR-PS-QS5-1505:setI", "SR-PS-QS5-1506:setI", "SR-PS-QS4-1507:setI", "SR-PS-QS3-1508:setI", "SR-PS-QS2-1509:setI", "SR-PS-QS1-1510:setI", "SR-PS-QS1-1601:setI", "SR-PS-QS2-1602:setI", "SR-PS-QS3-1603:setI", "SR-PS-QS4-1604:setI", "SR-PS-QS5-1605:setI", "SR-PS-QS5-1606:setI", "SR-PS-QS4-1607:setI", "SR-PS-QL3-1608:setI", "SR-PS-QL2-1609:setI", "SR-PS-QL1-1610:setI", "SR-PS-QL1-1701:setI", "SR-PS-QL2-1702:setI", "SR-PS-QL3-1703:setI", "SR-PS-QS4-1704:setI", "SR-PS-QS5-1705:setI", "SR-PS-QS5-1706:setI", "SR-PS-QS4-1707:setI", "SR-PS-QS3-1708:setI", "SR-PS-QS2-1709:setI", "SR-PS-QS1-1710:setI", "SR-PS-QS1-1801:setI", "SR-PS-QS2-1802:setI", "SR-PS-QS3-1803:setI", "SR-PS-QS4-1804:setI", "SR-PS-QS5-1805:setI", "SR-PS-QS5-1806:setI", "SR-PS-QS4-1807:setI", "SR-PS-QS3-1808:setI", "SR-PS-QS2-1809:setI", "SR-PS-QS1-1810:setI", "SR-PS-QS1-1901:setI", "SR-PS-QS2-1902:setI", "SR-PS-QS3-1903:setI", "SR-PS-QS4-1904:setI", "SR-PS-QS5-1905:setI", "SR-PS-QS5-1906:setI", "SR-PS-QS4-1907:setI", "SR-PS-QS3-1908:setI", "SR-PS-QS2-1909:setI", "SR-PS-QS1-1910:setI", "SR-PS-QS1-2001:setI", "SR-PS-QS2-2002:setI", "SR-PS-QS3-2003:setI", "SR-PS-QS4-2004:setI", "SR-PS-QS5-2005:setI", "SR-PS-QS5-2006:setI", "SR-PS-QS4-2007:setI", "SR-PS-QL3-2008:setI", "SR-PS-QL2-2009:setI", "SR-PS-QL1-2010:setI", "SR-PS-QL1-2101:setI", "SR-PS-QL2-2102:setI", "SR-PS-QL3-2103:setI", "SR-PS-QS4-2104:setI", "SR-PS-QS5-2105:setI", "SR-PS-QS5-2106:setI", "SR-PS-QS4-2107:setI", "SR-PS-QS3-2108:setI", "SR-PS-QS2-2109:setI", "SR-PS-QS1-2110:setI", "SR-PS-QS1-2201:setI", "SR-PS-QS2-2202:setI", "SR-PS-QS3-2203:setI", "SR-PS-QS4-2204:setI", "SR-PS-QS5-2205:setI", "SR-PS-QS5-2206:setI", "SR-PS-QS4-2207:setI", "SR-PS-QS3-2208:setI", "SR-PS-QS2-2209:setI", "SR-PS-QS1-2210:setI", "SR-PS-QS1-2301:setI", "SR-PS-QS2-2302:setI", "SR-PS-QS3-2303:setI", "SR-PS-QS4-2304:setI", "SR-PS-QS5-2305:setI", "SR-PS-QS5-2306:setI", "SR-PS-QS4-2307:setI", "SR-PS-QS3-2308:setI", "SR-PS-QS2-2309:setI", "SR-PS-QS1-2310:setI", "SR-PS-QS1-2401:setI", "SR-PS-QS2-2402:setI", "SR-PS-QS3-2403:setI", "SR-PS-QS4-2404:setI", "SR-PS-QS5-2405:setI", "SR-PS-QS5-2406:setI", "SR-PS-QS4-2407:setI", "SR-PS-QL3-2408:setI", "SR-PS-QL2-2409:setI", "SR-PS-QL1-2410:setI", "SR-PS-S1-011:setI", "SR-PS-S2-012:setI", "SR-PS-SD-013:setI", "SR-PS-SF-014:setI", "SR-PS-SD-015:setI", "SR-PS-S4-016:setI", "SR-PS-S3-017:setI", "SR-PS-S5-021:setI", "SR-PS-S6-022:setI", "SR-PS-SD-023:setI", "SR-PS-SF-024:setI", "SR-PS-SD-025:setI", "SR-PS-S6-026:setI", "SR-PS-S5-027:setI", "SR-PS-S5-031:setI", "SR-PS-S6-032:setI", "SR-PS-SD-033:setI", "SR-PS-SF-034:setI", "SR-PS-SD-035:setI", "SR-PS-S6-036:setI", "SR-PS-S5-037:setI", "SR-PS-S3-041:setI", "SR-PS-S4-042:setI", "SR-PS-SD-043:setI", "SR-PS-SF-044:setI", "SR-PS-SD-045:setI", "SR-PS-S2-046:setI", "SR-PS-S1-047:setI", "SR-PS-S1-051:setI", "SR-PS-S2-052:setI", "SR-PS-SD-053:setI", "SR-PS-SF-054:setI", "SR-PS-SD-055:setI", "SR-PS-S4-056:setI", "SR-PS-S3-057:setI", "SR-PS-S5-061:setI", "SR-PS-S6-062:setI", "SR-PS-SD-063:setI", "SR-PS-SF-064:setI", "SR-PS-SD-065:setI", "SR-PS-S6-066:setI", "SR-PS-S5-067:setI", "SR-PS-S5-071:setI", "SR-PS-S6-072:setI", "SR-PS-SD-073:setI", "SR-PS-SF-074:setI", "SR-PS-SD-075:setI", "SR-PS-S6-076:setI", "SR-PS-S5-077:setI", "SR-PS-S3-081:setI", "SR-PS-S4-082:setI", "SR-PS-SD-083:setI", "SR-PS-SF-084:setI", "SR-PS-SD-085:setI", "SR-PS-S2-086:setI", "SR-PS-S1-087:setI", "SR-PS-S1-091:setI", "SR-PS-S2-092:setI", "SR-PS-SD-093:setI", "SR-PS-SF-094:setI", "SR-PS-SD-095:setI", "SR-PS-S4-096:setI", "SR-PS-S3-097:setI", "SR-PS-S5-101:setI", "SR-PS-S6-102:setI", "SR-PS-SD-103:setI", "SR-PS-SF-104:setI", "SR-PS-SD-105:setI", "SR-PS-S6-106:setI", "SR-PS-S5-107:setI", "SR-PS-S5-111:setI", "SR-PS-S6-112:setI", "SR-PS-SD-113:setI", "SR-PS-SF-114:setI", "SR-PS-SD-115:setI", "SR-PS-S6-116:setI", "SR-PS-S5-117:setI", "SR-PS-S3-121:setI", "SR-PS-S4-122:setI", "SR-PS-SD-123:setI", "SR-PS-SF-124:setI", "SR-PS-SD-125:setI", "SR-PS-S2-126:setI", "SR-PS-S1-127:setI", "SR-PS-S1-131:setI", "SR-PS-S2-132:setI", "SR-PS-SD-133:setI", "SR-PS-SF-134:setI", "SR-PS-SD-135:setI", "SR-PS-S4-136:setI", "SR-PS-S3-137:setI", "SR-PS-S5-141:setI", "SR-PS-S6-142:setI", "SR-PS-SD-143:setI", "SR-PS-SF-144:setI", "SR-PS-SD-145:setI", "SR-PS-S6-146:setI", "SR-PS-S5-147:setI", "SR-PS-S5-151:setI", "SR-PS-S6-152:setI", "SR-PS-SD-153:setI", "SR-PS-SF-154:setI", "SR-PS-SD-155:setI", "SR-PS-S6-156:setI", "SR-PS-S5-157:setI", "SR-PS-S3-161:setI", "SR-PS-S4-162:setI", "SR-PS-SD-163:setI", "SR-PS-SF-164:setI", "SR-PS-SD-165:setI", "SR-PS-S2-166:setI", "SR-PS-S1-167:setI", "SR-PS-S1-171:setI", "SR-PS-S2-172:setI", "SR-PS-SD-173:setI", "SR-PS-SF-174:setI", "SR-PS-SD-175:setI", "SR-PS-S4-176:setI", "SR-PS-S3-177:setI", "SR-PS-S5-181:setI", "SR-PS-S6-182:setI", "SR-PS-SD-183:setI", "SR-PS-SF-184:setI", "SR-PS-SD-185:setI", "SR-PS-S6-186:setI", "SR-PS-S5-187:setI", "SR-PS-S5-191:setI", "SR-PS-S6-192:setI", "SR-PS-SD-193:setI", "SR-PS-SF-194:setI", "SR-PS-SD-195:setI", "SR-PS-S6-196:setI", "SR-PS-S5-197:setI", "SR-PS-S3-201:setI", "SR-PS-S4-202:setI", "SR-PS-SD-203:setI", "SR-PS-SF-204:setI", "SR-PS-SD-205:setI", "SR-PS-S2-206:setI", "SR-PS-S1-207:setI", "SR-PS-S1-211:setI", "SR-PS-S2-212:setI", "SR-PS-SD-213:setI", "SR-PS-SF-214:setI", "SR-PS-SD-215:setI", "SR-PS-S4-216:setI", "SR-PS-S3-217:setI", "SR-PS-S5-221:setI", "SR-PS-S6-222:setI", "SR-PS-SD-223:setI", "SR-PS-SF-224:setI", "SR-PS-SD-225:setI", "SR-PS-S6-226:setI", "SR-PS-S5-227:setI", "SR-PS-S5-231:setI", "SR-PS-S6-232:setI", "SR-PS-SD-233:setI", "SR-PS-SF-234:setI", "SR-PS-SD-235:setI", "SR-PS-S6-236:setI", "SR-PS-S5-237:setI", "SR-PS-S3-241:setI", "SR-PS-S4-242:setI", "SR-PS-SD-243:setI", "SR-PS-SF-244:setI", "SR-PS-SD-245:setI", "SR-PS-S2-246:setI", "SR-PS-S1-247:setI", "SR-PS-SKEW-011:setI", "SR-PS-SKEW-012:setI", "SR-PS-SKEW-013:setI", "SR-PS-SKEW-014:setI", "SR-PS-SKEW-015:setI", "SR-PS-SKEW-016:setI", "SR-PS-SKEW-017:setI", "SR-PS-SKEW-021:setI", "SR-PS-SKEW-022:setI", "SR-PS-SKEW-023:setI", "SR-PS-SKEW-024:setI", "SR-PS-SKEW-025:setI", "SR-PS-SKEW-026:setI", "SR-PS-SKEW-027:setI", "SR-PS-SKEW-031:setI", "SR-PS-SKEW-032:setI", "SR-PS-SKEW-033:setI", "SR-PS-SKEW-034:setI", "SR-PS-SKEW-035:setI", "SR-PS-SKEW-036:setI", "SR-PS-SKEW-037:setI", "SR-PS-SKEW-041:setI", "SR-PS-SKEW-042:setI", "SR-PS-SKEW-043:setI", "SR-PS-SKEW-044:setI", "SR-PS-SKEW-045:setI", "SR-PS-SKEW-046:setI", "SR-PS-SKEW-047:setI", "SR-PS-SKEW-051:setI", "SR-PS-SKEW-052:setI", "SR-PS-SKEW-053:setI", "SR-PS-SKEW-054:setI", "SR-PS-SKEW-055:setI", "SR-PS-SKEW-056:setI", "SR-PS-SKEW-057:setI", "SR-PS-SKEW-061:setI", "SR-PS-SKEW-062:setI", "SR-PS-SKEW-063:setI", "SR-PS-SKEW-064:setI", "SR-PS-SKEW-065:setI", "SR-PS-SKEW-066:setI", "SR-PS-SKEW-067:setI", "SR-PS-SKEW-071:setI", "SR-PS-SKEW-072:setI", "SR-PS-SKEW-073:setI", "SR-PS-SKEW-074:setI", "SR-PS-SKEW-075:setI", "SR-PS-SKEW-076:setI", "SR-PS-SKEW-077:setI", "SR-PS-SKEW-081:setI", "SR-PS-SKEW-082:setI", "SR-PS-SKEW-083:setI", "SR-PS-SKEW-084:setI", "SR-PS-SKEW-085:setI", "SR-PS-SKEW-086:setI", "SR-PS-SKEW-087:setI", "SR-PS-SKEW-091:setI", "SR-PS-SKEW-092:setI", "SR-PS-SKEW-093:setI", "SR-PS-SKEW-094:setI", "SR-PS-SKEW-095:setI", "SR-PS-SKEW-096:setI", "SR-PS-SKEW-097:setI", "SR-PS-SKEW-101:setI", "SR-PS-SKEW-102:setI", "SR-PS-SKEW-103:setI", "SR-PS-SKEW-104:setI", "SR-PS-SKEW-105:setI", "SR-PS-SKEW-106:setI", "SR-PS-SKEW-107:setI", "SR-PS-SKEW-111:setI", "SR-PS-SKEW-112:setI", "SR-PS-SKEW-113:setI", "SR-PS-SKEW-114:setI", "SR-PS-SKEW-115:setI", "SR-PS-SKEW-116:setI", "SR-PS-SKEW-117:setI", "SR-PS-SKEW-121:setI", "SR-PS-SKEW-122:setI", "SR-PS-SKEW-123:setI", "SR-PS-SKEW-124:setI", "SR-PS-SKEW-125:setI", "SR-PS-SKEW-126:setI", "SR-PS-SKEW-127:setI", "SR-PS-SKEW-131:setI", "SR-PS-SKEW-132:setI", "SR-PS-SKEW-133:setI", "SR-PS-SKEW-134:setI", "SR-PS-SKEW-135:setI", "SR-PS-SKEW-136:setI", "SR-PS-SKEW-137:setI", "SR-PS-SKEW-141:setI", "SR-PS-SKEW-142:setI", "SR-PS-SKEW-143:setI", "SR-PS-SKEW-144:setI", "SR-PS-SKEW-145:setI", "SR-PS-SKEW-146:setI", "SR-PS-SKEW-147:setI", "SR-PS-SKEW-151:setI", "SR-PS-SKEW-152:setI", "SR-PS-SKEW-153:setI", "SR-PS-SKEW-154:setI", "SR-PS-SKEW-155:setI", "SR-PS-SKEW-156:setI", "SR-PS-SKEW-157:setI", "SR-PS-SKEW-161:setI", "SR-PS-SKEW-162:setI", "SR-PS-SKEW-163:setI", "SR-PS-SKEW-164:setI", "SR-PS-SKEW-165:setI", "SR-PS-SKEW-166:setI", "SR-PS-SKEW-167:setI", "SR-PS-SKEW-171:setI", "SR-PS-SKEW-172:setI", "SR-PS-SKEW-173:setI", "SR-PS-SKEW-174:setI", "SR-PS-SKEW-175:setI", "SR-PS-SKEW-176:setI", "SR-PS-SKEW-177:setI", "SR-PS-SKEW-181:setI", "SR-PS-SKEW-182:setI", "SR-PS-SKEW-183:setI", "SR-PS-SKEW-184:setI", "SR-PS-SKEW-185:setI", "SR-PS-SKEW-186:setI", "SR-PS-SKEW-187:setI", "SR-PS-SKEW-191:setI", "SR-PS-SKEW-192:setI", "SR-PS-SKEW-193:setI", "SR-PS-SKEW-194:setI", "SR-PS-SKEW-195:setI", "SR-PS-SKEW-196:setI", "SR-PS-SKEW-197:setI", "SR-PS-SKEW-201:setI", "SR-PS-SKEW-202:setI", "SR-PS-SKEW-203:setI", "SR-PS-SKEW-204:setI", "SR-PS-SKEW-205:setI", "SR-PS-SKEW-206:setI", "SR-PS-SKEW-207:setI", "SR-PS-SKEW-211:setI", "SR-PS-SKEW-212:setI", "SR-PS-SKEW-213:setI", "SR-PS-SKEW-214:setI", "SR-PS-SKEW-215:setI", "SR-PS-SKEW-216:setI", "SR-PS-SKEW-217:setI", "SR-PS-SKEW-221:setI", "SR-PS-SKEW-222:setI", "SR-PS-SKEW-223:setI", "SR-PS-SKEW-224:setI", "SR-PS-SKEW-225:setI", "SR-PS-SKEW-226:setI", "SR-PS-SKEW-227:setI", "SR-PS-SKEW-231:setI", "SR-PS-SKEW-232:setI", "SR-PS-SKEW-233:setI", "SR-PS-SKEW-234:setI", "SR-PS-SKEW-235:setI", "SR-PS-SKEW-236:setI", "SR-PS-SKEW-237:setI", "SR-PS-SKEW-241:setI", "SR-PS-SKEW-242:setI", "SR-PS-SKEW-243:setI", "SR-PS-SKEW-244:setI", "SR-PS-SKEW-245:setI", "SR-PS-SKEW-246:setI", "SR-PS-SKEW-247:setI", "SR-RF2-LLRF:setGapVoltage", "SR-RF2-LLRF:setStationPhase", "SR-RF3-LLRF:setGapVoltage", "SR-RF3-LLRF:setStationPhase", "SR-PS-DMB09-Q1:setI", "SR-PS-DMB09-Q2:setI", "SR-PS-DMB09-Q3:setI", "SR-PS-DMB25-Q1:setI", "SR-PS-DMB25-Q2:setI", "SR-PS-DMB25-Q3:setI", "SR-PS-DMB41-Q1:setI", "SR-PS-DMB41-Q2:setI", "SR-PS-DMB41-Q3:setI", "SR-PS-DMB09-HC1:setI", "SR-PS-DMB09-HC2:setI", "SR-PS-DMB09-VC1:setI", "SR-PS-DMB09-VC2:setI", "SR-PS-DMB25-HC1:setI", "SR-PS-DMB25-HC2:setI", "SR-PS-DMB25-VC1:setI", "SR-PS-DMB25-VC2:setI", "SR-PS-DMB41-HC1:setI", "SR-PS-DMB41-HC2:setI", "SR-PS-DMB41-VC1:setI", "SR-PS-DMB41-VC2:setI"]  # PV nanes(SR)
  w38 = string[] ["LTB-PS-HC-1:setI", "LTB-PS-HC-2:setI", "LTB-PS-HC-3:setI", "LTB-PS-HC-4:setI", "LTB-PS-HC-5:setI", "LTB-PS-VC-1:setI", "LTB-PS-VC-2:setI", "LTB-PS-VC-3:setI", "LTB-PS-VC-4:setI", "LTB-PS-VC-5:setI", "LTB-PS-VC-6:setI", "LTB-PS-VC-7:setI", "LTB-PS-Q1A:setI", "LTB-PS-Q1B:setI", "LTB-PS-Q1C:setI", "LTB-PS-Q2A:setI", "LTB-PS-Q2B:setI", "LTB-PS-Q2C:setI", "LTB-PS-Q3A:setI", "LTB-PS-Q3B:setI", "LTB-PS-Q4A:setI", "LTB-PS-Q4B:setI", "LTB-PS-QQ:setI", "LTB-PS-BEND-1:setI", "LTB-PS-VC-2a:setI", "LTB-PS-HC-3a:setI", "LTB-PS-HC-3b:setI", "LTB-PS-HC-4a:setI", "LTB-PS-HC-5a:setI", "LI-DI-SLIT-motor:axis2Position1", "LI-DI-SLIT-motor:axis1Position1"]  # PV nanes(LTB)
  w39 = string[] ["BTS-PS-HC-1:setI", "BTS-PS-HC-2:setI", "BTS-PS-HC-3:setI", "BTS-PS-HC-4:setI", "BTS-PS-HC-5:setI", "BTS-PS-VC-2:setI", "BTS-PS-VC-3:setI", "BTS-PS-VC-4:setI", "BTS-PS-VC-5:setI", "BTS-PS-VC-6:setI", "BTS-PS-Q1A:setI", "BTS-PS-Q1B:setI", "BTS-PS-Q1C:setI", "BTS-PS-Q2A:setI", "BTS-PS-Q2B:setI", "BTS-PS-Q2C:setI", "BTS-PS-Q3A:setI", "BTS-PS-BEND-1:setI", "BTS-PS-BEND-2:setI", "BR-PS-EXT-K1:setHV", "BR-PS-EXT-K2:setHV", "SR-PS-INJ-SE1:setHV", "SR-PS-INJ-SE2:setHV", "SR-PS-INJ-K1:setHV", "SR-PS-INJ-K2:setHV", "SR-PS-INJ-K3:setHV", "SR-PS-INJ-K4:setHV", "CPCIPM-TI-EVR:Pulse4DelaySet", "CPCIPM-TI-EVR:Pulse5DelaySet", "CPCIPM-TI-EVR:Pulse3DelaySet", "CPCIPM-TI-EVR:Pulse6DelaySet", "CPCIPM-TI-EVR:Pulse7DelaySet", "T560:setADelay", "T560:setBDelay", "T560:setCDelay", "T560:setDDelay", "CPCIPM-TI-EVR:Pulse4DelaySet", "CPCIPM-TI-EVR:Pulse5DelaySet", "BR-PS-EXT-SE1:setHV", "BR-PS-EXT-SE2:setHV", "CPCIPM-TI-EVR:Pulse3DelaySet", "CPCIPM-TI-EVR:Pulse11DelaySet"]  # PV nanes(BTS)
  w42 = FALSE ("Trip Evt B")
  (unwired) string[] ["FE-DI-XBPM-051:SA:SA_X_MONITOR", "FE-DI-XBPM-051:SA:SA_Y_MONITOR", "FE-DI-XBPM-091:SA:SA_X_MONITOR", "FE-DI-XBPM-091:SA:SA_Y_MONITOR", "FE-DI-XBPM-211:SA:SA_X_MONITOR", "FE-DI-XBPM-211:SA:SA_Y_MONITOR", "FE-DI-XBPM-231:SA:SA_X_MONITOR", "FE-DI-XBPM-231:SA:SA_Y_MONITOR", "FE-DI-XBPM-251:SA:SA_X_MONITOR", "FE-DI-XBPM-251:SA:SA_Y_MONITOR", "FE-DI-XBPM-411:SA:SA_X_MONITOR", "FE-DI-XBPM-411:SA:SA_Y_MONITOR", "FE-DI-XBPM-451:SA:SA_X_MONITOR", "FE-DI-XBPM-451:SA:SA_Y_MONITOR"]
  (unwired) string[] ["SR-DI-SOFB-H:getStatus", "SR-DI-SOFB-V:getStatus", "IGPF:TPSX:FBCTRL", "IGPF:TPSY:FBCTRL", "SR-DI-FOFB-H:getStatus", "SR-DI-FOFB-V:getStatus"]
  # "TI-INJ-PROC:TimeToNextInjSec"
  # "V1.4.5 \n修改shift register 儲存筆數上限(之前沒有)，改成5000\n增加fill pattern的gap值\n檢查處加入ID 的mode"
  # "這3個變動太頻繁，不紀錄"
  # "PV nanes(ID gap_phase_Taper_)"
  # "PV nanes(Feedback_ILK)"
  # "V1.4.2 改成直接用最大最小值當作scale的最大最小值"
  # "1.4.1\n將BeamCurrent 圖形的Y軸上下限\n改成取最大值的1.01倍，再無條件進位取整數\n最小值的0.99倍，再無條件捨去取整數"
  # "FE-DI-XBPM-051:SA:SA_Y_MONITOR"
  # "FE-DI-XBPM-051:SA:SA_X_MONITOR"
  # "TPS-SR-052:bpm4:ilk:enabled"
  # "0 為OPEN"
  n1 = local read "last ? Hrs"() -> (w52:dbl)
  n2 = Multiply(x=3600.0 ("y"), y=w52) -> (x*y=w76:dbl)
  n3 = Get Date/Time In Seconds() -> (seconds since 1Jan1904=w47:timestamp)
  n4 = Subtract(x=w47, y=w76) -> (x-y=w46:timestamp)
  n5 = call "TimeToString.vi"("Time Stamp Control"=w47) -> ("result string"=w78:string)
  n6 = call "TimeToString.vi"("Time Stamp Control"=w46) -> ("result string"=w77:string)
  n7 = call <vilib>:"Application Directory.vi"() -> ("Application Directory"=w79:path)
  n8 = Build Path(base path=w79, name or relative path="DSN\\172-18-0-32.dsn") -> (appended path=w81:path)
  n9 = call-poly <vilib>:"DB Tools Open Connection.vi"("connection information"=w81) -> ("error out"=w70:errorcluster, "connection reference"=w69:T2)  [unwired: 7 in]
  n10 = Concatenate Strings("SELECT  float_val , smpl_time\nFROM sample \nwhere  channel_id = 104 and smpl_time between '" ("result string"), w77, "' ::timestamp and '" ("result string"), w78, "' ::timestamp" ("result string")) -> (w54:string)
  n11 = call-poly <vilib>:"DB Tools Execute Query.vi"("error in (no error)"=w70, "SQL query"=w54, "connection reference"=w69) -> ("error out"=w67:errorcluster, "recordset reference"=w68:T3)  [unwired: 5 in]
  n12 = call-poly <vilib>:"DB Tools Fetch Recordset Data.vi"("error in (no error)"=w67, "recordset reference"=w68) -> ("error out"=w65:errorcluster, "recordset data"=w62:variant[][], "recordset reference out"=w66:T3)  [unwired: 3 in]
  n13 = call-poly <vilib>:"DB Tools Free Object.vi"("error in (no error)"=w65, "recordset reference"=w66) -> ("error out"=w63:errorcluster, "connection reference"=w64:T2)  [unwired: 8 in]
  n14 = Variant To Data(type=string[][] [], Variant=w62) -> (data=w60:string[][])  [unwired: 1 in, 1 out]
  n15 = call <vilib>:"DB Tools Close Connection.vi"("error in (no error)"=w63, "connection reference"=w64) -> ()  [unwired: 5 in, 1 out]
  n16 = Transpose 2D Array(2D array=w60) -> (transposed array=w58:string[][])
  n17 = Index Array(array=w58, index (row) #1=0 ("index (row)"), index (row) #2=1 ("index (row)")) -> (element #1=w72:string[], element #2=w74:string[])  [unwired: 2 in]
  n18 = Fract/Exp String To Number(string=w72) -> (number=w48:dbl[])  [unwired: 3 in, 1 out]
  n19 = Array Max & Min(array=w48) -> (max value=w44:dbl, min value=w43:dbl)  [unwired: 2 out]
  n20 = for {
    tunnel: w74 -> [w85] mode=indexing
    tunnel: [w84] -> w73 mode=indexing
    n21 = Scan From String "Scan From String"(format string="%<%Y/%m/%d %p %I:%M:%S>T", input string=w85, initial scan location=u32 0, default 1=timestamp(-73814400 s since 1904-01-01)) -> (output 1=w88:timestamp)  [unwired: 1 in, 3 out]
    n22 = To Double Precision Float(number=w88) -> (double precision float=w84:dbl)
  }
  n23 = To Double Precision Float(number=w47) -> (double precision float=w50:dbl)
  n24 = To Double Precision Float(number=w46) -> (double precision float=w49:dbl)
  n25 = control-ref of="BeamCurrent History"() -> (w51:refnum<vi>)
  n26 = property on="Property Node" class="XYGraph (strict)"(reference=w51, "XScale.Maximum"=w50, "XScale.Minimum"=w49, "YScale.Maximum"=w44, "YScale.Minimum"=w43) -> ()  [unwired: 1 in, 2 out]
  n27 = local write "Refresh B"(w42) -> ()
  n28 = local write "Trip Evt B"(w42) -> ()
  n29 = Bundle(w73, w48) -> (w53:cluster{dbl[], dbl[]})  [unwired: 1 in]
  n30 = property on="result" class="Str"("Visible"=FALSE) -> ()  [unwired: 2 in, 2 out]
  n31 = Build Array (concatenate)(w31, w32, w27) -> (w30:string[])
  n32 = disable-structure shown="Disabled" {
    frame Disabled {
      (unwired) string[] ["TI-INJ-PROC:TopupHiLowStart", "SR-DI-DCCT:BeamCurrent", "SR-DI-DCCT:BeamLifetime", "SR-DI-XPC-40:SigmaX", "SR-DI-XPC-40:SigmaY", "SR-DI-TUNE:nux", "SR-DI-TUNE:nuy", "IGPF:TPSX:SRAM:VEC:PEAKFREQ2", "IGPF:TPSY:SRAM:VEC:PEAKFREQ2", "TI-INJ-PROC:setBucketAddressStart", "TI-INJ-PROC:setBucketAddressLast", "TI-INJ-PROC:setBucketAddressStep"]
      # "before 20180201"
    }
    frame Enabled {
    }
  }
  n33 = Build Array (concatenate)(w25, w38, w24, w39, w40, w30, string[] ["SR-DI-FOFB-H:setStatus", "SR-DI-FOFB-V:setStatus", "IGPF:TPSX:FBCTRL", "IGPF:TPSY:FBCTRL", "TPS-SR-022:bpm3:ilk:enabled", "SR-DI-ANGLE-ILK:StatusX", "SR-DI-ANGLE-ILK:StatusY", "SR-DI-RF-FB:setStatus", "SR-ID-EPU48-TFF:status", "SR-ID-EPU48-CFF:status", "SR-ID-EPU46-TFF:status", "SR-ID-EPU46-CFF:status"], w26, w29, w28) -> (w41:string[])
  "PV list" <- w41
  n34 = call <vilib>:"Application Directory.vi"() -> ("Application Directory"=w8:path)
  n35 = Get Date/Time In Seconds() -> (seconds since 1Jan1904=w35:timestamp)
  n36 = Build Path(base path=w8, name or relative path="musics") -> (appended path=w20:path)
  n37 = To Double Precision Float(number=w35) -> (double precision float=w33:dbl)
  "Program Start Time" <- w33
  n38 = while {
    shift-right: [w269] -> _
    shift-left: _ -> [w267]
    shift-right: [w268] -> _
    shift-left: _ -> [w266]
    shift-right: [w137] -> _
    shift-left: w53 -> [w136]
    tunnel: w33 -> [w132]
    shift-right: [w114] -> _
    shift-left: _ -> [w115]
    shift-right: [w96] -> _
    shift-left: _ -> [w97]
    shift-right: [w91] -> _
    shift-left: 0 ("index") -> [w94]
    stop <- "stop" stop-if-true
    (unwired) "TPS-SR-022:bpm3:ilk:enabled"
    (unwired) string[] ["Event Time      ", "PV_name        ", "Ori_Value", "New_Value "] ("diff_Value")
    w131 = dbl[] [1.0, 1.1666666666666667, 1.3333333333333333, 1.5, 1.6666666666666665, 1.8333333333333333, 2.0, 2.142857142857143, 2.2857142857142856, 2.4285714285714284, 2.571428571428571, 2.7142857142857144, 2.857142857142857, 3.0, 3.142857142857143, 3.2857142857142856, 3.4285714285714284, 3.571428571428571, 3.7142857142857144, 3.857142857142857, 4.0, 4.125, 4.25, 4.375, 4.5, 4.625, 4.75, 4.875, 5.0, 5.125, 5.25, 5.375, 5.5, 5.625, 5.75, 5.875, 6.0, 6.142857142857143, 6.285714285714286, 6.428571428571429, 6.571428571428571, 6.714285714285714, 6.857142857142857, 7.0, 7.142857142857143, 7.285714285714286, 7.428571428571429, 7.571428571428571, 7.714285714285714, 7.857142857142857, 8.0, 8.142857142857142, 8.285714285714286, 8.428571428571429, 8.571428571428571, 8.714285714285714, 8.857142857142858, 9.0, 9.142857142857142, 9.285714285714286, 9.428571428571429, 9.571428571428571, 9.714285714285714, 9.857142857142858, 10.0, 10.142857142857142, 10.285714285714286, 10.428571428571429, 10.571428571428571, 10.714285714285714, 10.857142857142858, 11.0, 11.142857142857142, 11.285714285714286, 11.428571428571429, 11.571428571428571, 11.714285714285714, 11.857142857142858, 12.0, 12.125, 12.25, 12.375, 12.5, 12.625, 12.75, 12.875, 13.0, 13.125, 13.25, 13.375, 13.5, 13.625, 13.75, 13.875, 14.0, 14.142857142857142, 14.285714285714286, 14.428571428571429, 14.571428571428571, 14.714285714285714, 14.857142857142858, 15.0, 15.142857142857142, 15.285714285714286, 15.428571428571429, 15.571428571428571, 15.714285714285714, 15.857142857142858, 16.0, 16.142857142857142, 16.285714285714285, 16.428571428571427, 16.571428571428573, 16.714285714285715, 16.857142857142858, 17.0, 17.142857142857142, 17.285714285714285, 17.428571428571427, 17.571428571428573, 17.714285714285715, 17.857142857142858, 18.0, 18.142857142857142, 18.285714285714285, 18.428571428571427, 18.571428571428573, 18.714285714285715, 18.857142857142858, 19.0, 19.142857142857142, 19.285714285714285, 19.428571428571427, 19.571428571428573, 19.714285714285715, 19.857142857142858, 20.0, 20.125, 20.25, 20.375, 20.5, 20.625, 20.75, 20.875, 21.0, 21.125, 21.25, 21.375, 21.5, 21.625, 21.75, 21.875, 22.0, 22.142857142857142, 22.285714285714285, 22.428571428571427, 22.571428571428573, 22.714285714285715, 22.857142857142858, 23.0, 23.142857142857142, 23.285714285714285, 23.428571428571427, 23.571428571428573, 23.714285714285715, 23.857142857142858, 24.0, 24.166666666666668, 24.333333333333332, 24.5, 24.666666666666668, 24.833333333333332]  # Array of X axis  平均分配至各段
    w162 = string[] ["SR-ID-IU22-05:setECMode", "SR-ID-IU22A-09:setECMode", "SR-ID-IU22B-09:setECMode", "SR-ID-IUT22-21:setECMode", "SR-ID-IU22-23:setECMode", "SR-ID-IU22A-25:setECMode", "SR-ID-IU22B-25:setECMode", "SR-ID-EPU48A-41:setECMode", "SR-ID-EPU48B-41:setECMode", "SR-ID-EPU46-45:setECMode"]  # ID_mode
    w248 = string[] ["FE-05-PAB:Open", "FE-05-MGV:Open", "FE-05-FCV:Open", "FE-09-PAB:Open", "FE-09-MGV:Open", "FE-09-FCV:Open", "FE-21-PAB:Open", "FE-21-MGV:Open", "FE-21-FCV:Open", "FE-23-PAB:Open", "FE-23-PAB:Open", "FE-23-FCV:Open", "FE-25-PAB:Open", "FE-25-MGV:Open", "FE-25-FCV:Open", "FE-41-PAB:Open", "FE-41-MGV:Open", "FE-41-FCV:Open", "FE-45-PAB:Open", "FE-45-MGV:Open", "FE-45-FCV:Open"]  # PAB_MGV_FCV enable
    (unwired) "LI-DI-WCM:getWfCh1"
    (unwired) "SR-DI-FP:CurrentBuffer"
    w381 = 0.001
    w379 = string[] ["SR-DI-BPM-011:Y", "SR-DI-BPM-012:Y", "SR-DI-BPM-013:Y", "SR-DI-BPM-014:Y", "SR-DI-BPM-015:Y", "SR-DI-BPM-016:Y", "SR-DI-BPM-017:Y", "SR-DI-BPM-021:Y", "SR-DI-BPM-022:Y", "SR-DI-BPM-023:Y", "SR-DI-BPM-024:Y", "SR-DI-BPM-025:Y", "SR-DI-BPM-026:Y", "SR-DI-BPM-027:Y", "SR-DI-BPM-031:Y", "SR-DI-BPM-032:Y", "SR-DI-BPM-033:Y", "SR-DI-BPM-034:Y", "SR-DI-BPM-035:Y", "SR-DI-BPM-036:Y", "SR-DI-BPM-037:Y", "SR-DI-BPM-041:Y", "SR-DI-BPM-042:Y", "SR-DI-BPM-043:Y", "SR-DI-BPM-044:Y", "SR-DI-BPM-045:Y", "SR-DI-BPM-046:Y", "SR-DI-BPM-047:Y", "SR-DI-BPM-048:Y", "SR-DI-BPM-050:Y", "SR-DI-BPM-051:Y", "SR-DI-BPM-052:Y", "SR-DI-BPM-053:Y", "SR-DI-BPM-054:Y", "SR-DI-BPM-055:Y", "SR-DI-BPM-056:Y", "SR-DI-BPM-057:Y", "SR-DI-BPM-061:Y", "SR-DI-BPM-062:Y", "SR-DI-BPM-063:Y", "SR-DI-BPM-064:Y", "SR-DI-BPM-065:Y", "SR-DI-BPM-066:Y", "SR-DI-BPM-067:Y", "SR-DI-BPM-071:Y", "SR-DI-BPM-072:Y", "SR-DI-BPM-073:Y", "SR-DI-BPM-074:Y", "SR-DI-BPM-075:Y", "SR-DI-BPM-076:Y", "SR-DI-BPM-077:Y", "SR-DI-BPM-081:Y", "SR-DI-BPM-082:Y", "SR-DI-BPM-083:Y", "SR-DI-BPM-084:Y", "SR-DI-BPM-085:Y", "SR-DI-BPM-086:Y", "SR-DI-BPM-087:Y", "SR-DI-BPM-091:Y", "SR-DI-BPM-092:Y", "SR-DI-BPM-093:Y", "SR-DI-BPM-094:Y", "SR-DI-BPM-095:Y", "SR-DI-BPM-096:Y", "SR-DI-BPM-097:Y", "SR-DI-BPM-101:Y", "SR-DI-BPM-102:Y", "SR-DI-BPM-103:Y", "SR-DI-BPM-104:Y", "SR-DI-BPM-105:Y", "SR-DI-BPM-106:Y", "SR-DI-BPM-107:Y", "SR-DI-BPM-111:Y", "SR-DI-BPM-112:Y", "SR-DI-BPM-113:Y", "SR-DI-BPM-114:Y", "SR-DI-BPM-115:Y", "SR-DI-BPM-116:Y", "SR-DI-BPM-117:Y", "SR-DI-BPM-121:Y", "SR-DI-BPM-122:Y", "SR-DI-BPM-123:Y", "SR-DI-BPM-124:Y", "SR-DI-BPM-125:Y", "SR-DI-BPM-126:Y", "SR-DI-BPM-127:Y", "SR-DI-BPM-128:Y", "SR-DI-BPM-130:Y", "SR-DI-BPM-131:Y", "SR-DI-BPM-132:Y", "SR-DI-BPM-133:Y", "SR-DI-BPM-134:Y", "SR-DI-BPM-135:Y", "SR-DI-BPM-136:Y", "SR-DI-BPM-137:Y", "SR-DI-BPM-141:Y", "SR-DI-BPM-142:Y", "SR-DI-BPM-143:Y", "SR-DI-BPM-144:Y", "SR-DI-BPM-145:Y", "SR-DI-BPM-146:Y", "SR-DI-BPM-147:Y", "SR-DI-BPM-151:Y", "SR-DI-BPM-152:Y", "SR-DI-BPM-153:Y", "SR-DI-BPM-154:Y", "SR-DI-BPM-155:Y", "SR-DI-BPM-156:Y", "SR-DI-BPM-157:Y", "SR-DI-BPM-161:Y", "SR-DI-BPM-162:Y", "SR-DI-BPM-163:Y", "SR-DI-BPM-164:Y", "SR-DI-BPM-165:Y", "SR-DI-BPM-166:Y", "SR-DI-BPM-167:Y", "SR-DI-BPM-171:Y", "SR-DI-BPM-172:Y", "SR-DI-BPM-173:Y", "SR-DI-BPM-174:Y", "SR-DI-BPM-175:Y", "SR-DI-BPM-176:Y", "SR-DI-BPM-177:Y", "SR-DI-BPM-181:Y", "SR-DI-BPM-182:Y", "SR-DI-BPM-183:Y", "SR-DI-BPM-184:Y", "SR-DI-BPM-185:Y", "SR-DI-BPM-186:Y", "SR-DI-BPM-187:Y", "SR-DI-BPM-191:Y", "SR-DI-BPM-192:Y", "SR-DI-BPM-193:Y", "SR-DI-BPM-194:Y", "SR-DI-BPM-195:Y", "SR-DI-BPM-196:Y", "SR-DI-BPM-197:Y", "SR-DI-BPM-201:Y", "SR-DI-BPM-202:Y", "SR-DI-BPM-203:Y", "SR-DI-BPM-204:Y", "SR-DI-BPM-205:Y", "SR-DI-BPM-206:Y", "SR-DI-BPM-207:Y", "SR-DI-BPM-208:Y", "SR-DI-BPM-210:Y", "SR-DI-BPM-211:Y", "SR-DI-BPM-212:Y", "SR-DI-BPM-213:Y", "SR-DI-BPM-214:Y", "SR-DI-BPM-215:Y", "SR-DI-BPM-216:Y", "SR-DI-BPM-217:Y", "SR-DI-BPM-221:Y", "SR-DI-BPM-222:Y", "SR-DI-BPM-223:Y", "SR-DI-BPM-224:Y", "SR-DI-BPM-225:Y", "SR-DI-BPM-226:Y", "SR-DI-BPM-227:Y", "SR-DI-BPM-231:Y", "SR-DI-BPM-232:Y", "SR-DI-BPM-233:Y", "SR-DI-BPM-234:Y", "SR-DI-BPM-235:Y", "SR-DI-BPM-236:Y", "SR-DI-BPM-237:Y", "SR-DI-BPM-241:Y", "SR-DI-BPM-242:Y", "SR-DI-BPM-243:Y", "SR-DI-BPM-244:Y", "SR-DI-BPM-245:Y", "SR-DI-BPM-246:Y", "SR-DI-BPM-247:Y"]  # sorted BPMY_174
    w378 = string[] ["SR-DI-BPM-011:X", "SR-DI-BPM-012:X", "SR-DI-BPM-013:X", "SR-DI-BPM-014:X", "SR-DI-BPM-015:X", "SR-DI-BPM-016:X", "SR-DI-BPM-017:X", "SR-DI-BPM-021:X", "SR-DI-BPM-022:X", "SR-DI-BPM-023:X", "SR-DI-BPM-024:X", "SR-DI-BPM-025:X", "SR-DI-BPM-026:X", "SR-DI-BPM-027:X", "SR-DI-BPM-031:X", "SR-DI-BPM-032:X", "SR-DI-BPM-033:X", "SR-DI-BPM-034:X", "SR-DI-BPM-035:X", "SR-DI-BPM-036:X", "SR-DI-BPM-037:X", "SR-DI-BPM-041:X", "SR-DI-BPM-042:X", "SR-DI-BPM-043:X", "SR-DI-BPM-044:X", "SR-DI-BPM-045:X", "SR-DI-BPM-046:X", "SR-DI-BPM-047:X", "SR-DI-BPM-048:X", "SR-DI-BPM-050:X", "SR-DI-BPM-051:X", "SR-DI-BPM-052:X", "SR-DI-BPM-053:X", "SR-DI-BPM-054:X", "SR-DI-BPM-055:X", "SR-DI-BPM-056:X", "SR-DI-BPM-057:X", "SR-DI-BPM-061:X", "SR-DI-BPM-062:X", "SR-DI-BPM-063:X", "SR-DI-BPM-064:X", "SR-DI-BPM-065:X", "SR-DI-BPM-066:X", "SR-DI-BPM-067:X", "SR-DI-BPM-071:X", "SR-DI-BPM-072:X", "SR-DI-BPM-073:X", "SR-DI-BPM-074:X", "SR-DI-BPM-075:X", "SR-DI-BPM-076:X", "SR-DI-BPM-077:X", "SR-DI-BPM-081:X", "SR-DI-BPM-082:X", "SR-DI-BPM-083:X", "SR-DI-BPM-084:X", "SR-DI-BPM-085:X", "SR-DI-BPM-086:X", "SR-DI-BPM-087:X", "SR-DI-BPM-091:X", "SR-DI-BPM-092:X", "SR-DI-BPM-093:X", "SR-DI-BPM-094:X", "SR-DI-BPM-095:X", "SR-DI-BPM-096:X", "SR-DI-BPM-097:X", "SR-DI-BPM-101:X", "SR-DI-BPM-102:X", "SR-DI-BPM-103:X", "SR-DI-BPM-104:X", "SR-DI-BPM-105:X", "SR-DI-BPM-106:X", "SR-DI-BPM-107:X", "SR-DI-BPM-111:X", "SR-DI-BPM-112:X", "SR-DI-BPM-113:X", "SR-DI-BPM-114:X", "SR-DI-BPM-115:X", "SR-DI-BPM-116:X", "SR-DI-BPM-117:X", "SR-DI-BPM-121:X", "SR-DI-BPM-122:X", "SR-DI-BPM-123:X", "SR-DI-BPM-124:X", "SR-DI-BPM-125:X", "SR-DI-BPM-126:X", "SR-DI-BPM-127:X", "SR-DI-BPM-128:X", "SR-DI-BPM-130:X", "SR-DI-BPM-131:X", "SR-DI-BPM-132:X", "SR-DI-BPM-133:X", "SR-DI-BPM-134:X", "SR-DI-BPM-135:X", "SR-DI-BPM-136:X", "SR-DI-BPM-137:X", "SR-DI-BPM-141:X", "SR-DI-BPM-142:X", "SR-DI-BPM-143:X", "SR-DI-BPM-144:X", "SR-DI-BPM-145:X", "SR-DI-BPM-146:X", "SR-DI-BPM-147:X", "SR-DI-BPM-151:X", "SR-DI-BPM-152:X", "SR-DI-BPM-153:X", "SR-DI-BPM-154:X", "SR-DI-BPM-155:X", "SR-DI-BPM-156:X", "SR-DI-BPM-157:X", "SR-DI-BPM-161:X", "SR-DI-BPM-162:X", "SR-DI-BPM-163:X", "SR-DI-BPM-164:X", "SR-DI-BPM-165:X", "SR-DI-BPM-166:X", "SR-DI-BPM-167:X", "SR-DI-BPM-171:X", "SR-DI-BPM-172:X", "SR-DI-BPM-173:X", "SR-DI-BPM-174:X", "SR-DI-BPM-175:X", "SR-DI-BPM-176:X", "SR-DI-BPM-177:X", "SR-DI-BPM-181:X", "SR-DI-BPM-182:X", "SR-DI-BPM-183:X", "SR-DI-BPM-184:X", "SR-DI-BPM-185:X", "SR-DI-BPM-186:X", "SR-DI-BPM-187:X", "SR-DI-BPM-191:X", "SR-DI-BPM-192:X", "SR-DI-BPM-193:X", "SR-DI-BPM-194:X", "SR-DI-BPM-195:X", "SR-DI-BPM-196:X", "SR-DI-BPM-197:X", "SR-DI-BPM-201:X", "SR-DI-BPM-202:X", "SR-DI-BPM-203:X", "SR-DI-BPM-204:X", "SR-DI-BPM-205:X", "SR-DI-BPM-206:X", "SR-DI-BPM-207:X", "SR-DI-BPM-208:X", "SR-DI-BPM-210:X", "SR-DI-BPM-211:X", "SR-DI-BPM-212:X", "SR-DI-BPM-213:X", "SR-DI-BPM-214:X", "SR-DI-BPM-215:X", "SR-DI-BPM-216:X", "SR-DI-BPM-217:X", "SR-DI-BPM-221:X", "SR-DI-BPM-222:X", "SR-DI-BPM-223:X", "SR-DI-BPM-224:X", "SR-DI-BPM-225:X", "SR-DI-BPM-226:X", "SR-DI-BPM-227:X", "SR-DI-BPM-231:X", "SR-DI-BPM-232:X", "SR-DI-BPM-233:X", "SR-DI-BPM-234:X", "SR-DI-BPM-235:X", "SR-DI-BPM-236:X", "SR-DI-BPM-237:X", "SR-DI-BPM-241:X", "SR-DI-BPM-242:X", "SR-DI-BPM-243:X", "SR-DI-BPM-244:X", "SR-DI-BPM-245:X", "SR-DI-BPM-246:X", "SR-DI-BPM-247:X"]  # sorted BPMX_174
    w437 = string[] ["BL-05A:HutchA_Enable", "BL-09A:HutchA_Enable", "BL-21A:HutchA_Enable", "BL-23A:HutchA_Enable", "BL-25A:HutchA_Enable", "BL-41A:HutchA_Enable", "BL-45A:HutchA_Enable"]  # Hutch enable
    w456 = string[] ["CPCI03-adl7452-0:doBank0Ch5", "CPCI05-adl7452-0:doBank0Ch5", "CPCI11-adl7452-0:doBank0Ch5", "CPCI12-adl7452-0:doBank0Ch5", "CPCI13-adl7452-0:doBank0Ch5", "CPCI21-adl7452-0:doBank0Ch5", "CPCI23-adl7452-0:doBank0Ch5"]  # FE enable
    w533 = 578.303 ("y")
    w538 = 1.202 ("y")
    # "20180208_\norbit ilk改名稱\n原：TPS-SR-022:bpm3:ilk:enabled\n現在：TPS-SR-022:bpm3:ilk:enabled_mon"
    # "每圈600ms情況下\n500圈就是5分鐘存一筆FP"
    # "SR-DI-RF-FB:getStatus"
    # "V1.4.2 改成直接用最大最小值當作scale的最大最小值"
    # "D:\\LOG運轉紀錄\\2016"
    # "45"
    # "41"
    # "25"
    # "23"
    # "21"
    # "09"
    # "05"
    # "05\n09\n21\n23\n25\n41\n45"
    # "gapMotorOff"
    n39 = Get Date/Time In Seconds() -> (seconds since 1Jan1904=w384:timestamp)
    n40 = event shown="[7] \"View Diff Button\": Value Change" {
      selector: _ -> [_ _ _ _ _ _ _ _ _ _ _]
      dyn-events: _ -> [_ _ _ _ _ _ _ _ _ _ _]
      timeout: 233 -> [_ _ _ _ _ _ _ _ _ _ _]
      tunnel: [_ w626 _ _ _ _ _ _ _ _ _] -> w138
      tunnel: [w612 w625 w632 w646 w683 w690 w717 w729 w755 w786 w807] -> w137
      tunnel: w136 -> [w612 w625 w632 _ w683 _ w717 w729 w755 w786 w807]
      tunnel: "last ? Hrs" -> [_ _ _ w653 _ w691 _ _ _ _ _]
      tunnel: w132 -> [_ w613 _ _ _ _ _ w728 _ w780 w791]
      tunnel: "T:Slow\nF:Fast" -> [_ _ _ w649 _ w686 _ _ _ _ _]
      tunnel: 0.004 ("最新時間") -> [_ _ _ w648 _ w685 _ _ _ _ _]
      event Timeout {
        n41 = event-data() -> ()  [unwired: 1 in, 3 out]
      }
      event "stop": Value Change {
        n42 = event-data() -> ("NewVal"=w626:bool)  [unwired: 1 in, 3 out]
        n43 = Get Date/Time In Seconds() -> (seconds since 1Jan1904=w619:timestamp)
        n44 = To Double Precision Float(number=w619) -> (double precision float=w618:dbl)
        n45 = Subtract(x=w618, y=43200.0) -> (x-y=w615:dbl)
        n46 = call "Main_Daily_path.vi"() -> ("Directory path"=w620:path)  [unwired: 10 in, 1 out]
        n47 = Greater?(x=w615, y=w613) -> (0:w616:bool)
        n48 = Select(t=w615, s=w616, f=w613) -> ()  [unwired: 1 out]
        n49 = call "B09_Save_new_lattice_files.vi"("For Test"=TRUE, "Directory Path"=w620) -> ()  [unwired: 10 in]
        n50 = call <vilib>:"Application Directory.vi"() -> ("Application Directory"=w614:path)
        n51 = local read "Diff list"() -> (w623:string[][])
        n52 = call "B07_Save_changed_PVs.vi"("For Test"=FALSE, "想要限制的筆數"=1000, "Directory Path"=w614, "紀錄起始時間  門檻"=w613, "diff_Value 2"=w623) -> ()  [unwired: 5 in, 2 out]
      }
      event "Open Button": Value Change {
        n53 = event-data() -> ()  [unwired: 1 in, 6 out]
        n54 = call <vilib>:"Beep.vi"("use system alert? (T)"=FALSE, "duration (msec)"=u32 40, "frequency (Hz)"=u32 1700) -> ()  [unwired: 9 in]
        n55 = call "Main_Daily_path.vi"() -> ("Directory path(STR)"=w631:string, "Directory path"=w630:path)  [unwired: 10 in]
        n56 = call <vilib>:"Check if File or Folder Exists.vi"("path"=w630) -> ("error out"=w636:errorcluster, "file or folder exists?"=w634:bool, "dup path"=w635:path)  [unwired: 8 in]
        n57 = case shown="False" w634 {
          tunnel: w635 -> [w643 w645]
          tunnel: w636 -> [w642 w644]
          tunnel: [w641 w645] -> _
          tunnel: [w640 w644] -> w633
          frame False {
            n58 = Create Folder(path (use dialog)=w643, error in=w642) -> (created path=w641:path, error out=w640:errorcluster)  [unwired: 1 in, 1 out]
          }
          frame True {
          }
        }
        n59 = Concatenate Strings("explorer ", w631) -> (w638:string)
        n60 = call <vilib>:"System Exec.vi"("wait until completion? (T)"=FALSE, "error in (no error)"=w633, "command line"=w638) -> ()  [unwired: 5 in, 4 out]
      }
      event "Trip Evt B": Value Change {
        n61 = event-data() -> ()  [unwired: 1 in, 1 out]
        n62 = flat-sequence {
          tunnel: w653 -> [w660]
          tunnel: [w660] -> w651
          tunnel: [w655] -> w650
          tunnel: w649 -> [w655]
          tunnel: w648 -> [w654]
          tunnel: [w654] -> w647
          tunnel: [w661] -> w652
          tunnel: w651 -> [w672]
          tunnel: w650 -> [w671]
          tunnel: w647 -> [w670]
          tunnel: [w678] -> w646
          tunnel: w652 -> [w678]
          frame #0 {
            n63 = property on="result" class="Str"("Visible"=FALSE) -> ()  [unwired: 2 in, 2 out]
            n64 = call <vilib>:"Beep.vi"("use system alert? (T)"=FALSE, "duration (msec)"=u32 40, "frequency (Hz)"=u32 1700) -> ()  [unwired: 9 in]
          }
          frame #1 {
            n65 = call "sub_plot_beamCurrent_and_trip_events.vi"("要看前幾個小時"=w672, "最新時間"=w670, "T:Slow\nF:Fast"=w671) -> ("Y min value"=w663:dbl, "Y max value"=w664:dbl, "X min value"=w665:dbl, "X max value"=w666:dbl, "BeamCurrent History"=w668:cluster{dbl[], dbl[]}[], "result"=→"result":string)  [unwired: 3 in]
            n66 = control-ref of="BeamCurrent History"() -> (w662:refnum<vi>)
            n67 = Index Array(array=w668, index=1) -> (element=w661:cluster{dbl[], dbl[]})
            n68 = property on="Property Node" class="XYGraph (strict)"(reference=w662, "XScale.Maximum"=w666, "XScale.Minimum"=w665, "YScale.Maximum"=w664, "YScale.Minimum"=w663) -> ()  [unwired: 1 in, 2 out]
          }
          frame #2 {
            n69 = local write "Trip Evt B"(FALSE ("Trip Evt B")) -> ()
            n70 = property on="result" class="Str"("Visible"=TRUE) -> ()  [unwired: 2 in, 2 out]
            n71 = call <vilib>:"Beep.vi"("use system alert? (T)"=FALSE, "duration (msec)"=u32 40, "frequency (Hz)"=u32 2000) -> ()  [unwired: 9 in]
          }
        }
      }
      event "Switch Tab": Value Change {
        n72 = event-data() -> ("NewVal"=w682:bool)  [unwired: 1 in, 1 out]
        n73 = Select(t=enum32{"_____", "           "}."_____" ("Tab Control"), s=w682, f=enum32{"_____", "           "}."           " ("Tab Control")) -> (s? t:f=→"Tab Control":enum32{"_____", "           "})
      }
      event "Refresh B": Value Change {
        n74 = event-data() -> ()  [unwired: 1 in, 6 out]
        n75 = flat-sequence {
          tunnel: w691 -> [w698]
          tunnel: [w698] -> w688
          tunnel: [w693] -> w687
          tunnel: w686 -> [w693]
          tunnel: w685 -> [w692]
          tunnel: [w692] -> w684
          tunnel: [w699] -> w689
          tunnel: w688 -> [w707]
          tunnel: w687 -> [w709]
          tunnel: w684 -> [w708]
          tunnel: [w716] -> w690
          tunnel: w689 -> [w716]
          frame #0 {
            n76 = property on="result" class="Str"("Visible"=FALSE) -> ()  [unwired: 2 in, 2 out]
            n77 = call <vilib>:"Beep.vi"("use system alert? (T)"=FALSE, "duration (msec)"=u32 40, "frequency (Hz)"=u32 1700) -> ()  [unwired: 9 in]
          }
          frame #1 {
            # "032  OPStatus    2195\n037  OPStatus    1899"
            n78 = call "sub_plot_beamCurrent_and_trip_events.vi"("要看前幾個小時"=w707, "最新時間"=w708, "T:Slow\nF:Fast"=w709) -> ("Y min value"=w703:dbl, "Y max value"=w704:dbl, "X min value"=w705:dbl, "X max value"=w706:dbl, "BeamCurrent History"=w701:cluster{dbl[], dbl[]}[], "result"=w702:string)  [unwired: 3 in]
            n79 = local write "result"(w702) -> ()
            n80 = control-ref of="BeamCurrent History"() -> (w710:refnum<vi>)
            n81 = property on="Property Node" class="XYGraph (strict)"(reference=w710, "XScale.Maximum"=w706, "XScale.Minimum"=w705, "YScale.Maximum"=w704, "YScale.Minimum"=w703) -> ()  [unwired: 1 in, 2 out]
            n82 = Index Array(array=w701, index=1) -> (element=w699:cluster{dbl[], dbl[]})
          }
          frame #2 {
            n83 = local write "Refresh B"(FALSE ("Trip Evt B")) -> ()
            n84 = property on="result" class="Str"("Visible"=TRUE) -> ()  [unwired: 2 in, 2 out]
            n85 = call <vilib>:"Beep.vi"("use system alert? (T)"=FALSE, "duration (msec)"=u32 40, "frequency (Hz)"=u32 2000) -> ()  [unwired: 9 in]
          }
        }
      }
      event "Save Lattice Button": Value Change {
        n86 = event-data() -> ()  [unwired: 1 in, 2 out]
        n87 = flat-sequence {
          frame #0 {
            n88 = call <vilib>:"Beep.vi"("use system alert? (T)"=FALSE, "duration (msec)"=u32 40, "frequency (Hz)"=u32 1700) -> ()  [unwired: 9 in]
          }
          frame #1 {
            n89 = call "Main_Daily_path.vi"() -> ("Directory path"=w721:path)  [unwired: 10 in, 1 out]
            n90 = call "B09_Save_new_lattice_files.vi"("For Test"=FALSE, "Directory Path"=w721) -> ()  [unwired: 10 in]
          }
          frame #2 {
            n91 = call <vilib>:"Beep.vi"("use system alert? (T)"=FALSE, "duration (msec)"=u32 40, "frequency (Hz)"=u32 2000) -> ()  [unwired: 9 in]
          }
        }
      }
      event "View Diff Button": Value Change {
        n92 = event-data() -> ()  [unwired: 1 in, 1 out]
        n93 = flat-sequence {
          tunnel: w728 -> [w734]
          tunnel: [w740] -> w726
          tunnel: [w745] -> w727
          tunnel: w726 -> [w745]
          tunnel: w727 -> [w747]
          frame #0 {
            # "12小時為43200sec"
            # "Save file"
            n94 = Get Date/Time In Seconds() -> (seconds since 1Jan1904=w739:timestamp)
            n95 = To Double Precision Float(number=w739) -> (double precision float=w738:dbl)
            n96 = call <vilib>:"Beep.vi"("use system alert? (T)"=FALSE, "duration (msec)"=u32 40, "frequency (Hz)"=u32 1700) -> ()  [unwired: 9 in]
            n97 = Subtract(x=w738, y=43200.0) -> (x-y=w735:dbl)
            n98 = Greater?(x=w735, y=w734) -> (0:w736:bool)
            n99 = Select(t=w735, s=w736, f=w734) -> (s? t:f=w733:dbl)
            n100 = local read "Diff list"() -> (w744:string[][])
            n101 = call "Main_Daily_path.vi"() -> ("Directory path"=w743:path)  [unwired: 10 in, 1 out]
            n102 = call "B07_Save_changed_PVs.vi"("For Test"=FALSE, "想要限制的筆數"=1000, "Directory Path"=w743, "紀錄起始時間  門檻"=w733, "diff_Value 2"=w744) -> ("saved file path"=w740:path)  [unwired: 5 in, 1 out]
          }
          frame #1 {
            # "Wait"
            n103 = Wait (ms)(milliseconds to wait=u32 300) -> ()  [unwired: 1 out]
          }
          frame #2 {
            # "Show"
            n104 = Path To String(path=w747) -> (string=w749:string)
            n105 = Concatenate Strings("explorer ", w749) -> (w748:string)
            n106 = call <vilib>:"System Exec.vi"("command line"=w748) -> ()  [unwired: 7 in, 4 out]
          }
          frame #3 {
            n107 = local write "View Diff Button"(FALSE ("View Diff Button")) -> ()
            n108 = call <vilib>:"Beep.vi"("use system alert? (T)"=FALSE, "duration (msec)"=u32 40, "frequency (Hz)"=u32 2000) -> ()  [unwired: 9 in]
          }
        }
      }
      event "Show Check list Button": Value Change {
        n109 = event-data() -> ()  [unwired: 1 in, 1 out]
        n110 = flat-sequence {
          frame #0 {
            n111 = call <vilib>:"Beep.vi"("use system alert? (T)"=FALSE, "duration (msec)"=u32 40, "frequency (Hz)"=u32 1700) -> ()  [unwired: 9 in]
          }
          frame #1 {
            n112 = local read "PV list"() -> (w759:string[])
            n113 = Array Size(array=w759) -> (size(s)=w760:i32)
            n114 = Array To Spreadsheet String(delimiter (Tab)="</BR>\n\r", array=w759, 3:"%s" ("format string")) -> (spreadsheet string=w771:string)
            n115 = Number To Decimal String(number=w760) -> (decimal integer string=w770:string)  [unwired: 1 in]
            n116 = call <vilib>:"Application Directory.vi"() -> ("Application Directory"=w761:path)
            n117 = Concatenate Strings("Tatal Checked PVs: ", w770, "</BR>\n\r" ("string"), w771) -> (w772:string)
            n118 = Build Path(base path=w761, name or relative path="Checked PV list.html") -> (appended path=w773:path)
            n119 = Write to Text File(file (use dialog)=w773, text=w772) -> ()  [unwired: 2 in, 3 out]
            n120 = flat-sequence {
              tunnel: w773 -> [w775]
              tunnel: [w775] -> w774
              frame #0 {
                n121 = Wait (ms)(milliseconds to wait=u32 500) -> ()  [unwired: 1 out]
              }
            }
            n122 = Path To String(path=w774) -> (string=w764:string)
            n123 = Concatenate Strings("explorer ", w764) -> (w763:string)
            n124 = call <vilib>:"System Exec.vi"("command line"=w763) -> ()  [unwired: 7 in, 4 out]
          }
          frame #2 {
            n125 = call <vilib>:"Beep.vi"("use system alert? (T)"=FALSE, "duration (msec)"=u32 40, "frequency (Hz)"=u32 2000) -> ()  [unwired: 9 in]
          }
        }
      }
      event Panel Close? {
        n126 = event-data() -> ()  [unwired: 1 in, 4 out]
        n127 = call "Main_Daily_path.vi"() -> ("Directory path"=w782:path)  [unwired: 10 in, 1 out]
        n128 = call "B09_Save_new_lattice_files.vi"("For Test"=TRUE, "Directory Path"=w782) -> ()  [unwired: 10 in]
        n129 = call <vilib>:"Application Directory.vi"() -> ("Application Directory"=w781:path)
        n130 = local read "Diff list"() -> (w785:string[][])
        n131 = call "B07_Save_changed_PVs.vi"("For Test"=FALSE, "想要限制的筆數"=1000, "Directory Path"=w781, "紀錄起始時間  門檻"=w780, "diff_Value 2"=w785) -> ()  [unwired: 5 in, 2 out]
        n132 = event-data() -> ()  [unwired: 2 in, 1 out]
      }
      event "Save Button": Value Change {
        n133 = event-data() -> ()  [unwired: 1 in, 1 out]
        n134 = Get Date/Time In Seconds() -> (seconds since 1Jan1904=w797:timestamp)
        n135 = To Double Precision Float(number=w797) -> (double precision float=w796:dbl)
        n136 = call <vilib>:"Beep.vi"("use system alert? (T)"=FALSE, "duration (msec)"=u32 40, "frequency (Hz)"=u32 1700) -> ()  [unwired: 9 in]
        n137 = Subtract(x=w796, y=43200.0) -> (x-y=w793:dbl)
        n138 = Greater?(x=w793, y=w791) -> (0:w794:bool)
        n139 = Select(t=w793, s=w794, f=w791) -> (s? t:f=w792:dbl)
        n140 = local read "Diff list"() -> (w801:string[][])
        n141 = call "Main_Daily_path.vi"() -> ("Directory path"=w800:path)  [unwired: 10 in, 1 out]
        n142 = call "B07_Save_changed_PVs.vi"("For Test"=FALSE, "想要限制的筆數"=1000, "Directory Path"=w800, "紀錄起始時間  門檻"=w792, "diff_Value 2"=w801) -> ()  [unwired: 5 in, 2 out]
        n143 = Get Date/Time In Seconds() -> (seconds since 1Jan1904=w809:timestamp)
        n144 = Format Date/Time String(time format string (%c)="%Y", seconds (now)=w809, UTC format=FALSE) -> (date/time string=w827:string)
        n145 = Format Date/Time String(time format string (%c)="%d", seconds (now)=w809, UTC format=FALSE) -> (date/time string=w836:string)
        n146 = call "to_be_2_string.vi"("string 2"=w836) -> ("substring 2"=w837:string)  [unwired: 10 in]
        n147 = Format Date/Time String(time format string (%c)="%m", seconds (now)=w809, UTC format=FALSE) -> (date/time string=w831:string)
        n148 = Concatenate Strings("D" ("磁碟位置"), ":\\LOG運轉紀錄\\", w827, "\\", w831, "\\", w837) -> (w820:string)
        n149 = Format Date/Time String(time format string (%c)="%Y%m%d%H%M%S", seconds (now)=w809) -> (date/time string=w815:string)  [unwired: 1 in]
        n150 = String To Path(string=w820) -> (path=w823:path)
        n151 = call <vilib>:"Check if File or Folder Exists.vi"("path"=w823) -> ("error out"=w821:errorcluster, "file or folder exists?"=w835:bool, "dup path"=w822:path)  [unwired: 8 in]
        n152 = invoke on="Cluster" class="Clust (strict)" method="Get Image"() -> ("image data"=w790:T4)  [unwired: 6 in, 5 out]
        n153 = case shown="False" w835 {
          tunnel: w822 -> [w848 w850]
          tunnel: w821 -> [w847 w849]
          tunnel: [w846 w850] -> w808
          tunnel: [w845 w849] -> _
          frame False {
            n154 = Create Folder(path (use dialog)=w848, error in=w847) -> (created path=w846:path, error out=w845:errorcluster)  [unwired: 1 in, 1 out]
          }
          frame True {
          }
        }
        n155 = call "Main_Daily_path.vi"() -> ("Directory path"=w802:path)  [unwired: 10 in, 1 out]
        n156 = Path To String(path=w808) -> (string=w819:string)
        n157 = Concatenate Strings(w819, "\\" ("string"), w815) -> (w810:string)
        n158 = call "B09_Save_new_lattice_files.vi"("For Test"=FALSE, "Directory Path"=w802) -> ()  [unwired: 10 in]
        n159 = Concatenate Strings(w810, ".jpg" ("file format")) -> (w811:string)
        n160 = String To Path(string=w811) -> (path=w814:path)
        n161 = call <vilib>:"Draw Flattened Pixmap.vi"("image data"=w790) -> ("new picture"=w788:picture)  [unwired: 8 in]
        "new picture" <- w788
        n162 = call <vilib>:"Write JPEG File.vi"("quality (80)"=100, "image data"=w790, "path to JPEG file"=w814) -> ("error out"=w789:errorcluster)  [unwired: 7 in, 1 out]
        "error out 3" <- w789
        n163 = flat-sequence {
          tunnel: w789 -> [w840]
          tunnel: w788 -> [_]
          frame #0 {
            n164 = Temporary Directory() -> (w839:path)
            n165 = control-ref of="new picture"() -> (w844:refnum<vi>)
            n166 = invoke class="Pict" method="Export Image"(reference=w844, error in=w840, "File Type"=enum32{"BMP", "EPS", "EMF", "PICT"}."BMP", "Target"=enum32{"File", "Clipboard"}."Clipboard", "Path"=w839, "Hide Grid"=TRUE ("Always Overwrite")) -> (error out=→"error out":errorcluster)  [unwired: 1 in, 6 out]
          }
        }
      }
    }
    n167 = Format Date/Time String(time format string (%c)="%Y/%m/%d_%H:%M:%S", seconds (now)=w384) -> (date/time string=w89:string)  [unwired: 1 in]
    n168 = Format Date/Time String(time format string (%c)="%Y/%m/%d", seconds (now)=w384) -> (date/time string=w90:string)  [unwired: 1 in]
    "NOW date" <- w90
    n169 = Format Date/Time String(time format string (%c)="%H:%M:%S", seconds (now)=w384) -> (date/time string=w295:string)  [unwired: 1 in]
    "NOW time" <- w295
    n170 = call-poly <userlib>:"CaLabGet.vi"("PV Names"=string[] ["FE-DI-XBPM-051:signals:sa.X", "FE-DI-XBPM-051:signals:sa.Y", "FE-DI-XBPM-091:SA:SA_X_MONITOR", "FE-DI-XBPM-091:SA:SA_Y_MONITOR", "FE-DI-XBPM-211:SA:SA_X_MONITOR", "FE-DI-XBPM-211:SA:SA_Y_MONITOR", "FE-DI-XBPM-231:SA:SA_X_MONITOR", "FE-DI-XBPM-231:SA:SA_Y_MONITOR", "FE-DI-XBPM-251:SA:SA_X_MONITOR", "FE-DI-XBPM-251:SA:SA_Y_MONITOR", "FE-DI-XBPM-411:SA:SA_X_MONITOR", "FE-DI-XBPM-411:SA:SA_Y_MONITOR", "FE-DI-XBPM-451:SA:SA_X_MONITOR", "FE-DI-XBPM-451:SA:SA_Y_MONITOR", "FE-DI-XBPM-052:signals:sa.X", "FE-DI-XBPM-052:signals:sa.Y", "FE-DI-XBPM-092:SA:SA_X_MONITOR", "FE-DI-XBPM-092:SA:SA_Y_MONITOR", "FE-DI-XBPM-212:SA:SA_X_MONITOR", "FE-DI-XBPM-212:SA:SA_Y_MONITOR", "FE-DI-XBPM-232:SA:SA_X_MONITOR", "FE-DI-XBPM-232:SA:SA_Y_MONITOR", "FE-DI-XBPM-252:SA:SA_X_MONITOR", "FE-DI-XBPM-252:SA:SA_Y_MONITOR", "FE-DI-XBPM-412:SA:SA_X_MONITOR", "FE-DI-XBPM-412:SA:SA_Y_MONITOR", "FE-DI-XBPM-452:SA:SA_X_MONITOR", "FE-DI-XBPM-452:SA:SA_Y_MONITOR"] ("appended array")) -> ("1rst Value (number)"=w404:dbl[])  [unwired: 8 in, 6 out]
    n171 = Multiply(x=w404, y=0.001) -> (x*y=w403:dbl[])
    n172 = disable-structure shown="Disabled" {
      frame Disabled {
        n173 = To Long Integer() -> (32bit integer=w895:i32)  [unwired: 1 in]
        n174 = case shown="1" w895 {
          tunnel: ["Decay" "Top-Up"] -> _
          frame 0, Default {
          }
          frame 1 {
          }
        }
      }
      frame Enabled {
      }
    }
    n175 = call-poly <userlib>:"CaLabGet.vi"("PV Names"=string[] ["SR-DI-FP:CurrentBuffer", "BR-DI-FP:CurrentBuffer"]) -> ("Value Array (number)"=w474:dbl[][])  [unwired: 8 in, 6 out]
    n176 = Greater Or Equal?(x=w94, y=500) -> (x >= y?=w92:bool)
    n177 = Index Array(array=w474, index (row) #1=0 ("index"), index (row) #2=1 ("index (row)")) -> (element #1=w95:dbl[], element #2=w116:dbl[])  [unwired: 2 in]
    n178 = Index Array(array=w403, index #1=0 ("index"), index #2=1 ("index"), index #3=2 ("index"), index #4=3 ("index"), index #5=4 ("index"), index #6=5 ("index"), index #7=6 ("index"), index #8=7 ("index"), index #9=8 ("index"), index #10=9 ("index"), index #11=10 ("index"), index #12=11 ("index"), index #13=12 ("index"), index #14=13 ("index"), index #15=14 ("index"), index #16=15 ("index"), index #17=16 ("index"), index #18=17 ("index"), index #19=18 ("index"), index #20=19 ("index"), index #21=20 ("index"), index #22=21 ("index"), index #23=22 ("index"), index #24=23 ("index"), index #25=24 ("index"), index #26=25 ("index"), index #27=26 ("index"), index #28=27 ("index")) -> (element #1=w322:dbl, element #2=w315:dbl, element #3=w321:dbl, element #4=w314:dbl, element #5=w320:dbl, element #6=w313:dbl, element #7=w319:dbl, element #8=w312:dbl, element #9=w318:dbl, element #10=w311:dbl, element #11=w317:dbl, element #12=w310:dbl, element #13=w316:dbl, element #14=w309:dbl, element #15=w218:dbl, element #16=w217:dbl, element #17=w216:dbl, element #18=w215:dbl, element #19=w206:dbl, element #20=w205:dbl, element #21=w200:dbl, element #22=w199:dbl, element #23=w198:dbl, element #24=w197:dbl, element #25=w166:dbl, element #26=w165:dbl, element #27=w164:dbl, element #28=w163:dbl)
    n179 = Build Array (concatenate)(w95, w95) -> (w123:dbl[])
    n180 = for {
      tunnel: w123 -> [w610] mode=indexing
      shift-right: [w604] -> _
      shift-left: _ -> [w603]
      shift-right: [w607] -> _
      shift-left: 0 -> [w608]
      tunnel: [w605] -> w126 mode=indexing if=w598
      w609 = 0.015  # Threshold
      n181 = Increment(x=w608) -> (x+1=w605:i32)
      n182 = Less Or Equal?(x=w610, y=w609) -> (x <= y?=w604:bool)
      n183 = Not Equal?(x=w604, y=w603) -> ()  [unwired: 1 out]
      n184 = Equal?(x=w604, y=TRUE) -> (x = y?=w595:bool)
      n185 = Equal?(x=w603, y=FALSE) -> (x = y?=w594:bool)
      n186 = Equal?(x=w604, y=FALSE) -> (x = y?=w600:bool)
      n187 = Equal?(x=w603, y=TRUE) -> (x = y?=w599:bool)
      n188 = And(x=w595, y=w594) -> (x .and. y?=w593:bool)
      n189 = And(x=w600, y=w599) -> (x .and. y?=w598:bool)
      n190 = Select(t=0, s=w593, f=w605) -> (s? t:f=w607:i32)
    }
    n191 = Array Max & Min(array=w126) -> (max value=w127:i32)  [unwired: 3 out]
    n192 = case shown="True" w92 {
      selector: w92 -> [_ w565]
      tunnel: w95 -> [_ w576]
      tunnel: w94 -> [w557 _]
      tunnel: [w556 0 ("index")] -> w91
      tunnel: w89 -> [_ w571]
      frame False {
        n193 = Increment(x=w557) -> (x+1=w556:i32)
      }
      frame True {
        n194 = call "Main_Daily_path.vi"("nothing"=w565) -> ("Directory path"=w572:path)  [unwired: 9 in, 1 out]
        n195 = Number To Fractional String(number=w576, precision (6)=i16 6) -> (F-format string=w570:string[])  [unwired: 2 in]
        n196 = Build Path(base path=w572, name or relative path="Association\\" ("string")) -> (appended path=w561:path)
        n197 = Build Array (concatenate)(w571, w570) -> (w568:string[])
        n198 = call <vilib>:"Check if File or Folder Exists.vi"("path"=w561) -> ("error out"=w564:errorcluster, "file or folder exists?"=w562:bool, "dup path"=w563:path)  [unwired: 8 in]
        n199 = case shown="False" w562 {
          tunnel: w563 -> [w581 w582]
          tunnel: [w580 w583] -> _
          tunnel: w564 -> [w579 w583]
          tunnel: [w578 w582] -> w560
          frame False {
            n200 = Create Folder(path (use dialog)=w581, error in=w579) -> (created path=w578:path, error out=w580:errorcluster)  [unwired: 1 in, 1 out]
          }
          frame True {
          }
        }
        n201 = Build Path(base path=w560, name or relative path="SR_FP.csv" ("string")) -> (appended path=w558:path)
        n202 = call-poly <vilib>:"Write To Spreadsheet File.vi"("delimiter (\\t)"="," ("delimiter (\\t)"), "transpose? (no:F)"=FALSE, "format (%s)"="%s" ("format (%.3f)"), "append to file? (new file:F)"=TRUE, "1D data"=w568, "file path (dialog if empty)"=w558) -> ()  [unwired: 2 in, 1 out]
      }
    }
    n203 = Multiply(x=w127, y=2) -> (x*y=w124:i32)
    n204 = Add Array Elements(numeric array=w116) -> (sum=w119:dbl)
    n205 = call-poly <userlib>:"CaLabGet.vi"("PV Names"=string[] ["LI:restoreFilename", "LTB:restoreFilename", "BR:restoreFilename", "BTS:restoreFilename", "SR:restoreFilename"]) -> ("1rst Value (string)"=w476:string[])  [unwired: 8 in, 6 out]
    n206 = call-poly <userlib>:"CaLabGet.vi"("PV Names"=string[] ["LI-ES-CPS-01:PULSEMODE", "LI-ES-BPS-01:SETU:GRID", "LI-ES-BPS-01:SETU:MBM", "LI-ES-BPS-01:SETU:SBM", "LI-RF-HVP-31:SET:U", "CPCITM-TI-EVRTG:Pulse6DelaySet", "CPCITM-TI-EVRTG:Pulse7DelaySet", "CPCITM-TI-EVRTG:Pulse6WidthSet", "CPCITM-TI-EVRTG:Pulse7WidthSet", "CPCITM-TI-EVRTG:GTX6CtrlGTXPHSet", "CPCITM-TI-EVRTG:GTX7CtrlGTXPHSet", "CPCITM-TI-EVRTG:GTX6DlySet", "CPCITM-TI-EVRTG:GTX7DlySet"]) -> ("1rst Value (string)"=w466:string[], "1rst Value (number)"=w517:dbl[])  [unwired: 8 in, 5 out]
    n207 = call-poly <userlib>:"CaLabGet.vi"("PV Names"=string[] ["BR-PS-INJ-SE:setHV", "BR-PS-INJ-KI:setHV", "BR-PS-EXT-K1:setHV", "BR-PS-EXT-K2:setHV", "BR-PS-EXT-SE1:setHV", "BR-PS-EXT-SE2:setHV", "SR-PS-INJ-SE1:setHV", "SR-PS-INJ-SE2:setHV", "SR-PS-INJ-K1:setHV", "SR-PS-INJ-K2:setHV", "SR-PS-INJ-K3:setHV", "SR-PS-INJ-K4:setHV"]) -> ("1rst Value (number)"=w519:dbl[])  [unwired: 8 in, 6 out]
    n208 = call-poly <userlib>:"CaLabGet.vi"("PV Names"=string[] ["SR-RF-MSG:setFreq", "SR-RF2-LLRF:local", "SR-RF2-LLRF:getOperationMode", "SR-RF2-LLRF:getGapVoltage", "SR-RF2-LLRF:setGapVoltage", "SR-RF2-LLRF:setStationPhase", "SR-RF3-LLRF:local", "SR-RF3-LLRF:getOperationMode", "SR-RF3-LLRF:getGapVoltage", "SR-RF3-LLRF:setGapVoltage", "SR-RF3-LLRF:setStationPhase"]) -> ("1rst Value (number)"=w492:dbl[])  [unwired: 8 in, 6 out]
    n209 = Greater Or Equal?(x=w119, y=0.015) -> (x >= y?=w117:bool)
    n210 = call-poly <userlib>:"CaLabGet.vi"("PV Names"=string[] ["TI-INJ-PROC:TopupFixTimeStart", "SR-DI-DCCT:BeamCurrent", "SR-DI-DCCT:BeamLifetime", "SR-DI-XPC-40:SigmaX", "SR-DI-XPC-40:SigmaY", "SR-DI-TUNE:nux", "SR-DI-TUNE:nuy", "IGPF:TPSX:SRAM:VEC:PEAKFREQ2", "IGPF:TPSY:SRAM:VEC:PEAKFREQ2", "TI-INJ-PROC:setBucketAddressStart", "TI-INJ-PROC:setBucketAddressLast", "TI-INJ-PROC:setBucketAddressStep"]) -> ("1rst Value (number)"=w553:dbl[])  [unwired: 8 in, 6 out]
    n211 = Index Array(array=w466, index=0) -> (element=w464:string)
    n212 = Index Array(array=w517, index #1=0 ("index"), index #2=1 ("index"), index #3=2 ("index"), index #4=3 ("index"), index #5=4 ("index"), index #6=5 ("index"), index #7=6 ("index"), index #8=7 ("index"), index #9=8 ("index"), index #10=9 ("index"), index #11=10 ("index"), index #12=11 ("index"), index #13=12 ("index")) -> (element #2=w354:dbl, element #3=w468:dbl, element #4=w467:dbl, element #5=w352:dbl, element #8=w463:dbl, element #9=w462:dbl, element #10=w461:dbl, element #11=w460:dbl, element #12=w459:dbl, element #13=w458:dbl)  [unwired: 3 out]
    n213 = Index Array(array=w519, index #1=0 ("index"), index #2=1 ("index"), index #3=2 ("index"), index #4=3 ("index"), index #5=4 ("index"), index #6=5 ("index"), index #7=6 ("index"), index #8=7 ("index"), index #9=8 ("index"), index #10=9 ("index"), index #11=10 ("index"), index #12=11 ("index")) -> (element #1=w367:dbl, element #2=w366:dbl, element #3=w365:dbl, element #4=w364:dbl, element #5=w363:dbl, element #6=w362:dbl, element #7=w361:dbl, element #8=w360:dbl, element #9=w359:dbl, element #10=w358:dbl, element #11=w357:dbl, element #12=w356:dbl)
    n214 = Index Array(array=w492, index #1=0 ("index"), index #2=1 ("index"), index #3=2 ("index"), index #4=3 ("index"), index #5=4 ("index"), index #6=5 ("index"), index #7=6 ("index"), index #8=7 ("index"), index #9=8 ("index"), index #10=9 ("index"), index #11=10 ("index")) -> (element #1=w346:dbl, element #2=w489:dbl, element #3=w487:dbl, element #5=w272:dbl, element #6=w273:dbl, element #7=w484:dbl, element #8=w483:dbl, element #10=w342:dbl, element #11=w343:dbl)  [unwired: 2 out]
    n215 = Index Array(array=w553, index #1=0 ("index"), index #2=1 ("index"), index #3=2 ("index"), index #4=3 ("index"), index #5=4 ("index"), index #6=5 ("index"), index #7=6 ("index"), index #8=7 ("index"), index #9=8 ("index"), index #10=9 ("index"), index #11=10 ("index"), index #12=11 ("index")) -> (element #1=w551:dbl, element #2=w96:dbl, element #3=w375:dbl, element #4=w539:dbl, element #5=w537:dbl, element #6=w536:dbl, element #7=w535:dbl, element #8=w534:dbl, element #9=w532:dbl, element #10=w370:dbl, element #11=w369:dbl, element #12=w368:dbl)
    n216 = Index Array(array=w476, index #1=0 ("index"), index #2=1 ("index"), index #3=2 ("index"), index #4=3 ("index"), index #5=4 ("index")) -> (element #1=w338:string, element #2=w337:string, element #3=w341:string, element #4=w340:string, element #5=w339:string)
    n217 = call-poly <userlib>:"CaLabGet.vi"("PV Names"=w248) -> ("1rst Value (number)"=w250:dbl[])  [unwired: 8 in, 6 out]
    n218 = call-poly <userlib>:"CaLabGet.vi"("PV Names"=w437) -> ("1rst Value (string)"=w445:string[])  [unwired: 8 in, 6 out]
    n219 = To Byte Integer(number=w250) -> (8bit integer=w249:i8[])
    n220 = feedback #1() -> (w112:string)  [unwired: 1 in]
    n221 = case shown="True" w117 {
      tunnel: w116 -> [_ w592]
      tunnel: [w590 w592] -> w114
      tunnel: w115 -> [w590 _]
      tunnel: [w589 w591] -> w113
      tunnel: w112 -> [w589 _]
      frame False {
      }
      frame True {
        n222 = local read "NOW time"() -> (w591:string)
      }
    }
    n223 = feedback-in #1(w113) -> ()
    n224 = for {
      tunnel: w249 -> [w854] mode=indexing
      tunnel: [w851] -> w226 mode=indexing
      n225 = Number To Boolean Array(number=w854) -> (Boolean array=w853:bool[])
      n226 = Index Array(array=w853, index=0) -> (element=w851:bool)
    }
    n227 = for {
      tunnel: w445 -> [w864] mode=indexing
      tunnel: [w863] -> w446 mode=indexing
      n228 = case shown="\"Enable\"" w864 {
        tunnel: [FALSE TRUE] -> w863
        frame "Disable", Default {
        }
        frame "Enable" {
        }
      }
    }
    n229 = call-poly <userlib>:"CaLabGet.vi"("PV Names"=w456) -> ("1rst Value (string)"=w448:string[])  [unwired: 8 in, 6 out]
    n230 = call-poly <userlib>:"CaLabGet.vi"("PV Names"=string[] ["SR-ID-IU22-05:getGap", "SR-ID-IU22A-09:getGap", "SR-ID-IU22B-09:getGap", "SR-ID-IUT22-21:getGap", "SR-ID-IU22-23:getGap", "SR-ID-IU22A-25:getGap", "SR-ID-IU22B-25:getGap", "SR-ID-EPU48A-41:getGap", "SR-ID-EPU48A-41:getPhase", "SR-ID-EPU48B-41:getGap", "SR-ID-EPU48B-41:getPhase", "SR-ID-EPU46-45:getGap", "SR-ID-EPU46-45:getPhase", "SR-ID-IUT22-21:getGapTaper", "SR-ID-EPU48PS-41:getGap"]) -> ("1rst Value (number)"=w436:dbl[])  [unwired: 8 in, 6 out]
    n231 = for {
      tunnel: w448 -> [w868] mode=indexing
      tunnel: [w867] -> w447 mode=indexing
      n232 = case shown="\"enable\"" w868 {
        tunnel: [FALSE TRUE] -> w867
        frame "disable", Default {
        }
        frame "enable" {
        }
      }
    }
    n233 = call-poly <userlib>:"CaLabGet.vi"("PV Names"=string[] ["SR-ID-IU22-05:gapMotorOff", "SR-ID-IU22A-09:gapMotorOff", "SR-ID-IU22B-09:gapMotorOff", "SR-ID-IUT22-21:gapMotorOff", "SR-ID-IU22-23:gapMotorOff", "SR-ID-IU22A-25:gapMotorOff", "SR-ID-IU22B-25:gapMotorOff", "SR-ID-EPU48A-41:gapMotorOff", "SR-ID-EPU48B-41:gapMotorOff", "SR-ID-EPU46-45:gapMotorOff", "SR-ID-EPU48A-41:phaseMotorOff", "SR-ID-EPU48B-41:phaseMotorOff", "SR-ID-EPU46-45:phaseMotorOff"]) -> ("1rst Value (string)"=w388:string[])  [unwired: 8 in, 6 out]
    n234 = To Long Integer(number=w551) -> (32bit integer=w554:i32)
    n235 = To Long Integer(number=w487) -> (32bit integer=w488:i32)
    n236 = To Long Integer(number=w489) -> (32bit integer=w490:i32)
    n237 = To Long Integer(number=w483) -> (32bit integer=w486:i32)
    n238 = To Long Integer(number=w484) -> (32bit integer=w485:i32)
    n239 = Index Array(array=w436, index #1=0 ("index"), index #2=1 ("index"), index #3=2 ("index"), index #4=3 ("index"), index #5=4 ("index"), index #6=5 ("index"), index #7=6 ("index"), index #8=7 ("index"), index #9=8 ("index"), index #10=9 ("index"), index #11=10 ("index"), index #12=11 ("index"), index #13=12 ("index"), index #14=13 ("index"), index #15=14 ("index")) -> (element #1=w336:dbl, element #2=w335:dbl, element #3=w334:dbl, element #4=w333:dbl, element #5=w332:dbl, element #6=w331:dbl, element #7=w330:dbl, element #8=w329:dbl, element #9=w328:dbl, element #10=w327:dbl, element #11=w326:dbl, element #12=w325:dbl, element #13=w324:dbl, element #14=w271:dbl, element #15=w323:dbl)
    n240 = for {
      tunnel: w388 -> [w860] mode=indexing
      tunnel: [w859] -> w387 mode=indexing
      n241 = case shown="\"1\", Default" w860 {
        tunnel: [FALSE TRUE] -> w859
        frame "1", Default {
        }
        frame "0" {
        }
      }
    }
    n242 = Index Array(array=w226, index #1=0 ("index"), index #2=1 ("index"), index #3=2 ("index"), index #4=3 ("index"), index #5=4 ("index"), index #6=5 ("index"), index #7=6 ("index"), index #8=7 ("index"), index #9=8 ("index"), index #10=9 ("index"), index #11=10 ("index"), index #12=11 ("index"), index #13=12 ("index"), index #14=13 ("index"), index #15=14 ("index"), index #16=15 ("index"), index #17=16 ("index"), index #18=17 ("index"), index #19=18 ("index"), index #20=19 ("index"), index #21=20 ("index")) -> (element #1=w223:bool, element #2=w222:bool, element #3=w221:bool, element #4=w210:bool, element #5=w209:bool, element #6=w208:bool, element #7=w203:bool, element #8=w202:bool, element #9=w201:bool, element #10=w192:bool, element #11=w191:bool, element #12=w190:bool, element #13=w185:bool, element #14=w184:bool, element #15=w183:bool, element #16=w182:bool, element #17=w181:bool, element #18=w180:bool, element #19=w179:bool, element #20=w178:bool, element #21=w177:bool)
    n243 = case shown="1" w490 {
      tunnel: [FALSE TRUE] -> w348
      frame 0, Default {
      }
      frame 1 {
      }
    }
    n244 = case shown="1" w485 {
      tunnel: [FALSE TRUE] -> w345
      frame 0, Default {
      }
      frame 1 {
      }
    }
    n245 = case shown="0" w488 {
      tunnel: [TRUE FALSE] -> w347
      frame 0 {
      }
      frame 1, Default {
      }
    }
    n246 = case shown="0" w486 {
      tunnel: [TRUE FALSE] -> w344
      frame 0 {
      }
      frame 1, Default {
      }
    }
    n247 = case shown="1" w554 {
      tunnel: ["Decay" "Top-up(time)"] -> w376
      frame 0, Default {
      }
      frame 1 {
      }
    }
    n248 = Negate(x=w271) -> (-x=w270:dbl)
    n249 = Index Array(array=w446, index #1=0 ("index"), index #2=1 ("index"), index #3=2 ("index"), index #4=3 ("index"), index #5=4 ("index"), index #6=5 ("index"), index #7=6 ("index")) -> (element #1=w224:bool, element #2=w220:bool, element #3=w204:bool, element #4=w187:bool, element #5=w186:bool, element #6=w168:bool, element #7=w167:bool)
    n250 = case shown="\"MBM\", Default" w464 {
      tunnel: ["MBM" "SBM"] -> w355
      tunnel: w468 -> [w874 _]
      tunnel: [w874 w879] -> w353
      tunnel: w467 -> [_ w879]
      tunnel: w463 -> [_ w878]
      tunnel: w462 -> [w873 _]
      tunnel: [w873 w878] -> w351
      tunnel: w461 -> [_ w877]
      tunnel: w460 -> [w872 _]
      tunnel: [w872 w877] -> w350
      tunnel: w459 -> [_ w876]
      tunnel: w458 -> [w871 _]
      tunnel: [w871 w876] -> w349
      frame "MBM", Default {
      }
      frame "SBM" {
      }
    }
    n251 = Multiply(x=w539, y=w538) -> (x*y=w374:dbl)
    n252 = Divide(x=w534, y=w533) -> (x/y=w372:dbl)
    n253 = Multiply(x=w537, y=w538) -> (x*y=w373:dbl)
    n254 = Divide(x=w532, y=w533) -> (x/y=w371:dbl)
    n255 = Index Array(array=w447, index #1=0 ("index"), index #2=1 ("index"), index #3=2 ("index"), index #4=3 ("index"), index #5=4 ("index"), index #6=5 ("index"), index #7=6 ("index")) -> (element #1=w225:bool, element #2=w219:bool, element #3=w207:bool, element #4=w189:bool, element #5=w188:bool, element #6=w170:bool, element #7=w169:bool)
    n256 = call "FE_PAB_OpenState.vi"("FE"=w225, "XBPMX 2"=w218, "XBPMY 2"=w217, "Hutch"=w224, "PAB"=w223, "MGV"=w222, "FCV"=w221) -> ("XBPMX 2"=w214:string, "XBPMY 2"=w213:string)  [unwired: 7 in]
    n257 = call "FE_PAB_OpenState.vi"("FE"=w219, "XBPMX 2"=w216, "XBPMY 2"=w215, "Hutch"=w220, "PAB"=w210, "MGV"=w209, "FCV"=w208) -> ("XBPMX 2"=w212:string, "XBPMY 2"=w211:string)  [unwired: 7 in]
    n258 = call-poly <userlib>:"CaLabGet.vi"("PV Name"="TI-INJ-PROC:getTrig-SR-KICKER") -> ("1rst Value (string)"=w471:string)  [unwired: 8 in, 6 out]
    n259 = Index Array(array=w387, index #1=0 ("index"), index #2=1 ("index"), index #3=2 ("index"), index #4=3 ("index"), index #5=4 ("index"), index #6=5 ("index"), index #7=6 ("index"), index #8=7 ("index"), index #9=8 ("index"), index #10=9 ("index"), index #11=10 ("index"), index #12=11 ("index"), index #13=12 ("index")) -> (element #1=w308:bool, element #2=w307:bool, element #3=w306:bool, element #4=w305:bool, element #5=w304:bool, element #6=w303:bool, element #7=w302:bool, element #8=w301:bool, element #9=w300:bool, element #10=w299:bool, element #11=w298:bool, element #12=w297:bool, element #13=w296:bool)
    n260 = call-poly <userlib>:"CaLabGet.vi"("PV Names"=w378) -> ("1rst Value (number)"=w380:dbl[])  [unwired: 8 in, 6 out]
    n261 = call-poly <userlib>:"CaLabGet.vi"("PV Names"=w379) -> ("1rst Value (number)"=w382:dbl[])  [unwired: 8 in, 6 out]
    n262 = call "FE_PAB_OpenState.vi"("FE"=w207, "XBPMX 2"=w206, "XBPMY 2"=w205, "Hutch"=w204, "PAB"=w203, "MGV"=w202, "FCV"=w201) -> ("XBPMX 2"=w196:string, "XBPMY 2"=w195:string)  [unwired: 7 in]
    n263 = call-poly <userlib>:"CaLabGet.vi"("PV Names"=string[] ["SR-DI-FOFB-H:getStatus", "SR-DI-FOFB-V:getStatus", "IGPF:TPSX:FBCTRL", "IGPF:TPSY:FBCTRL", "TPS-SR-022:bpm3:ilk:enabled_mon", "SR-DI-ANGLE-ILK:StatusX", "SR-DI-ANGLE-ILK:StatusY", "SR-DI-RF-FB:getStatus"]) -> ("1rst Value (string)"=w285:string[], "1rst Value (number)"=w286:dbl[])  [unwired: 8 in, 5 out]
    n264 = Get Date/Time In Seconds() -> (seconds since 1Jan1904=w98:timestamp)
    n265 = call "FE_PAB_OpenState.vi"("FE"=w189, "XBPMX 2"=w200, "XBPMY 2"=w199, "Hutch"=w187, "PAB"=w192, "MGV"=w191, "FCV"=w190) -> ("XBPMX 2"=w194:string, "XBPMY 2"=w193:string)  [unwired: 7 in]
    n266 = Multiply(x=w380, y=w381) -> (x*y=w107:dbl[])
    n267 = To Byte Integer(number=w286) -> (8bit integer=w282:i8[])
    n268 = Multiply(x=w382, y=w381) -> (x*y=w106:dbl[])
    n269 = for {
      tunnel: w282 -> [w856] mode=indexing
      tunnel: [w855] -> w292 mode=indexing
      n270 = case shown="1" w856 {
        tunnel: [TRUE FALSE] -> w855
        frame 1 {
        }
        frame 0, Default {
        }
      }
    }
    n271 = Subtract(x=w97, y=w96) -> (x-y=w103:dbl)
    n272 = Array Max & Min(array=w107) -> (max value=w111:dbl, min value=w110:dbl)  [unwired: 2 out]
    n273 = Array Max & Min(array=w106) -> (max value=w109:dbl, min value=w108:dbl)  [unwired: 2 out]
    n274 = Format Date/Time String(time format string (%c)="%Y%m%d_%H%M%S", seconds (now)=w98) -> (date/time string=w99:string)  [unwired: 1 in]
    n275 = Greater?(x=w103, y=150.0) -> (0:w101:bool)
    n276 = call "FE_PAB_OpenState.vi"("FE"=w188, "XBPMX 2"=w198, "XBPMY 2"=w197, "Hutch"=w186, "PAB"=w185, "MGV"=w184, "FCV"=w183) -> ("XBPMX 2"=w176:string, "XBPMY 2"=w175:string)  [unwired: 7 in]
    n277 = Index Array(array=w285, index #1=0 ("index"), index #2=1 ("index"), index #3=7 ("index")) -> (element #1=w280:string, element #2=w279:string, element #3=w133:string)
    n278 = case shown="True" w101 {
      tunnel: w99 -> [_ w584]
      frame False {
      }
      frame True {
        n279 = flat-sequence {
          tunnel: [w586] -> w585
          tunnel: w584 -> [w586]
          tunnel: w585 -> [w588]
          frame #0 {
            n280 = Wait Until Next ms Multiple(millisecond multiple=u32 32000) -> ()  [unwired: 1 out]
          }
          frame #1 {
            n281 = call "Save_PM_BPM_data.vi"("date_time"=w588) -> ()  [unwired: 11 in]
          }
        }
      }
    }
    n282 = property on="BPMY Graph 2" class="XYGraph (strict)"("YScale.Maximum"=w109, "YScale.Minimum"=w108) -> ()  [unwired: 2 in, 2 out]
    n283 = property on="BPMX Graph 2" class="XYGraph (strict)"("YScale.Maximum"=w111, "YScale.Minimum"=w110) -> ()  [unwired: 2 in, 2 out]
    n284 = call "FE_PAB_OpenState.vi"("FE"=w170, "XBPMX 2"=w166, "XBPMY 2"=w165, "Hutch"=w168, "PAB"=w182, "MGV"=w181, "FCV"=w180) -> ("XBPMX 2"=w174:string, "XBPMY 2"=w173:string)  [unwired: 7 in]
    n285 = call "FE_PAB_OpenState.vi"("FE"=w169, "XBPMX 2"=w164, "XBPMY 2"=w163, "Hutch"=w167, "PAB"=w179, "MGV"=w178, "FCV"=w177) -> ("XBPMX 2"=w172:string, "XBPMY 2"=w171:string)  [unwired: 7 in]
    n286 = Bundle("Array of X axis  平均分配至各段"=w131, w107) -> (w130:cluster{"Array of X axis  平均分配至各段":dbl[], dbl[]})  [unwired: 1 in]
    n287 = Bundle("Array of X axis  平均分配至各段"=w131, w106) -> (w129:cluster{"Array of X axis  平均分配至各段":dbl[], dbl[]})  [unwired: 1 in]
    n288 = Index Array(array=w292, index #1=2 ("index"), index #2=3 ("index"), index #3=4 ("index"), index #4=5 ("index"), index #5=6 ("index")) -> (element #1=w278:bool, element #2=w277:bool, element #3=w276:bool)  [unwired: 2 out]
    n289 = Equal?(x="1" ("1rst Value (string)"), y=w471) -> (x = y?=w469:bool)
    "x = y?" <- w469
    n290 = case shown="True" TRUE {
      tunnel: w138 -> [_ w611]
      frame False {
      }
      frame True {
        n291 = Quit LabVIEW(quit? (T)=w611) -> ()
      }
    }
    n292 = case shown="True" w469 {
      tunnel: w536 -> [_ w884]
      tunnel: w535 -> [_ w883]
      tunnel: [w882 w884] -> w269
      tunnel: [w881 w883] -> w268
      tunnel: w267 -> [w882 _]
      tunnel: w266 -> [w881 _]
      frame False {
      }
      frame True {
        n293 = local read "NOW date"() -> (→"date kickeron":string)
        n294 = local read "NOW time"() -> (→"time kickeron":string)
      }
    }
    n295 = Wait Until Next ms Multiple(millisecond multiple=u32 600) -> ()  [unwired: 1 out]
    n296 = local read "date kickeron"() -> (w275:string)
    n297 = local read "time kickeron"() -> (w274:string)
    n298 = call-poly <userlib>:"CaLabGet.vi"("PV Names"=w162) -> ("1rst Value (string)"=w151:string[])  [unwired: 8 in, 6 out]
    n299 = Index Array(array=w151, index #1=0 ("index"), index #2=1 ("index"), index #3=2 ("index"), index #4=3 ("index"), index #5=4 ("index"), index #6=5 ("index"), index #7=6 ("index"), index #8=7 ("index"), index #9=8 ("index"), index #10=9 ("index")) -> (element #1=w150:string, element #2=w149:string, element #3=w148:string, element #4=w147:string, element #5=w146:string, element #6=w145:string, element #7=w144:string, element #8=w143:string, element #9=w142:string, element #10=w141:string)
    n300 = Bundle By Name(cluster=T1 {"SR Fill Pattern"=[], "Beam Current(mA"=320.769453, "Beam Lifetime(min)"=354.3939151043138, "Beamsize X(um)"=63.15189373514937, "Beamsize Y(um)"=38.03691397287648, "Tune X(from BPM)"=0.1487279843444227, "Tune Y(from BPM)"=0.2309197651663405, "Mode"="Top-Up", "NuX(from BBF) "=0.15142063757609414, "NuY(from BBF)"=0.22496346361412184, "IU22-23gap(R)"=7.0, "IU22-05gap(R)"=7.372, "IU22-05M"=TRUE, "IU22A-09gap(R)"=8.05, "IU22A-09M"=TRUE, "IU22B-09gap(R)"=40.001, "IU22B-09M"=FALSE, "IUT22-21gap(R)"=7.0, "IUT22-21M"=TRUE, "IU22-23M"=TRUE, "IU22A-25gap(R)"=7.0, "IU22A-25M"=TRUE, "IU22B-25gap(R)"=40.0, "IU22B-25M"=FALSE, "EPU48A-41gap(R)"=65.00055, "EPU48A-41gM"=FALSE, "EPU48B-41gap(R)"=27.450000000000003, "EPU48B-41gM"=TRUE, "EPU46-45gap(R)"=44.99850000000001, "EPU46-45gM"=FALSE, "EPU48A-41phase(R)"=0.00055, "EPU48B-41phase(R)"=0.0, "EPU46-45phase(R)"=5e-05, "Grid volt.(V)[S]"=33.0, "Gun mode"="MBM", "Mod.3 HV(kV)[S]"=35.37999999999996, "SR"="SR_DMB_2017_1024_0300LOCO.data", "BR"="Booster_2017_1023_0900.data", "LI"="Linac_2017_0413_1015.data", "LTB"="LTB_JT_2017_0828_1050.data", "BTS"="BTS_2017_1023_0900.data", "RF2 remote"=TRUE, "RF2 OP mode"=TRUE, "RF2 phase.[S]"=-42.0, "RF Freq.(s)"=499655365.67399085, "RF2 gap volt[S]"=1600.0, "RF3 remote"=TRUE, "RF3 OP mode"=TRUE, "RF3 phase.[S]"=1.1999999999999995, "RF3 gap volt.[S]"=1600.0, "BBF V"=TRUE, "BBF H"=TRUE, "BR ext. kicker1(kV)"=17.666, "BR ext. kicker2(kV)"=17.666, "BR ext. sep.1(V)"=322.14, "BR ext. sep.2(V)"=441.1, "BR inj. sep.(V)"=104.95, "BR inj. kicker(kV)"=13.449999999999969, "SR kicker4(kV)"=7.945, "SR kicker3(kV)"=8.02, "SR kicker2(kV)"=8.142, "SR kicker1(kV)"=8.1, "SR inj. sep.2(V)"=397.2, "SR inj. sep.1(V)"=398.04, "Bucket Start"=100.0, "Bucket Last"=450.0, "Bucket Step"=10.0, "Orbit ILK(P)"=TRUE, "IU22-05 Hutch Enable"=TRUE, "IU22A-09M Hutch Enable"=TRUE, "IUT22-21M Hutch Enable"=TRUE, "IU22-23M Hutch Enable"=TRUE, "IU22A-25M Hutch Enable"=TRUE, "EPU48A-41M Hutch Enable"=TRUE, "EPU46-45M Hutch Enable"=FALSE, "EPU46-45 FE Enable"=TRUE, "EPU48A-41 FE Enable"=TRUE, "IU22A-25 FE Enable"=TRUE, "IU22-23 FE Enable"=TRUE, "IUT22-21 FE Enable"=TRUE, "IU22A-09 FE Enable"=TRUE, "IU22-05 FE Enable"=TRUE, "EPU48A-41pM"=FALSE, "EPU48B-41pM"=TRUE, "EPU46-45pM"=FALSE, "Gun volt.(V)[S]"=23.5, "Width count"=75.0, "2ns step"=2.0, "10ps delay"=150.0, "phase shifter"=130.0015, "Taper"=1.0899999999999999, "05XBPMX 1"=14.279, "09XBPMX 1"=-34.837, "21XBPMX 1"=-36.466, "23XBPMX 1"=-38.547000000000004, "25XBPMX 1"=-40.08, "41XBPMX 1"=-513.551, "45XBPMX 1"=-12.86, "05XBPMY 1"=51.999, "09XBPMY 1"=30.004, "21XBPMY 1"=-4.771, "23XBPMY 1"=19.080000000000002, "25XBPMY 1"=-4.366, "41XBPMY 1"=309.241, "45XBPMY 1"=1.842, "FOFB H"="On", "FOFB V"="On", "time string"="15:45:09", "date"="2017/10/28", "date (last kicker ON)"="", "time string (last kicker ON)"="", "Radio Buttons 2"=enum."absolute", "09XBPMX 2"="23.77", "09XBPMY 2"="-18.01", "05XBPMY 2"="-459.85", "05XBPMX 2"="-403.56", "21XBPMY 2"="-134.87", "21XBPMX 2"="-31.92", "23XBPMY 2"="233.82", "23XBPMX 2"="11.09", "25XBPMY 2"="5171.53", "25XBPMX 2"="2152.43", "41XBPMY 2"=" closed", "41XBPMX 2"=" PAB ", "45XBPMX 2"=" Hutch ", "45XBPMY 2"=" closed", "05 mode"="Follow", "09A mode"="Follow", "09B mode"="Follow", "21 mode"="Follow", "23 mode"="Follow", "25A mode"="Follow", "25B mode"="Follow", "41A mode"="Follow", "41B mode"="Follow", "46 mode"="Follow", "BeamCurrent History"={"BPM NO.  1_172"=array[4319 elements], array[4319 elements]}, "SR Beam Current in            hours"=12.0, "RF FB"="On", "gap value："=0, "BR Fill Pattern"=[], "time string (last INJ) "="", "BPMX Graph 2"={"Array of X axis  平均分配至各段"=[1.0, 1.1666666666666667, 1.3333333333333333, 1.5, 1.6666666666666665, 1.8333333333333333, 2.0, 2.142857142857143, 2.2857142857142856, 2.4285714285714284, 2.571428571428571, 2.7142857142857144, 2.857142857142857, 3.0, 3.142857142857143, 3.2857142857142856, 3.4285714285714284, 3.571428571428571, 3.7142857142857144, 3.857142857142857, 4.0, 4.125, 4.25, 4.375, 4.5, 4.625, 4.75, 4.875, 5.0, 5.125, 5.25, 5.375, 5.5, 5.625, 5.75, 5.875, 6.0, 6.142857142857143, 6.285714285714286, 6.428571428571429, 6.571428571428571, 6.714285714285714, 6.857142857142857, 7.0, 7.142857142857143, 7.285714285714286, 7.428571428571429, 7.571428571428571, 7.714285714285714, 7.857142857142857, 8.0, 8.142857142857142, 8.285714285714286, 8.428571428571429, 8.571428571428571, 8.714285714285714, 8.857142857142858, 9.0, 9.142857142857142, 9.285714285714286, 9.428571428571429, 9.571428571428571, 9.714285714285714, 9.857142857142858, 10.0, 10.142857142857142, 10.285714285714286, 10.428571428571429, 10.571428571428571, 10.714285714285714, 10.857142857142858, 11.0, 11.142857142857142, 11.285714285714286, 11.428571428571429, 11.571428571428571, 11.714285714285714, 11.857142857142858, 12.0, 12.125, 12.25, 12.375, 12.5, 12.625, 12.75, 12.875, 13.0, 13.125, 13.25, 13.375, 13.5, 13.625, 13.75, 13.875, 14.0, 14.142857142857142, 14.285714285714286, 14.428571428571429, 14.571428571428571, 14.714285714285714, 14.857142857142858, 15.0, 15.142857142857142, 15.285714285714286, 15.428571428571429, 15.571428571428571, 15.714285714285714, 15.857142857142858, 16.0, 16.142857142857142, 16.285714285714285, 16.428571428571427, 16.571428571428573, 16.714285714285715, 16.857142857142858, 17.0, 17.142857142857142, 17.285714285714285, 17.428571428571427, 17.571428571428573, 17.714285714285715, 17.857142857142858, 18.0, 18.142857142857142, 18.285714285714285, 18.428571428571427, 18.571428571428573, 18.714285714285715, 18.857142857142858, 19.0, 19.142857142857142, 19.285714285714285, 19.428571428571427, 19.571428571428573, 19.714285714285715, 19.857142857142858, 20.0, 20.125, 20.25, 20.375, 20.5, 20.625, 20.75, 20.875, 21.0, 21.125, 21.25, 21.375, 21.5, 21.625, 21.75, 21.875, 22.0, 22.142857142857142, 22.285714285714285, 22.428571428571427, 22.571428571428573, 22.714285714285715, 22.857142857142858, 23.0, 23.142857142857142, 23.285714285714285, 23.428571428571427, 23.571428571428573, 23.714285714285715, 23.857142857142858, 24.0, 24.166666666666668, 24.333333333333332, 24.5, 24.666666666666668, 24.833333333333332], [-104.35000000000001, -27.61, -81.269, 31.074, 6.062, -136.0, 99.494, -88.141, -46.889, -165.06900000000002, 6.021, -84.98, 1.75, -8.811, 8.532, -133.949, -96.848, 24.799, 5.059, -100.301, 144.643, -9.353, 21.271, -55.053000000000004, 53.308, 191.175, 158.868, 222.566, -123.501, -26.869, 534.8770000000001, 573.141, -225.076, -6.779, 120.711, -75.419, 85.256, 50.948, -59.4, -203.09900000000002, -20.847, 130.465, -112.508, 76.115, 15.039, -35.207, -105.659, -16.897000000000002, 68.91, -141.159, 107.378, 144.351, -55.053000000000004, -193.076, 129.21, 58.157000000000004, -162.566, 153.643, 28.149, 9.358, -84.211, 85.112, 22.422, -31.252, 89.379, -47.49, 54.793, -68.275, 110.611, -118.584, -371.90500000000003, -20.115000000000002, -329.103, -249.097, -146.817, 118.556, -25.749, -98.32600000000001, 55.269, -122.093, 50.967, -55.89, 88.019, -0.462, -608.1560000000001, -139.752, -304.999, -215.022, 93.23400000000001, 44.699, -65.235, 37.049, -3.491, -169.852, 216.458, 50.398, -92.285, -132.13400000000001, -12.869, 66.74, -188.53300000000002, 148.653, -5.112, -71.334, -177.681, 41.168, -12.532, -184.913, 194.919, 52.414, -75.628, -80.415, -36.814, 105.73100000000001, -104.36800000000001, 110.101, 49.669000000000004, -67.327, -157.372, 29.624000000000002, 22.156, -105.663, 47.799, 11.591000000000001, -75.285, -79.821, 34.331, -24.937, -158.703, 177.15, 200.872, -165.849, -60.67, 20.183, -15.311, -111.206, 107.58800000000001, 26.489, 69.547, -41.230000000000004, 81.986, 54.43, 253.076, 378.43600000000004, -117.003, -304.999, 131.013, 2.21, -158.435, 94.489, 63.017, -82.94500000000001, 99.147, 65.752, -37.261, -102.577, 41.791000000000004, 66.599, -163.73, 160.137, -7.15, -51.275, -140.353, 33.772, 54.203, -147.597, 128.696, 58.22, -47.144, -184.493, 56.980000000000004, 67.437, -54.227000000000004, -0.031]}, "BPMY Graph 2"={"Array of X axis  平均分配至各段"=[1.0, 1.1666666666666667, 1.3333333333333333, 1.5, 1.6666666666666665, 1.8333333333333333, 2.0, 2.142857142857143, 2.2857142857142856, 2.4285714285714284, 2.571428571428571, 2.7142857142857144, 2.857142857142857, 3.0, 3.142857142857143, 3.2857142857142856, 3.4285714285714284, 3.571428571428571, 3.7142857142857144, 3.857142857142857, 4.0, 4.125, 4.25, 4.375, 4.5, 4.625, 4.75, 4.875, 5.0, 5.125, 5.25, 5.375, 5.5, 5.625, 5.75, 5.875, 6.0, 6.142857142857143, 6.285714285714286, 6.428571428571429, 6.571428571428571, 6.714285714285714, 6.857142857142857, 7.0, 7.142857142857143, 7.285714285714286, 7.428571428571429, 7.571428571428571, 7.714285714285714, 7.857142857142857, 8.0, 8.142857142857142, 8.285714285714286, 8.428571428571429, 8.571428571428571, 8.714285714285714, 8.857142857142858, 9.0, 9.142857142857142, 9.285714285714286, 9.428571428571429, 9.571428571428571, 9.714285714285714, 9.857142857142858, 10.0, 10.142857142857142, 10.285714285714286, 10.428571428571429, 10.571428571428571, 10.714285714285714, 10.857142857142858, 11.0, 11.142857142857142, 11.285714285714286, 11.428571428571429, 11.571428571428571, 11.714285714285714, 11.857142857142858, 12.0, 12.125, 12.25, 12.375, 12.5, 12.625, 12.75, 12.875, 13.0, 13.125, 13.25, 13.375, 13.5, 13.625, 13.75, 13.875, 14.0, 14.142857142857142, 14.285714285714286, 14.428571428571429, 14.571428571428571, 14.714285714285714, 14.857142857142858, 15.0, 15.142857142857142, 15.285714285714286, 15.428571428571429, 15.571428571428571, 15.714285714285714, 15.857142857142858, 16.0, 16.142857142857142, 16.285714285714285, 16.428571428571427, 16.571428571428573, 16.714285714285715, 16.857142857142858, 17.0, 17.142857142857142, 17.285714285714285, 17.428571428571427, 17.571428571428573, 17.714285714285715, 17.857142857142858, 18.0, 18.142857142857142, 18.285714285714285, 18.428571428571427, 18.571428571428573, 18.714285714285715, 18.857142857142858, 19.0, 19.142857142857142, 19.285714285714285, 19.428571428571427, 19.571428571428573, 19.714285714285715, 19.857142857142858, 20.0, 20.125, 20.25, 20.375, 20.5, 20.625, 20.75, 20.875, 21.0, 21.125, 21.25, 21.375, 21.5, 21.625, 21.75, 21.875, 22.0, 22.142857142857142, 22.285714285714285, 22.428571428571427, 22.571428571428573, 22.714285714285715, 22.857142857142858, 23.0, 23.142857142857142, 23.285714285714285, 23.428571428571427, 23.571428571428573, 23.714285714285715, 23.857142857142858, 24.0, 24.166666666666668, 24.333333333333332, 24.5, 24.666666666666668, 24.833333333333332], [-143.858, -13.775, -13.785, 122.665, -66.475, 31.541, 2.118, -24.67, 28.275000000000002, 0.139, -36.578, -28.396, 48.925000000000004, 9.287, -3.412, 70.053, -21.479, 14.89, -7.234, 5.521, -3.164, 19.558, -37.538000000000004, 37.11, -77.159, -13.755, 77.63, 28.249000000000002, -209.114, -44.569, 92.851, 173.641, -70.156, -22.722, 17.795, -6.59, 25.654, -41.882, 53.713, 9.237, -26.164, 18.357, 63.695, -8.542, 5.183, -5.99, 9.508000000000001, -5.462, -29.446, 36.574, -52.552, 51.439, -48.502, 0.73, -23.836000000000002, -3.648, -9.628, -5.485, -68.679, 95.486, -62.041000000000004, 54.633, -58.791000000000004, 68.305, -49.682, 29.838, -8.459, 3.213, -5.561, -80.617, 58.144, 15.346, -158.743, -40.726, 5.259, 3.258, 41.128, -54.377, 5.01, 18.84, 11.403, -20.73, 21.792, -17.296, 27.29, 0.783, -6.804, -137.476, 116.70700000000001, -6.929, 17.846, -3.586, 11.754, 6.341, 0.292, -0.911, -8.236, -5.312, 14.939, -29.945, 30.573, -9.991, -49.344, 82.117, -27.45, 22.291, -6.636, -9.389, 10.034, -14.218, 14.215, -7.3, 12.409, -44.302, 50.197, -36.089, -9.120000000000001, 45.881, 14.836, -27.324, 10.765, -10.139, -33.252, 2.737, -9.99, -6.019, -53.329, -28.159, 2.676, -36.9, -2.372, 8.92, 13.599, -25.723, -16.436, 7.722, -0.088, -29.122, 32.814, -20.521, 30.155, -45.734, 36.611000000000004, 74.528, 68.482, -22.548000000000002, -31.398, 134.603, -45.587, -0.981, -40.156, 24.441, 20.477, -31.424, 19.5, -11.789, 16.394000000000002, -38.567, 9.523, 0.09, -0.058, -4.8500000000000005, 11.71, 25.637, -10.51, -18.101, -12.389000000000001, 95.417, -138.726, 30.355, 96.245, -48.666000000000004, 40.851, -0.71]}} ("Cluster"), "Tune X(from BPM)"=w269, "Tune Y(from BPM)"=w268, "date (last kicker ON)"=w275, "time string (last kicker ON)"=w274, "date"=w90, "time string"=w295, "Mode"=w376, "Beam Current(mA"=w96, "Beam Lifetime(min)"=w375, "Beamsize X(um)"=w374, "Beamsize Y(um)"=w373, "NuX(from BBF)"=w372, "NuY(from BBF)"=w371, "Bucket Start"=w370, "Bucket Last"=w369, "Bucket Step"=w368, "BR inj. sep.(V)"=w367, "BR inj. kicker(kV)"=w366, "BR ext. kicker1(kV)"=w365, "BR ext. kicker2(kV)"=w364, "BR ext. sep.1(V)"=w363, "BR ext. sep.2(V)"=w362, "SR inj. sep.1(V)"=w361, "SR inj. sep.2(V)"=w360, "SR kicker1(kV)"=w359, "SR kicker2(kV)"=w358, "SR kicker3(kV)"=w357, "SR kicker4(kV)"=w356, "Gun mode"=w355, "Grid volt.(V)[S]"=w354, "Gun volt.(V)[S]"=w353, "Mod.3 HV(kV)[S]"=w352, "Width count"=w351, "2ns step"=w350, "10ps delay"=w349, "RF2 remote"=w348, "RF2 OP mode"=w347, "RF2 phase.[S]"=w273, "RF Freq.(s)"=w346, "RF2 gap volt[S]"=w272, "RF3 remote"=w345, "RF3 OP mode"=w344, "RF3 phase.[S]"=w343, "RF3 gap volt.[S]"=w342, "BR"=w341, "BTS"=w340, "LI"=w338, "LTB"=w337, "SR"=w339, "SR Fill Pattern"=w95, "IU22-05 Hutch Enable"=w224, "IU22A-09M Hutch Enable"=w220, "IUT22-21M Hutch Enable"=w204, "IU22-23M Hutch Enable"=w187, "IU22A-25M Hutch Enable"=w186, "EPU48A-41M Hutch Enable"=w168, "EPU46-45M Hutch Enable"=w167, "EPU46-45 FE Enable"=w169, "EPU48A-41 FE Enable"=w170, "IU22A-25 FE Enable"=w188, "IU22-23 FE Enable"=w189, "IUT22-21 FE Enable"=w207, "IU22A-09 FE Enable"=w219, "IU22-05 FE Enable"=w225, "IU22-05gap(R)"=w336, "IU22A-09gap(R)"=w335, "IU22B-09gap(R)"=w334, "IUT22-21gap(R)"=w333, "IU22-23gap(R)"=w332, "IU22A-25gap(R)"=w331, "IU22B-25gap(R)"=w330, "EPU48A-41gap(R)"=w329, "EPU48A-41phase(R)"=w328, "EPU48B-41gap(R)"=w327, "EPU48B-41phase(R)"=w326, "EPU46-45gap(R)"=w325, "EPU46-45phase(R)"=w324, "Taper"=w270, "phase shifter"=w323, "05XBPMX 1"=w322, "09XBPMX 1"=w321, "21XBPMX 1"=w320, "23XBPMX 1"=w319, "25XBPMX 1"=w318, "41XBPMX 1"=w317, "45XBPMX 1"=w316, "05XBPMY 1"=w315, "09XBPMY 1"=w314, "21XBPMY 1"=w313, "23XBPMY 1"=w312, "25XBPMY 1"=w311, "41XBPMY 1"=w310, "45XBPMY 1"=w309, "IU22-05M"=w308, "IU22A-09M"=w307, "IU22B-09M"=w306, "IUT22-21M"=w305, "IU22-23M"=w304, "IU22A-25M"=w303, "IU22B-25M"=w302, "EPU48A-41gM"=w301, "EPU48B-41gM"=w300, "EPU46-45gM"=w299, "EPU48A-41pM"=w298, "EPU48B-41pM"=w297, "EPU46-45pM"=w296, "BPMX Graph 2"=w130, "BPMY Graph 2"=w129, "Radio Buttons 2"=enum32{"absolute", "different with"}."absolute", "FOFB H"=w280, "FOFB V"=w279, "BBF H"=w278, "BBF V"=w277, "Orbit ILK(P)"=w276, "05XBPMX 2"=w214, "05XBPMY 2"=w213, "09XBPMX 2"=w212, "09XBPMY 2"=w211, "21XBPMX 2"=w196, "21XBPMY 2"=w195, "23XBPMX 2"=w194, "23XBPMY 2"=w193, "25XBPMX 2"=w176, "25XBPMY 2"=w175, "41XBPMX 2"=w174, "41XBPMY 2"=w173, "45XBPMX 2"=w172, "45XBPMY 2"=w171, "05 mode"=w150, "09A mode"=w149, "09B mode"=w148, "21 mode"=w147, "23 mode"=w146, "25A mode"=w145, "25B mode"=w144, "41A mode"=w143, "41B mode"=w142, "46 mode"=w141, "BeamCurrent History"=w137, "RF FB"=w133, "gap value："=w124, "BR Fill Pattern"=w114, "time string (last INJ)"=w112) -> (→"Cluster":T1)
  }
  n301 = List Folder(path=w20) -> (filenames=w16:string[])  [unwired: 3 in, 3 out]
  n302 = Index Array(array=w16, index=w17) -> (element=w15:string)
  n303 = Build Path(base path=w20, name or relative path=w15) -> (appended path=w14:path)
  "appended path" <- w14
  n304 = while {
    tunnel: w33 -> [_]
    shift-right: [w917] -> _
    shift-left: string[] [] -> [w914]
    shift-right: [w905] -> _
    shift-left: string[][] [] -> [w908]
    tunnel: w41 -> [w911]
    i -> [w909]
    stop <- w910 stop-if-true
    w902 = 1000  # limit
    # "為了使檯面上記憶體不要使用太多而做的筆數限制"
    n305 = flat-sequence {
      tunnel: [w961] -> w918
      tunnel: [w960] -> w915
      tunnel: w914 -> [w960]
      tunnel: [w959] -> w912
      tunnel: w911 -> [w959]
      tunnel: [w971] -> w919
      tunnel: w918 -> [w971]
      tunnel: [w969] -> w916
      tunnel: w915 -> [w970]
      tunnel: [w963] -> w913
      tunnel: w912 -> [w962]
      tunnel: w919 -> [w994]
      tunnel: [w992] -> w917
      tunnel: w916 -> [w992]
      tunnel: w913 -> [w991]
      tunnel: [w991] -> w900
      frame #0 {
        n306 = Tick Count (ms)() -> (millisecond timer value=w961:u32)
      }
      frame #1 {
        n307 = Get Date/Time In Seconds() -> (seconds since 1Jan1904=w966:timestamp)
        n308 = To Double Precision Float(number=w966) -> (double precision float=w965:dbl)
        n309 = Format Date/Time String(time format string (%c)="%Y/%m/%d %H:%M:%S", seconds (now)=w966) -> (date/time string=w967:string)  [unwired: 1 in]
        n310 = Number To Fractional String(number=w965) -> (F-format string=w964:string)  [unwired: 3 in]
        n311 = call-poly <userlib>:"CaLabGet.vi"("PV Names"=w962) -> ("1rst Value (string)"=w969:string[])  [unwired: 8 in, 6 out]
        n312 = for {
          tunnel: w970 -> [w973] mode=indexing
          tunnel: w969 -> [w972] mode=indexing
          tunnel: w962 -> [w981] mode=indexing
          tunnel: w967 -> [w980]
          tunnel: [w979] -> w963 mode=indexing if=w977
          tunnel: w964 -> [w978]
          i -> [w976]
          n313 = Greater Or Equal?(x=w976, y=1) -> (x >= y?=w974:bool)
          n314 = case shown="True" w974 {
            tunnel: w981 -> [_ w990]
            tunnel: w973 -> [_ w989]
            tunnel: w972 -> [_ w988]
            tunnel: w980 -> [_ w987]
            tunnel: [string[] [] w986] -> w979
            tunnel: w978 -> [_ w985]
            tunnel: [FALSE w984] -> w977
            frame False {
            }
            frame True {
              n315 = Not Equal?(x=w989, y=w988) -> (x != y?=w984:bool)
              n316 = Build Array(w987, w990, w989, w988, w985) -> (w986:string[])
            }
          }
        }
      }
      frame #2 {
        n317 = Tick Count (ms)() -> (millisecond timer value=w995:u32)
        n318 = Subtract(x=w995, y=w994) -> (x-y=→"dT":u32)
      }
    }
    n319 = while {
      i -> [w952]
      stop <- w956 stop-if-true
      # "每60秒，表示法:\n100 600"
      # "每十秒，表示法:\n100 100"
      n320 = local read "stop"() -> (w955:bool)
      n321 = Multiply(x="Check period", y=10) -> (x*y=w953:i32)
      n322 = Greater Or Equal?(x=w952, y=w953) -> (x >= y?=w957:bool)
      n323 = Wait Until Next ms Multiple(millisecond multiple=u32 99) -> ()  [unwired: 1 out]
      n324 = Or(x=w957, y=w955) -> (x .or. y?=w956:bool)
    }
    n325 = Array Size(array=w908) -> (size(s)=w907:i32[])
    n326 = Build Array (concatenate)(w908, w900) -> (w904:string[][])
    n327 = Index Array(array=w907, index=0) -> (element=w903:i32)
    "EVENTs" <- w903
    n328 = Greater Or Equal?(x=w903, y=w902) -> (x >= y?=w901:bool)
    n329 = case shown="True" w901 {
      selector: w901 -> [_ w921]
      tunnel: w904 -> [w920 w938]
      tunnel: [w920 w942] -> w905
      tunnel: w903 -> [_ w933]
      tunnel: w902 -> [_ w932]
      frame False {
      }
      frame True {
        n330 = call "Main_Daily_path.vi"("nothing"=w921) -> ("Directory path"=w929:path)  [unwired: 9 in, 1 out]
        n331 = Build Path(base path=w929, name or relative path="Association\\" ("string")) -> (appended path=w925:path)
        n332 = call <vilib>:"Check if File or Folder Exists.vi"("path"=w925) -> ("error out"=w926:errorcluster, "file or folder exists?"=w928:bool, "dup path"=w927:path)  [unwired: 8 in]
        n333 = case shown="False" w928 {
          tunnel: w927 -> [w948 w949]
          tunnel: [w947 w950] -> _
          tunnel: w926 -> [w946 w950]
          tunnel: [w945 w949] -> w924
          frame False {
            n334 = Create Folder(path (use dialog)=w948, error in=w946) -> (created path=w945:path, error out=w947:errorcluster)  [unwired: 1 in, 1 out]
          }
          frame True {
          }
        }
        n335 = Array Subset(array=w938, index (row)=0 ("index"), length (row)=w932, index (col)=0 ("index"), length (col)=5 ("length")) -> (w937:string[][])
        n336 = Subtract(x=w933, y=w932) -> (x-y=w931:i32)
        n337 = Build Path(base path=w924, name or relative path="changedPVsBKUPov1k.csv" ("string")) -> (appended path=w923:path)
        n338 = call-poly <vilib>:"Write To Spreadsheet File.vi"("delimiter (\\t)"="," ("delimiter (\\t)"), "transpose? (no:F)"=FALSE, "append to file? (new file:F)"=TRUE, "2D data"=w937, "file path (dialog if empty)"=w923) -> ()  [unwired: 3 in, 1 out]
        n339 = Array Subset "Array Subset"(array=w938, index (row)=w932, length (row)=w931, index (col)=0 ("index"), length (col)=5 ("length")) -> (w942:string[][])
      }
    }
    "Diff list" <- w905
    n340 = local read "stop"() -> (w910:bool)
    "check loop" <- w909
  }
  n341 = Path To String(path=w14) -> (string=w2:string)
  n342 = property class="IWMPPlayer4"(reference="WindowsMediaPlayer", "enabled"=TRUE, "uiMode"="invisible") -> (reference out=w13:refnum<k7>, error out=w6:errorcluster, "settings"=w10:refnum<k7>, "controls"=w19:refnum<k7>)  [unwired: 1 in]
  n343 = property on="new picture" class="Pict"("Visible"=TRUE) -> ()  [unwired: 2 in, 2 out]
  n344 = property class="IWMPSettings"(reference=w10, error in=w6, "autoStart"=FALSE) -> (error out=w4:errorcluster, "volume"=w11:i32)  [unwired: 1 out]
  n345 = local write "Vol."(w11) -> ()
  n346 = property class="IWMPPlayer4"(reference=w13, error in=w4, "URL"=w2) -> (reference out=w18:refnum<k7>, error out=→"error out 2":errorcluster)
  n347 = while {
    tunnel: w18 -> [w998]
    tunnel: w19 -> [w1003]
    tunnel: w20 -> [w1000]
    stop <- w996 stop-if-true
    n348 = flat-sequence {
      tunnel: w998 -> [w1008]
      tunnel: [w1008] -> w997
      frame #0 {
        n349 = Wait (ms)(milliseconds to wait=u32 300 ("millisecond multiple")) -> ()  [unwired: 1 out]
      }
    }
    n350 = property class="IWMPPlayer4"(reference=w997) -> (reference out=w1001:refnum<k7>, error out=w999:errorcluster, "status"=w1007:string)  [unwired: 1 in]
    "status" <- w1007
    n351 = local read "Play Button"() -> (w1004:bool)
    n352 = Equal?(x=w1007, y="已停止") -> (x = y?=w1005:bool)
    n353 = And(x=w1005, y=w1004) -> (x .and. y?=w1002:bool)
    n354 = case shown="True" w1002 {
      tunnel: w1003 -> [_ w1025]
      tunnel: w1001 -> [_ w1014]
      tunnel: w1000 -> [_ w1013]
      tunnel: w999 -> [_ w1010]
      frame False {
      }
      frame True {
        n355 = local read "index"() -> (w1016:i32)
        n356 = List Folder(path=w1013) -> (filenames=w1017:string[])  [unwired: 3 in, 3 out]
        n357 = Increment(x=w1016) -> (x+1=w1015:i32)
        n358 = Array Size(array=w1017) -> (size(s)=w1023:i32)
        n359 = Decrement(x=w1023) -> (x-1=w1024:i32)
        n360 = Greater?(x=w1015, y=w1024) -> (0:w1018:bool)
        n361 = Select(t=0, s=w1018, f=w1015) -> (s? t:f=w1011:i32)
        n362 = Index Array(array=w1017, index=w1011) -> (element=w1020:string)
        n363 = Build Path(base path=w1013, name or relative path=w1020) -> (appended path=w1021:path)
        n364 = Path To String(path=w1021) -> (string=w1022:string)
        n365 = property class="IWMPPlayer4"(reference=w1014, error in=w1010, "URL"=w1022) -> (error out=w1012:errorcluster)  [unwired: 1 out]
        n366 = local write "index"(w1011) -> ()
        n367 = invoke class="IWMPControls" method="play"(reference=w1025, error in=w1012) -> ()  [unwired: 1 in, 3 out]
      }
    }
    n368 = local read "stop"() -> (w996:bool)
  }
  n369 = while {
    tunnel: w19 -> [w1033]
    tunnel: [w1032] -> w5
    tunnel: w10 -> [w1031]
    shift-right: [w1027] -> _
    shift-left: w17 -> [w1030]
    tunnel: w20 -> [w1029]
    tunnel: w18 -> [w1028]
    stop <- w1026 stop-if-true
    n370 = event shown="[0] \"Play Button\": Value Change" {
      selector: _ -> [_ _ _ _ _]
      dyn-events: _ -> [_ _ _ _ _]
      timeout: _ -> [_ _ _ _ _]
      tunnel: w1033 -> [w1036 w1039 w1046 w1060 _]
      tunnel: [w1035 w1038 _ _ _] -> w1032
      tunnel: w1031 -> [_ _ _ _ w1076]
      tunnel: w1030 -> [w1034 w1037 w1058 w1073 w1075]
      tunnel: w1029 -> [_ _ w1052 w1066 _]
      tunnel: w1028 -> [_ _ w1059 w1074 _]
      tunnel: [w1034 w1037 w1053 w1068 w1075] -> w1027
      event "Play Button": Value Change {
        n371 = event-data() -> ()  [unwired: 1 in, 1 out]
        n372 = invoke class="IWMPControls" method="play"(reference=w1036) -> (error out=w1035:errorcluster)  [unwired: 2 in, 2 out]
      }
      event "Pause Button": Value Change {
        n373 = event-data() -> ("NewVal"=w1040:bool)  [unwired: 1 in]
        n374 = case shown="False" w1040 {
          tunnel: w1039 -> [w1041 w1044]
          tunnel: [w1042 w1043] -> w1038
          frame False {
            n375 = invoke class="IWMPControls" method="play"(reference=w1041) -> (error out=w1042:errorcluster)  [unwired: 2 in, 2 out]
          }
          frame True {
            n376 = invoke class="IWMPControls" method="pause"(reference=w1044) -> (error out=w1043:errorcluster)  [unwired: 2 in, 2 out]
          }
        }
      }
      event "Skip Forward Button": Value Change {
        n377 = event-data() -> ()  [unwired: 1 in, 1 out]
        n378 = List Folder(path=w1052) -> (filenames=w1057:string[])  [unwired: 3 in, 3 out]
        n379 = Increment(x=w1058) -> (x+1=w1055:i32)
        n380 = Array Size(array=w1057) -> (size(s)=w1048:i32)
        n381 = Decrement(x=w1048) -> (x-1=w1047:i32)
        n382 = Greater?(x=w1055, y=w1047) -> (0:w1056:bool)
        n383 = Select(t=0, s=w1056, f=w1055) -> (s? t:f=w1053:i32)
        n384 = Index Array(array=w1057, index=w1053) -> (element=w1051:string)
        n385 = Build Path(base path=w1052, name or relative path=w1051) -> (appended path=w1050:path)
        n386 = Path To String(path=w1050) -> (string=w1049:string)
        n387 = property class="IWMPPlayer4"(reference=w1059, "URL"=w1049) -> (error out=w1045:errorcluster)  [unwired: 1 in, 1 out]
        n388 = invoke class="IWMPControls" method="play"(reference=w1046, error in=w1045) -> ()  [unwired: 1 in, 3 out]
      }
      event "Skip Back Button": Value Change {
        n389 = event-data() -> ()  [unwired: 1 in, 1 out]
        n390 = List Folder(path=w1066) -> (filenames=w1072:string[])  [unwired: 3 in, 3 out]
        n391 = Decrement(x=w1073) -> (x-1=w1070:i32)
        n392 = Array Size(array=w1072) -> (size(s)=w1063:i32)
        n393 = Decrement(x=w1063) -> (x-1=w1062:i32)
        n394 = Less?(x=w1070, y=0) -> (x < y?=w1071:bool)
        n395 = Select(t=w1062, s=w1071, f=w1070) -> (s? t:f=w1068:i32)
        n396 = Index Array(array=w1072, index=w1068) -> (element=w1064:string)
        n397 = Build Path(base path=w1066, name or relative path=w1064) -> (appended path=w1067:path)
        n398 = Path To String(path=w1067) -> (string=w1065:string)
        n399 = property class="IWMPPlayer4"(reference=w1074, "URL"=w1065) -> (error out=w1061:errorcluster)  [unwired: 1 in, 1 out]
        n400 = invoke class="IWMPControls" method="play"(reference=w1060, error in=w1061) -> ()  [unwired: 1 in, 3 out]
      }
      event "Vol.": Value Change {
        n401 = event-data() -> ()  [unwired: 1 in, 1 out]
        n402 = property class="IWMPSettings"(reference=w1076, "volume"="Vol.") -> ()  [unwired: 1 in, 2 out]
      }
    }
    "index" <- w1027
    n403 = local read "stop"() -> (w1026:bool)
  }
  n404 = local write "stop"(FALSE ("stop")) -> ()
  n405 = invoke class="IWMPPlayer4" method="close"(reference=w18, error in=w5) -> ()  [unwired: 1 in, 3 out]
  n406 = disable-structure shown="Disabled" {
    frame Disabled {
      (unwired) string[] ["LI-VA-VAL-01:STA:POS", "LI-VA-VAL-02:STA:POS", "LI-VA-VAL-03:STA:POS", "LI-VA-VAL-04:STA:POS", "LI-VA-VAL-05:STA:POS"]
      # "VALVE(EPICS)"
    }
    frame Enabled {
    }
  }
  n407 = disable-structure shown="Disabled" {
    frame Disabled {
    }
    frame Enabled {
    }
  }
